vi "Main.vi"() -> ()   [LabVIEW 2018]
uses:
  <vilib>/picture/picture.llb/imagedata.ctl
  <vilib>/Utility/miscctls.llb/LVPoint32TypeDef.ctl
  <vilib>/Utility/miscctls.llb/LVMouseTypeDef.ctl
  <vilib>/Utility/miscctls.llb/LVPositionTypeDef.ctl
  <vilib>/Utility/miscctls.llb/LVPointTypeDef.ctl
  <vilib>/Utility/miscctls.llb/LVRectTypeDef.ctl
  Shared Variables/Alarm Cluster (UI).ctl
  Shared Variables/Alarm Cluster.ctl
  Drag and Drop/State Cluster.ctl
  support/Message Queue/Message Cluster.ctl
  Drag and Drop/Thumbnail Cluster.ctl
  Drag and Drop/Object Cluster.ctl
  Drag and Drop/Object Type Enum.ctl
  Config Module/Controls/Main Config Cluster.ctl
  OPC/OPC Module Config.ctl
  Scale Module Folder/Measure Instrument/State Enum.ctl
  OPC/OPC Settings.ctl
  OPC/Variable Data Cluster.ctl
  <vilib>/OPCUA/controls/NodeId.ctl
  <vilib>/OPCUA/controls/OPC UA StatusCode.ctl
  <vilib>/OPCUA/controls/Subscription ID.ctl
  <vilib>/OPCUA/controls/OPC UA Client Refnum.ctl
  <vilib>/OPCUA/controls/Subscription Data Change.ctl
  <vilib>/OPCUA/controls/Data Type.ctl
  Feed Module/Controls/Feed Module Config Cluster.ctl
  Feed Module/Controls/Feed Module Settings Cluster.ctl
  Ismatec ISM 831C/Controls/Ismatech Settings Cluster.ctl
  Masterflex 7550-30/Controls/Settings Cluster.ctl
  Mettler Toledo/Controls/Settings Cluster.ctl
  Bronkhorst M13 Flow Meter/Settings Cluster.ctl
  Measure Instrument/PID 2 Parameters Cluster.ctl
  Measure Instrument/PID Input Enum.ctl
  Measure Instrument/PID 2 Output Enum.ctl
  Tacmina QI/Tacmina QI DAQ Setting.ctl
  KNF Pump/Settings Cluster plus SIMDOS.ctl
  ASIA Pump/Pump Settings.ctl
  VICI M50 Party Mode/Settings Cluster.ctl
  FLOM Pump/Settings Cluster.ctl
  SSI PR Class/SSI PR or LD Settings Cluster.ctl
  Masterflex 75211/Masterflex 75211 DAQ Setting.ctl
  SSI PR Class/SSI P40 Settings Cluster.ctl
  TT Module/Controls/TT Module Config Cluster.ctl
  Tag VIs/Numeric Alarm Settings Cluster.ctl
  Acquisition/Hardware Configuration.ctl
  Acquisition/Task Cluster.ctl
  PT Module/Controls/PT Module Config Cluster.ctl
  Scale Module Folder/Feed Module/Controls/Scale Module Config Cluster.ctl
  Scale Module Folder/Feed Module/Controls/Scale Module Settings Cluster.ctl
  Pump Module Folder/Pump Module Config Cluster.ctl
  Pump Module Folder/Pump Module Settings Cluster.ctl
  LabJack Module/Controls/U3 Module Config Cluster.ctl
  Decoration Module/Decoration Module Config Cluster.ctl
  Flow Module Folder/Feed Module/Controls/Flow Module Config Cluster.ctl
  Flow Module Folder/Feed Module/Controls/Flow Module Settings Cluster.ctl
  TCU Module/TCU Module Folder/TCU Module Config Cluster.ctl
  TCU Module/TCU Module Folder/TCU Module Settings Cluster.ctl
  TCU Module/TCU Module Folder/Measure Instrument/Output Devices.ctl
  Huber TCU/Huber Settings.ctl
  Lauda Integral XT-150 TCU/Lauda Settings.ctl
  Julabo Type 1 TCU/Julabo Type 1 TCU Folder/Julabo FP-50 Settings.ctl
  Huber Unistat 410 TCU/Huber Unistat 410 RS485 Settings.ctl
  D-O Module Folder/Not Sure Where this is Used.ctl
  Sequencing/Squence Control.ctl
  D-O Module Folder/D-O Module Config Cluster.ctl
  D-O Module Folder/Valve Clusters.ctl
  D-O Module Folder/D-O Module Settings Cluster.ctl
  D-O Module Folder/D-O Device Settings Cluster.ctl
  VICI Electronic Actuator/VICI Electronic Actuator Settings.ctl
  Pressure Regulator Control Module/Pressure Regulator/Controls/4-20mA Module Config Cluster.ctl
  Pressure Regulator Control Module/Pressure Regulator/Controls/4-20mA Module Settings Cluster.ctl
  Pressure Transmitter/Pressure Transmitter Device Settings.ctl
  Pressure Reg Module/Pressure Regulator Device Settings.ctl
  Tag VIs/Tag FGV Operation Enum.ctl
  Shared Variables/Alarm Log Operation Enum.ctl
  Drag and Drop/Drop Parameters Cluster.ctl
  Drag and Drop/Module Instance Number Operation Enum.ctl
  Drag and Drop/Module Type Enum.ctl
  <vilib>/Utility/error.llb/DialogType.ctl
  Config Module/Controls/Config File Operation Enum.ctl
  Waveform Loop/Start Params Cluster.ctl
  Pump Calibration Program/Pump Calibration Config.ctl
  support/Message Queue/Enqueue Message (Single).vi
  <vilib>/Utility/cursorutil.llb/Set Cursor (Icon Pict).vi
  Main/Main Globals.vi
  LabJack Module/U3 (Main).vit
  D-O Module Folder/D-O Module (Main).vi
  TCU Module/TCU Module Folder/TCU Module (Main).vi
  Flow Module Folder/Flow Module (Main).vi
  <vilib>/Utility/cursorutil.llb/Set Cursor (Cursor ID).vi
  support/Message Queue/Message Queue.lvlib
  support/User Event - Stop/User Event - Stop.lvlib
  support/Support Library.lvlib
  Drag and Drop/Drag and Drop.lvlib
  Feed Module/Feed Module.lvlib
  TT Module/TT Module.lvlib
  History Graph/History Graph.lvlib
  Waveform Loop/Waveform Loop.lvlib
  CSV Log/CSV Log.lvlib
  TDMS Log/TDMS Log.lvlib
  Shared Variables/Dynamic Shared Variables.lvlib
  DAQ/DAQ.lvlib
  Config Module/Config Module.lvlib
  Bronkhorst M13 Flow Meter/Bronkhorst M13 Flow Meter.lvlib
  Mettler Toledo/Mettler Toledo.lvlib
  Masterflex 7550-30/Masterflex 7550-30.lvlib
  Ismatec ISM 831C/Ismatec ISM 831C.lvlib
  PT Module/PT Module.lvlib
  Scale Module Folder/Scale Module.lvlib
  Pump Module Folder/Pump Module.lvlib
  <vilib>/lvdsc/NI_DSC.lvlib
  LabJack Module/U3 Module.lvlib
  Flow Module Folder/Flow Module.lvlib
  Tacmina QI/Tacmina QI.lvlib
  KNF Pump/KNF SIMDOS.lvlib
  Huber TCU/Huber Ministat 230 TCU.lvlib
  TCU Module/TCU Module Folder/TCU Module.lvlib
  Lauda Integral XT-150 TCU/Lauda TCU.lvlib
  Julabo Type 1 TCU/Julabo Type 1 TCU Folder/Julabo Type FP-50 TCU.lvlib
  ASIA Pump.lvlib
  Sequencing/Sequencing Library.lvlib
  VICI M50 Party Mode/VICI M6 M50 Party Mode.lvlib
  D-O Module Folder/D-O Module.lvlib
  Pressure Regulator Control Module/Pressure Regulator/4-20mA Module.lvlib
  Pressure Reg Module/Pressure Regulator Library.lvlib
  Pressure Transmitter/Pressure Transmitter Library.lvlib
  FLOM Pump/FLOM Pump.lvlib
  support/Command Log VIs/Command Logging.lvlib
  Calibration VIs/Calibration.lvlib
  Lauda Integral XT-150 TCU/TCP Library.lvlib
  SSI PR Class/SSI PR or LD Pump.lvlib
  Scale Module Folder/Measure Instrument/Scale Module Engine.lvlib
  OPC/OPC UA.lvlib
  D-O Module Folder/DIO Valve/VICI Electronic Actuator.lvlib
  subVIs/Main SubVIs.lvlib
  Masterflex 75211/Masterflex 75211.lvlib
  SSI PR Class/SSI P40 Pump.lvlib
  Huber Unistat 410 TCU/Huber Unistat 410 TCU.lvlib
panel:
  out "Cluster":T1 {"Main Config"."PR Module Configs"."Settings"."PID 2 Parameters"."output range"."output low" format="%.2f"; "Main Config"."PR Module Configs"."Settings"."PID 2 Parameters"."output range"."output high" min=0.0 max=100.0 format="%.2f"; "Main Config"."PR Module Configs"."Settings"."PID 2 Parameters"."PID gains"."derivative time (Td, min)" format="%.3f"; "Main Config"."PR Module Configs"."Settings"."PID 2 Parameters"."PID gains"."integral time (Ti, min)" format="%.3f"; "Main Config"."PR Module Configs"."Settings"."PID 2 Parameters"."PID gains"."proportional gain (Kc)" format="%.3f"; "Main Config"."Steps"."Control" items=["Pump %", "Setpoint"]; "Main Config"."TCU Module Configs"."Settings"."Huber Unistat 410 Settings"."Address" min=0 max=99 format="%02.0f"; "Main Config"."TCU Module Configs"."Settings"."Julabo FP-50 Settings"."Pump Power" min=0 max=8 step=1; "Main Config"."TCU Module Configs"."Settings"."Lauda Settings"."Pump Power" min=0 max=8 step=1; "Main Config"."Pump Module Configs"."Settings"."ASIA Pump C"."channel" min=0 max=1 step=1; "Main Config"."Pump Module Configs"."Settings"."Masterflex"."Pump Number" min=1.0 max=20.0 step=1.0; "Main Config"."Pump Module Configs"."Settings"."Ismatech"."Pump Number" min=1.0 max=20.0 step=1.0; "Main Config"."Feed Module Configs"."Settings"."output range"."output low" min=0.0 max=100.0 format="%.2f"; "Main Config"."Feed Module Configs"."Settings"."output range"."output high" format="%.2f"; "Main Config"."Feed Module Configs"."Settings"."PID 2 Parameters"."PID gains"."derivative time (Td, min)" format="%.3f"; "Main Config"."Feed Module Configs"."Settings"."PID 2 Parameters"."PID gains"."integral time (Ti, min)" format="%.3f"; "Main Config"."Feed Module Configs"."Settings"."PID 2 Parameters"."PID gains"."proportional gain (Kc)" format="%.3f"; "Main Config"."Feed Module Configs"."Settings"."ASIA Pump C"."channel" min=0 max=1 step=1; "Main Config"."Feed Module Configs"."Settings"."Ismatech"."Pump Number" min=1.0 max=20.0 step=1.0; "Main Config"."Feed Module Configs"."Settings"."Masterflex"."Pump Number" min=1.0 max=20.0 step=1.0}
  in  "Alarm History Button":bool
  out "Alarm Model":T65[](array[typedef]) {"Alarm"."value" format="%.2f"; "Alarm"."setpoint" format="%.2f"; "Alarm"."clear time" format="%<%X\n%x>T"; "Alarm"."ack time" format="%<%X\n%x>T"; "Alarm"."set time" format="%<%X\n%x>T"}
  in  "UI Alarms":T66[](array[typedef])
  out "Message Data":variant
  out "data":errorcluster
  in  "End Program":bool
  out "CSV Log File":path
  out "error out":errorcluster
  in  "E-Stop":bool
  out "x-y":T4
  out "Front Panel Window:Panel Bounds":T4
  out "Drop Offset":T6
  out "Origin":T67
  out "Position":T6
  out "output cluster":cluster{"Coords":T10, "Mouse":T68}
  out "Mouse Position":cluster{"X":i32, "Y":i32}
  out "Path":path
  out "index of element":i32
  out "image data":T69
  in  "Page":string="Batch"
  in  "Notebook":string="Test"
  in  "Exit":bool
  in  "Settings":bool
  in  "Pause Log Button":bool
  in  "Force Trigger":bool
  in  "Start Log":bool
  out "Canvas":picture
  out "Palette":picture
  in  "?":T1 {"Main Config"."PR Module Configs"."Settings"."PID 2 Parameters"."output range"."output low" format="%.2f"; "Main Config"."PR Module Configs"."Settings"."PID 2 Parameters"."output range"."output high" min=0.0 max=100.0 format="%.2f"; "Main Config"."PR Module Configs"."Settings"."PID 2 Parameters"."PID gains"."derivative time (Td, min)" format="%.3f"; "Main Config"."PR Module Configs"."Settings"."PID 2 Parameters"."PID gains"."integral time (Ti, min)" format="%.3f"; "Main Config"."PR Module Configs"."Settings"."PID 2 Parameters"."PID gains"."proportional gain (Kc)" format="%.3f"; "Main Config"."Steps"."Control" items=["Pump %", "Setpoint"]; "Main Config"."TCU Module Configs"."Settings"."Huber Unistat 410 Settings"."Address" min=0 max=99 format="%02.0f"; "Main Config"."TCU Module Configs"."Settings"."Julabo FP-50 Settings"."Pump Power" min=0 max=8 step=1; "Main Config"."TCU Module Configs"."Settings"."Lauda Settings"."Pump Power" min=0 max=8 step=1; "Main Config"."Pump Module Configs"."Settings"."ASIA Pump C"."channel" min=0 max=1 step=1; "Main Config"."Pump Module Configs"."Settings"."Masterflex"."Pump Number" min=1.0 max=20.0 step=1.0; "Main Config"."Pump Module Configs"."Settings"."Ismatech"."Pump Number" min=1.0 max=20.0 step=1.0; "Main Config"."Feed Module Configs"."Settings"."output range"."output low" min=0.0 max=100.0 format="%.2f"; "Main Config"."Feed Module Configs"."Settings"."output range"."output high" format="%.2f"; "Main Config"."Feed Module Configs"."Settings"."PID 2 Parameters"."PID gains"."derivative time (Td, min)" format="%.3f"; "Main Config"."Feed Module Configs"."Settings"."PID 2 Parameters"."PID gains"."integral time (Ti, min)" format="%.3f"; "Main Config"."Feed Module Configs"."Settings"."PID 2 Parameters"."PID gains"."proportional gain (Kc)" format="%.3f"; "Main Config"."Feed Module Configs"."Settings"."ASIA Pump C"."channel" min=0 max=1 step=1; "Main Config"."Feed Module Configs"."Settings"."Ismatech"."Pump Number" min=1.0 max=20.0 step=1.0; "Main Config"."Feed Module Configs"."Settings"."Masterflex"."Pump Number" min=1.0 max=20.0 step=1.0}
  # "little pump\ncentrifigual pump\nflow rate\npressure\nS or P to the left\nsolvent or process"
  # "Question: how do we make the live VI, such as the feed module graphic\nsized right for the picture that is loaded?\n\nProbably should standarize each module size. Then the  flow sheet\ndrawings will all just match the size and we don't have to worry about\nscale."
  # "vertical or horizontal lines\nextendable"
  # "Tasks\n1. Load graphic\n2. Drag and drop onto picture control\n3. Picture control draws hot spot\n4. If drag and drop on picture control, then resize and redraw the nearest hotspot\n5. When operator turns \"ON\" the system, then the hotspots are replaced with actual VIs."
  # "as much drawing room as possible"
  # "Instrument Settings"
  # "Instrument Settings"
  # "Output Instruments"
  # "Flow Meter Settings"
  # "Output Instruments"
  # "Scale Settings"
  # "Output Instruments"
  # "Input Instruments"
  # "Instrument Settings"
  # "Instrument Settings"
  # "Output Instruments"
  # "Flow Meter Settings"
  # "Output Instruments"
  # "Scale Settings"
  # "Output Instruments"
  # "Input Instruments"
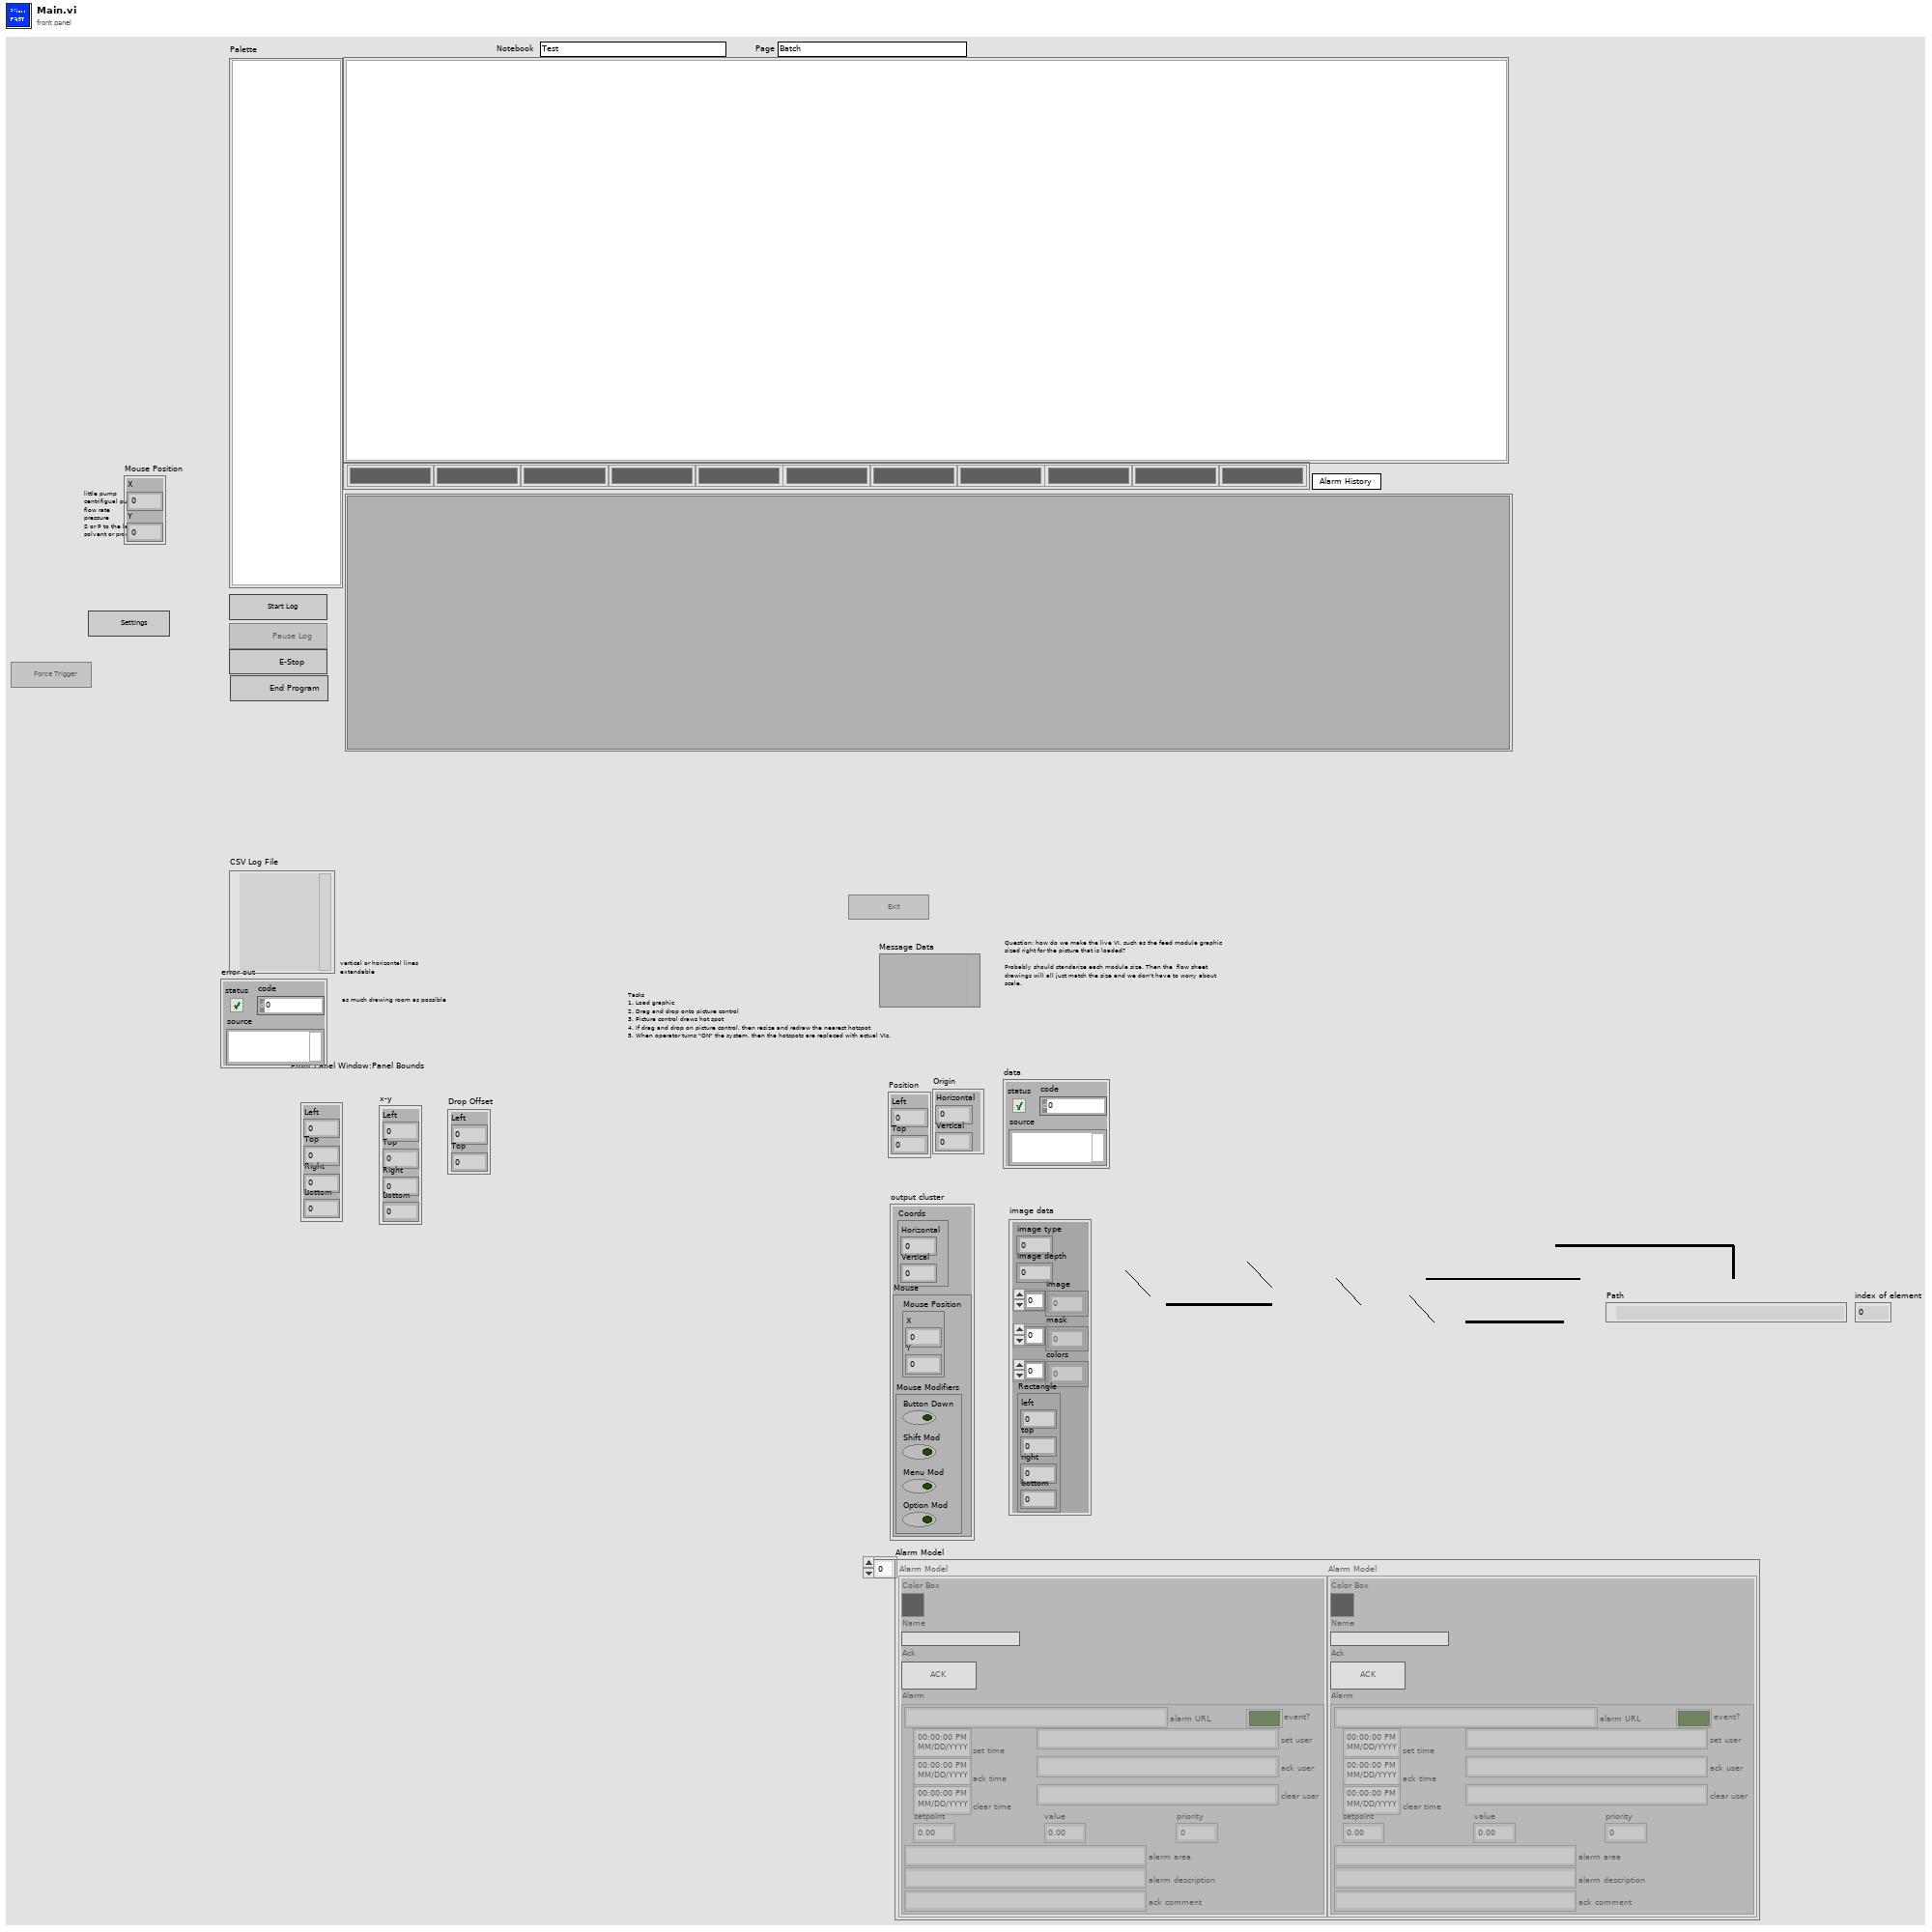
[diagram p1: front panel]
types:
  T1 = typedef "Drag and Drop.lvlib/State Cluster.ctl" = cluster{"VI refs":refnum<vi>[], "Queues":refnum<queue>[], "[Thumbnails]":T2[], "Drag Object Idx":i32, "[Objects]":T3[], "Active Object":i32, "Drop Offset":T6, "Process Name":string, "Main Config":T7, "Campaign Filepath":path, "Config Changed?":bool}
  T2 = typedef "Thumbnail Cluster.ctl" = cluster{"Path":path, "Rectangle":cluster{"left":i16, "top":i16, "right":i16, "bottom":i16}}
  T3 = typedef "Object Cluster.ctl" = cluster{"BMP Path":path, "Anchor Position":cluster{"X":i32, "Y":i32}, "Hot Spot":T4, "Type":T5, "Parameters":variant}
  T4 = typedef "LVRectTypeDef.ctl" = cluster{"Left":i16, "Top":i16, "Right":i16, "Bottom":i16}
  T5 = typedef "Object Type Enum.ctl" = enum16{"Icon", "Line", "Text", "Feed Module"}
  T6 = typedef "LVPositionTypeDef.ctl" = cluster{"Left":i32, "Top":i32}
  T7 = typedef "Config Module.lvlib/Main Config Cluster.ctl" = cluster{"Notebook":string, "Page":string, "OPC Module Configs":T8[], "Feed Module Configs":T17[], "Log File Path":path, "TT Module Configs":T34[], "DAQ Config":T36, "PT Module Configs":T38[], "Scale Module Configs":T39[], "Pump Module Configs":T41[], "U3 Module Configs":T43[], "Decoration Module Configs":T44[], "Flow Module Configs":T45[], "TCU Module Configs":T47[], "Steps":T54, "Abort":bool, "DO Module Configs":T56[], "PR Module Configs":T61[], "Cycle Period":dbl}
  T8 = typedef "OPC UA.lvlib/OPC Module Config.ctl" = cluster{"State":T9, "GUID":string, "Drop Coords":T10, "Configuration":T11, "First Iteration":bool, "Data":cluster{"Object Name":string, "Variable Array":T12[]}[], "Process Name":string, "Load Count":i32, "Log Started":bool, "subscription ID out":T15, "OPC UA client refnum out":T16, "Event Registration Refnum":refnum<event-registration>, "Start Time":timestamp, "Current Time":timestamp}
  T9 = typedef "Scale Module.lvlib/Scale Module Engine.lvlib/State Enum.ctl" = enum16{"Measuring", "Idle"}
  T10 = typedef "LVPoint32TypeDef.ctl" = cluster{"Horizontal":i32, "Vertical":i32}
  T11 = typedef "OPC UA.lvlib/OPC Settings.ctl" = cluster{"Cycle Period":dbl, "server endpoint URL":string, "security policy":cluster{"message mode":enum16{"None", "Sign", "Sign and Encrypt"}, "security":enum16{"Basic256", "Basic128Rsa15"}}, "Trust Any Server":bool}
  T12 = typedef "OPC UA.lvlib/Variable Data Cluster.ctl" = cluster{"node ID":T13, "browse name":string, "status":T14, "timestamp":timestamp, "value ":variant}
  T13 = typedef "NodeId.ctl" = string
  T14 = typedef "OPC UA StatusCode.ctl" = u32
  T15 = typedef "Subscription ID.ctl" = u32
  T16 = typedef "OPC UA Client Refnum.ctl" = refnum<k21>
  T17 = typedef "Feed Module.lvlib/Feed Module Config Cluster.ctl" = cluster{"GUID":string, "Drop Coords":T10, "Process Name":string, "Queue Name":string, "Settings":T18, "Settings Load Count":i32, "OP Load Count":i32}
  T18 = typedef "Feed Module.lvlib/Feed Module Settings Cluster.ctl" = cluster{"Cycle Period":dbl, "Ismatech":T19, "Masterflex":T20, "Mettler":T21, "Bronkhorst M13 Flow Meter":T22, "PID 2 Parameters":T23, "Manual Entry":dbl, "Auto?":bool, "output range":cluster{"output high":dbl, "output low":dbl}, "Bronkhorst M14":T21, "Tacmina Settings":T26, "KNF SIMDOS Settings":T27, "ASIA Pump C":T28, "VICI Settings":T29, "FLOM Settings":T30, "SSI PR/LD Settings":T31, "Masterflex 75211 Settings":T32, "SSI P40 Settings":T33}
  T19 = typedef "Ismatec ISM 831C.lvlib/Ismatech Settings Cluster.ctl" = cluster{"VISA resource name":refnum<visa-resource-name>, "Simulated?":bool, "Pump Number":dbl, "Reverse?":bool}
  T20 = typedef "Masterflex 7550-30.lvlib/Settings Cluster.ctl" = cluster{"VISA resource name":refnum<visa-resource-name>, "Simulated?":bool, "Pump Number":dbl, "Reverse?":bool}
  T21 = typedef "Mettler Toledo.lvlib/Settings Cluster.ctl" = cluster{"VISA resource name":refnum<visa-resource-name>, "Simulated?":bool}
  T22 = typedef "Bronkhorst M13 Flow Meter.lvlib/Settings Cluster.ctl" = cluster{"VISA resource name":refnum<visa-resource-name>, "Simulated?":bool}
  T23 = typedef "PID 2 Parameters Cluster.ctl" = cluster{"Input Device":T24, "Output Device":T25, "Setpoint":dbl, "PID gains":cluster{"proportional gain (Kc)":dbl, "integral time (Ti, min)":dbl, "derivative time (Td, min)":dbl}}
  T24 = typedef "PID Input Enum.ctl" = enum16{"Default", "Bronkhorst M13", "Bronkhorst M14", "Scale Rate of Change"}
  T25 = typedef "PID 2 Output Enum.ctl" = enum16{"Default", "Ismatec ISM 831C", "Masterflex 7550-30", "VICI", "Tacmina QI", "KNF SIMDOS", "ASIA Type C", "FLOM UI-22-11", "SSI PR/LD", "SSI P40", "Masterflex 75211-70"}
  T26 = typedef "Tacmina QI.lvlib/Tacmina QI DAQ Setting.ctl" = cluster{"Analog DAQ Task":refnum<k21>, "Digital DAQ Task":refnum<k21>}
  T27 = typedef "KNF SIMDOS.lvlib/Settings Cluster plus SIMDOS.ctl" = cluster{"VISA resource name":refnum<visa-resource-name>, "Simulated?":bool}
  T28 = typedef "ASIA Pump.lvlib/Pump Settings.ctl" = cluster{"ASIA Pump #":i32, "channel":i32, "Simulated":bool}
  T29 = typedef "VICI M6 M50 Party Mode.lvlib/Settings Cluster.ctl" = cluster{"VISA resource name":refnum<visa-resource-name>, "Simulated?":bool, "Pump Letter":string, "Reverse?":bool}
  T30 = typedef "FLOM Pump.lvlib/Settings Cluster.ctl" = cluster{"VISA resource name":refnum<visa-resource-name>, "Simulated?":bool, "Pump Number":dbl}
  T31 = typedef "SSI PR or LD Pump.lvlib/SSI PR or LD Settings Cluster.ctl" = cluster{"VISA resource name":refnum<visa-resource-name>, "Simulated?":bool}
  T32 = typedef "Masterflex 75211.lvlib/Masterflex 75211 DAQ Setting.ctl" = cluster{"Analog DAQ Task":refnum<k21>, "Digital DAQ Task":refnum<k21>}
  T33 = typedef "SSI P40 Pump.lvlib/SSI P40 Settings Cluster.ctl" = cluster{"VISA resource name":refnum<visa-resource-name>, "Simulated?":bool}
  T34 = typedef "TT Module.lvlib/TT Module Config Cluster.ctl" = cluster{"GUID":string, "Drop Coords":T10, "Input Channel Tag Name ":string, "Process Name":string, "Queue Name":string, "Input Channel Numeric Alarm Settings":T35[]}
  T35 = typedef "Numeric Alarm Settings Cluster.ctl" = cluster{"enable? (F)":bool, "name":string, "alarm type":enum16{"HI_HI", "HI", "LO", "LO_LO"}, "level/change":dbl, "deadband/time":dbl, "alarm delay":dbl, "priority":u32, "ack type":enum16{"Auto", "User", "None", "Each Occurrence"}, "area":string, "description":string, "log? (T)":bool}
  T36 = typedef "DAQ.lvlib/Hardware Configuration.ctl" = cluster{"Tasks":T37[]}
  T37 = typedef "Task Cluster.ctl" = cluster{"DAQmx Task":refnum<k21>, "Read-Write Radio":enum32{"Read", "Write"}}
  T38 = typedef "PT Module.lvlib/PT Module Config Cluster.ctl" = cluster{"GUID":string, "Drop Coords":T10, "Input Channel Tag Name ":string, "Process Name":string, "Queue Name":string, "Input Channel Numeric Alarm Settings":T35[]}
  T39 = typedef "Scale Module.lvlib/Scale Module Config Cluster.ctl" = cluster{"GUID":string, "Drop Coords":T10, "Process Name":string, "Queue Name":string, "Settings":T40, "Load Count":i32}
  T40 = typedef "Scale Module.lvlib/Scale Module Settings Cluster.ctl" = cluster{"Cycle Period":dbl, "Mettler":T21, "Scale Type":string}
  T41 = typedef "Pump Module.lvlib/Pump Module Config Cluster.ctl" = cluster{"GUID":string, "Drop Coords":T10, "Process Name":string, "Queue Name":string, "Settings":T42, "Load Count":i32}
  T42 = typedef "Pump Module.lvlib/Pump Module Settings Cluster.ctl" = cluster{"Cycle Period":dbl, "Manual Entry":dbl, "Output Device":T25, "Ismatech":T19, "Masterflex":T20, "VICI Settings":T29, "Tacmina Settings":T26, "KNF SIMDOS Settings":T27, "ASIA Pump C":T28, "FLOM Settings":T30, "SSI PR/LD Settings":T31, "SSI P40 Settings":T31, "Masterflex 75211 Settings":T32, "Pump Calibration File":path, "Calibration Slope":dbl, "Calibration Y Intercept":dbl, "Pump Cal Enum":u16}
  T43 = typedef "U3 Module.lvlib/U3 Module Config Cluster.ctl" = cluster{"GUID":string, "Drop Coords":T10, "AI Channel Number":enum16{"Default", "AI0", "AI1", "AI2", "AI3", "AI4", "AI5", "AI6", "AI7"}, "Process Name":string, "Queue Name":string, "Input Channel Numeric Alarm Settings":T35[]}
  T44 = typedef "Decoration Module Config Cluster.ctl" = cluster{"GUID":string, "Drop Coords":T10, "Decoration Filepath":path}
  T45 = typedef "Flow Module.lvlib/Flow Module Config Cluster.ctl" = cluster{"GUID":string, "Drop Coords":T10, "Process Name":string, "Queue Name":string, "Settings":T46, "Load Count":i32}
  T46 = typedef "Flow Module.lvlib/Flow Module Settings Cluster.ctl" = cluster{"Cycle Period":dbl, "Bronkhorst M13":T21, "Flow Meter Type":string, "Bronkhorst M14":T21}
  T47 = typedef "TCU Module.lvlib/TCU Module Config Cluster.ctl" = cluster{"GUID":string, "Drop Coords":T10, "Process Name":string, "Queue Name":string, "Settings":T48, "Load Count":i32, "Power Level Changed":bool}
  T48 = typedef "TCU Module.lvlib/TCU Module Settings Cluster.ctl" = cluster{"Cycle Period":dbl, "Setpoint Entry":dbl, "Output Device":T49, "Huber Ministat 230 Settings":T50, "Lauda Settings":T51, "Julabo FP-50 Settings":T52, "Internal Control?":bool, "Huber Unistat 410 Settings":T53}
  T49 = typedef "Output Devices.ctl" = enum16{"Default", "Huber Ministat 230", "Huber Unistat 410", "Lauda XT-150", "Julabo FP-50"}
  T50 = typedef "Huber Ministat 230 TCU.lvlib/Huber Settings.ctl" = cluster{"VISA resource name":refnum<visa-resource-name>, "Simulated?":bool}
  T51 = typedef "Lauda TCU.lvlib/Lauda Settings.ctl" = cluster{"VISA resource name":refnum<visa-resource-name>, "Simulated?":bool, "Pump Power":i32}
  T52 = typedef "Julabo Type FP-50 TCU.lvlib/Julabo FP-50 Settings.ctl" = cluster{"VISA resource name":refnum<visa-resource-name>, "Simulated?":bool, "Pump Power":i32}
  T53 = typedef "Huber Unistat 410 TCU.lvlib/Huber Unistat 410 RS485 Settings.ctl" = cluster{"VISA resource name":refnum<visa-resource-name>, "Address":i8, "Simulated?":bool}
  T54 = typedef "Not Sure Where this is Used.ctl" = T55[]
  T55 = typedef "Sequencing Library.lvlib/Squence Control.ctl" = cluster{"Module":string, "Control":u16, "Value":dbl, "Wait (sec)":dbl}
  T56 = typedef "D-O Module.lvlib/D-O Module Config Cluster.ctl" = cluster{"GUID":string, "Drop Coords":T10, "Process Name":string, "Queue Name":string, "Settings":T57, "Load Count":i32}
  T57 = typedef "D-O Module.lvlib/Valve Clusters.ctl" = cluster{"Valve Settings":T58, "Valve Type":enum16{"Default", "Digital Output Valve", "VICI Electronic Actuator"}, "Time On (Sec)":dbl, "Time Off (Sec)":dbl, "Run?":bool}
  T58 = typedef "D-O Module.lvlib/D-O Module Settings Cluster.ctl" = cluster{"D-O Settings":T59, "VICI Electronic Actuator":T60}
  T59 = typedef "D-O Module.lvlib/D-O Device Settings Cluster.ctl" = cluster{"DAQmx Task Name":refnum<k21>, "Output Channel":u16, "Output Channel Names":string[]}
  T60 = typedef "VICI Electronic Actuator.lvlib/VICI Electronic Actuator Settings.ctl" = cluster{"VISA resource name":refnum<visa-resource-name>, "Mode":enum16{"Two Positions With Stops", "Two Positions Without Stops", "Mutiposition"}, "Simulated":bool}
  T61 = typedef "4-20mA Module.lvlib/4-20mA Module Config Cluster.ctl" = cluster{"GUID":string, "Drop Coords":T10, "Process Name":string, "Queue Name":string, "Settings":T62, "Settings Load Count":i32}
  T62 = typedef "4-20mA Module.lvlib/4-20mA Module Settings Cluster.ctl" = cluster{"Cycle Period":dbl, "PID 2 Parameters":cluster{"Input Device":enum16{"Default", "4-20mA"}, "Output Device":enum16{"Default", "Equilibar Pressure Reg", "Flow Regulator"}, "Setpoint":dbl, "PID gains":cluster{"proportional gain (Kc)":dbl, "integral time (Ti, min)":dbl, "derivative time (Td, min)":dbl}, "output range":cluster{"output low":dbl, "output high":dbl}}, "Manual Entry":dbl, "Auto?":bool, "4-20mA Input Settings":T63, "4-20mA Out Settings":T64, "Input Channel Tag Name ":string}
  T63 = typedef "Pressure Transmitter Library.lvlib/Pressure Transmitter Device Settings.ctl" = cluster{"Input Channel ":u16}
  T64 = typedef "Pressure Regulator Library.lvlib/Pressure Regulator Device Settings.ctl" = cluster{"Output DAQ Task":refnum<k21>}
  T65 = typedef "Dynamic Shared Variables.lvlib/Alarm Cluster.ctl" = cluster{"Color Box":u32, "Name":string, "Ack":bool, "Alarm":cluster{"alarm URL":string, "set time":timestamp, "set user":string, "ack time":timestamp, "ack user":string, "clear time":timestamp, "clear user":string, "setpoint":dbl, "value":dbl, "priority":u32, "alarm area":string, "alarm description":string, "ack comment":string, "event?":bool, "Refnum":u64}}
  T66 = typedef "Dynamic Shared Variables.lvlib/Alarm Cluster (UI).ctl" = cluster{"Color Box":u32, "Name":string, "Ack":bool}
  T67 = typedef "LVPointTypeDef.ctl" = cluster{"Horizontal":i16, "Vertical":i16}
  T68 = typedef "LVMouseTypeDef.ctl" = cluster{"Mouse Position":cluster{"X":i32, "Y":i32}, "Mouse Modifiers":cluster{"Button Down":bool, "Shift Mod":bool, "Menu Mod":bool, "Option Mod":bool}}
  T69 = typedef "imagedata.ctl" = cluster{"image type":i32, "image depth":i32, "image":u8[], "mask":u8[], "colors":u32[], "Rectangle":cluster{"left":i16, "top":i16, "right":i16, "bottom":i16}}
  T70 = typedef "Tag FGV Operation Enum.ctl" = enum16{"Init", "Set Notification Queue", "Create Tag", "Commit", "Write Tag (Numeric)", "Write Tag (Boolean)", "Read All Tags", "Read One Tag", "Delete Tag Category", "Set Alarm Parameters (Numeric)", "Set Alarm Parameters (Boolean)", "Enable All Alarms", "Disable All Alarms", "Delete All Tags", "Read Alarms", "Ack Alarm", "Read Alarm Parameters (Numeric)", "Read Alarm Parameters (Boolean)"}
  T71 = cluster{"Down":bool, "Mouse":T68, "Drag":bool, "Canvas":bool}
  T72 = cluster{"Busy":bool, "PumpCnt":dbl, "RemoteEntered":bool, "OverpressureSet":bool}[]
  T73 = typedef "Main Queue Cluster.ctl" = cluster{"UI":refnum<queue>, "Waveform Loop":refnum<queue>, "CSV Log":refnum<queue>, "TDMS Log":refnum<queue>, "Graphs":refnum<queue>[], "DAQ":refnum<queue>, "Sequence":refnum<queue>, "TCP Write":refnum<queue>, "Sequence UI":refnum<queue>, "OPC UA Log":refnum<queue>, "TCP Read":refnum<queue>}
  T74 = cluster{"Event Registration Refnum":refnum<event-registration>, "Stop Event Registration Refnum":refnum<event-registration>}
  T75 = typedef "Alarm Log Operation Enum.ctl" = enum16{"Create Log", "Log Alarm", "Close Log"}
  T76 = enum32{"Invalid", "Standard", "Closed", "Hidden", "Minimized", "Maximized"}
  T77 = enum8{"Enabled", "Disabled", "Disabled and Grayed Out"}
  T78 = cluster{"alarm URL":string, "set time":timestamp, "set user":string, "ack time":timestamp, "ack user":string, "clear time":timestamp, "clear user":string, "setpoint":dbl, "value":dbl, "priority":u32, "alarm area":string, "alarm description":string, "ack comment":string, "event?":bool, "Refnum":u64}[]
  T79 = cluster{"alarm URL":string, "set time":timestamp, "set user":string, "ack time":timestamp, "ack user":string, "clear time":timestamp, "clear user":string, "setpoint":dbl, "value":dbl, "priority":u32, "alarm area":string, "alarm description":string, "ack comment":string, "event?":bool, "Refnum":u64}
  T80 = typedef "Drag and Drop.lvlib/Module Type Enum.ctl" = enum16{"<unknown module>", "Feed", "TT", "PT", "Scale", "Flow", "Pump", "U3", "TCU", "DO", "PR", "OPC"}
  T81 = typedef "Module Instance Number Operation Enum.ctl" = enum16{"Init", "Next Instance Number"}
  T82 = typedef "Drop Parameters Cluster.ctl" = cluster{"Module VI Filepath":path, "Process Name":string, "Main UI Message Queue":refnum<queue>, "Drop Coords":T10, "Module Parameters":variant, "Name of Parent Window":string}
  T83 = typedef "Config Module.lvlib/Config File Operation Enum.ctl" = enum16{"Read", "Write"}
  T84 = typedef "Waveform Loop.lvlib/Start Params Cluster.ctl" = cluster{"dt (seconds)":dbl, "CSV Logfile path":path, "TDMS Logfile path":path}
  T85 = typedef "Calibration.lvlib/Pump Calibration Config.ctl" = cluster{"Settings":cluster{"Cycle Period":dbl, "Ismatech":T19, "Masterflex":T20, "Bronkhorst M13 Flow Meter":T22, "PID 2 Parameters":cluster{"Input Device":T24, "Output Device":T25}, "Bronkhorst M14":T21, "Tacmina Settings":T26, "KNF SIMDOS Settings":T27, "VICI M50 Settings":T29, "FLOM Settings":T30, "Calibration Limits":cluster{"Minimum (ml/min)":dbl, "Maximum (ml/min)":dbl, "Steps":dbl}, "SSI PR Settings":T31}, "Flowmeter Output":dbl, "Density":dbl, "FL Temp":dbl, "Speed %":dbl, "File Refnum":refnum<file>, "Pump On?":enum16{"Off", "On", "Not Initialized"}}
  T86 = typedef "DialogType.ctl" = u16
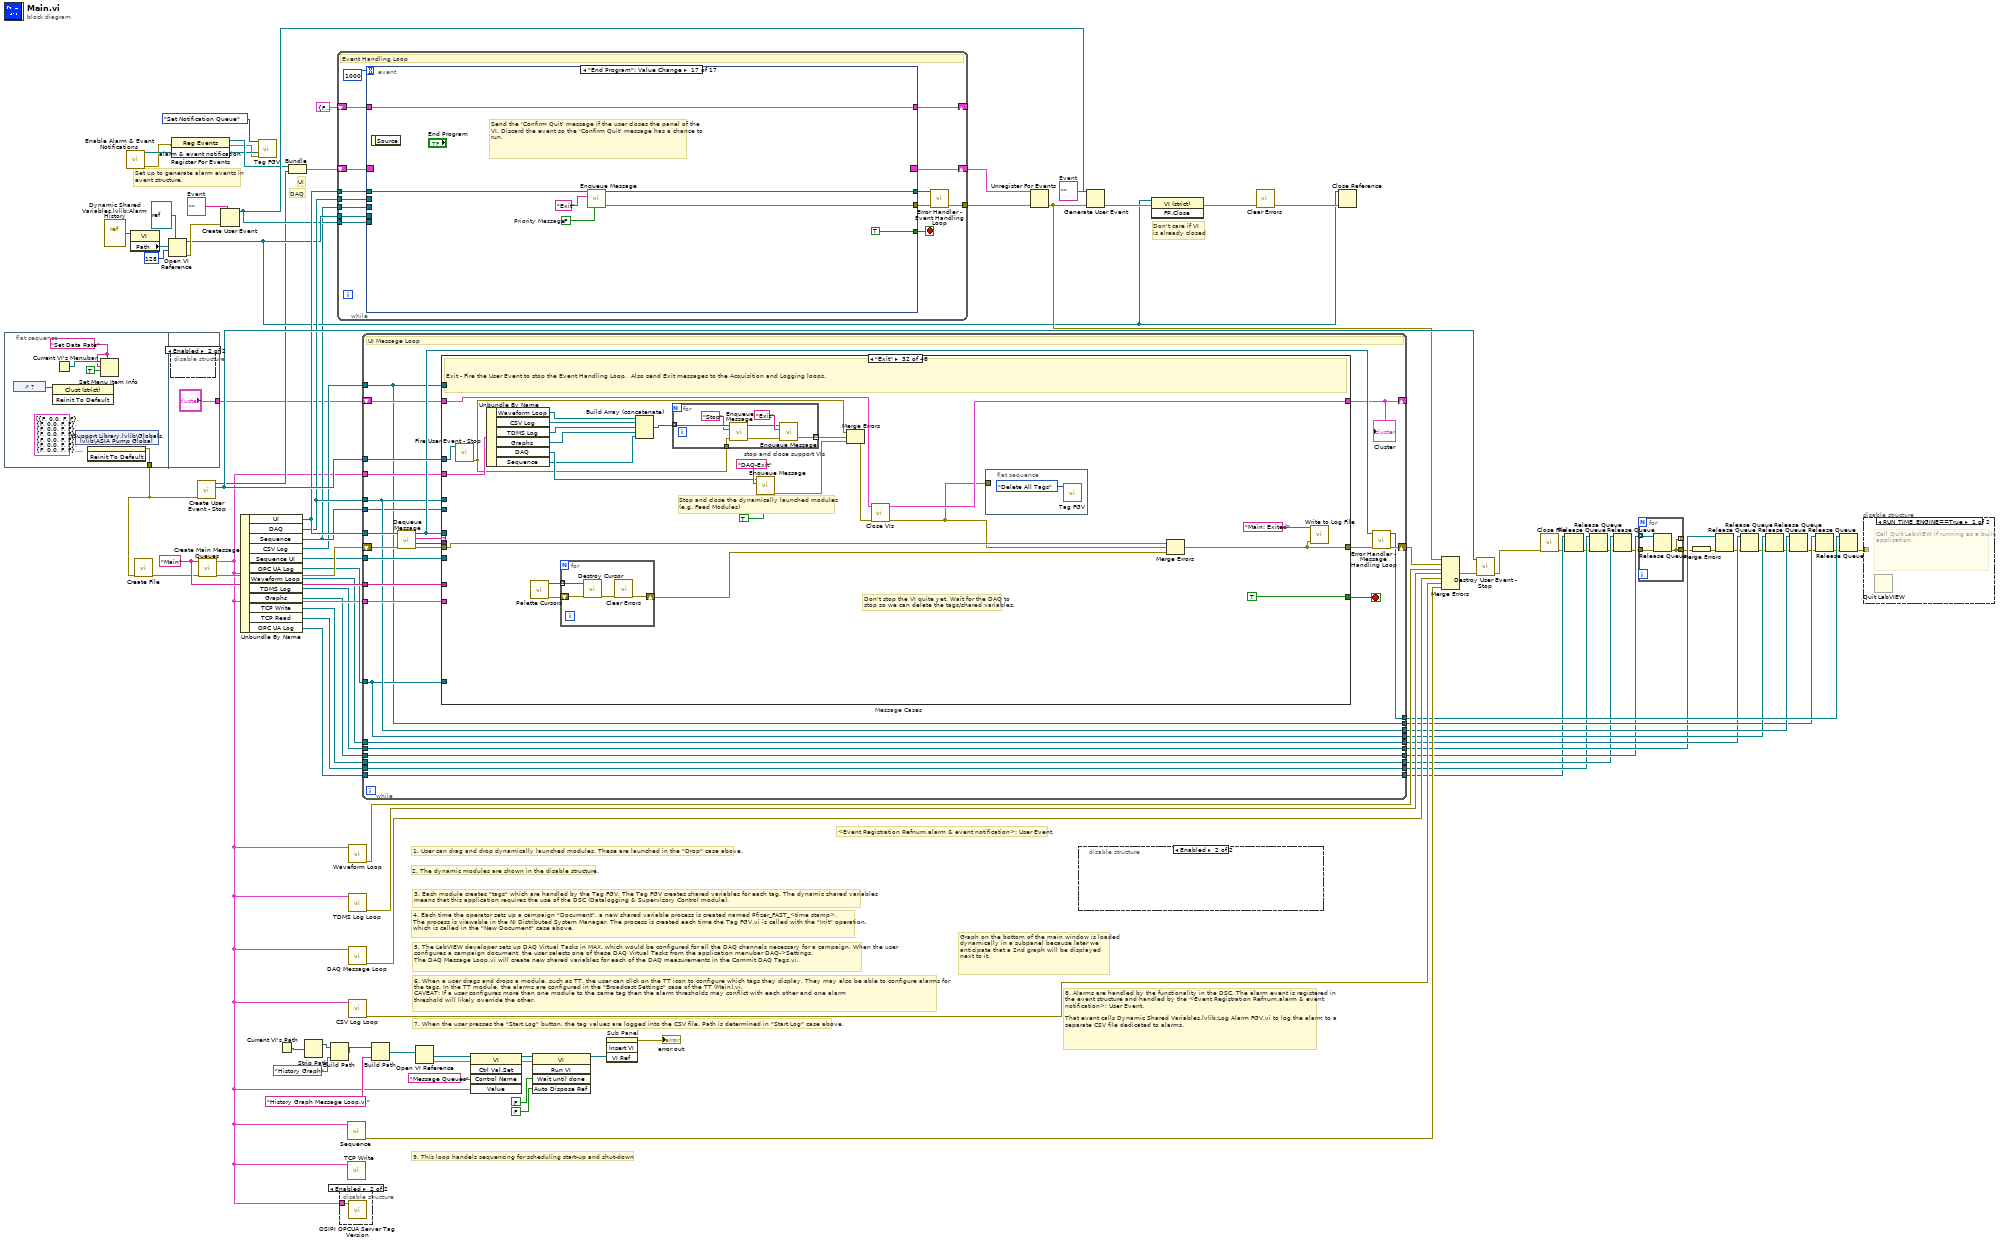
[diagram p0: block diagram]
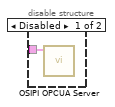
[diagram p2: hidden frame]
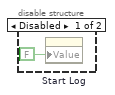
[diagram p3: hidden frame]
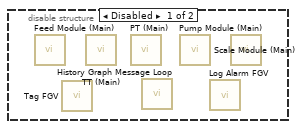
[diagram p5: hidden frame]
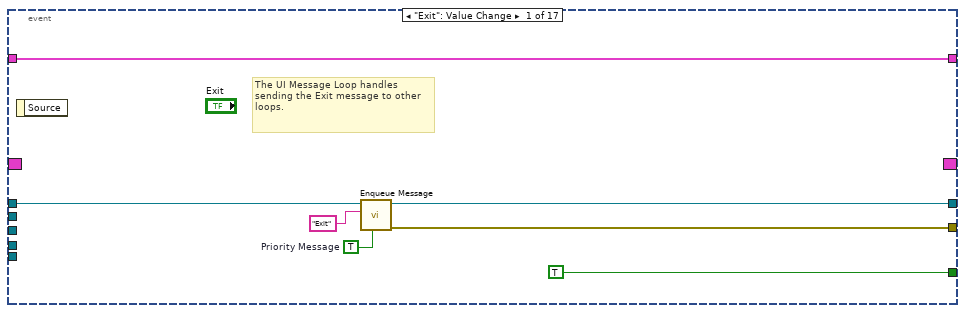
[diagram p6: hidden frame]
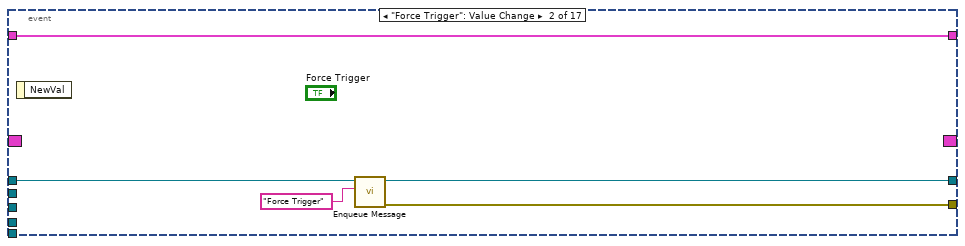
[diagram p7: hidden frame]
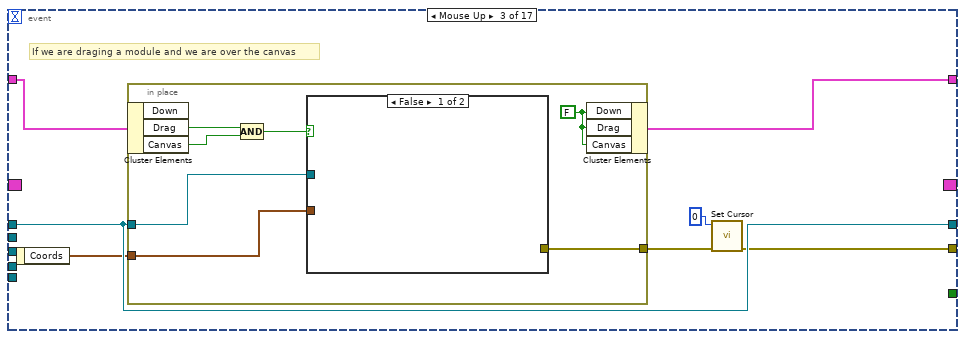
[diagram p8: hidden frame]
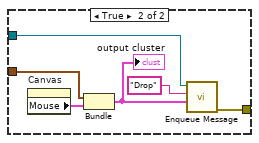
[diagram p9: hidden frame]
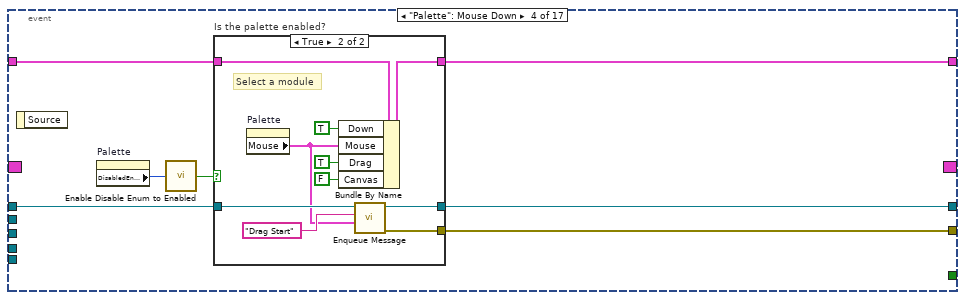
[diagram p10: hidden frame]
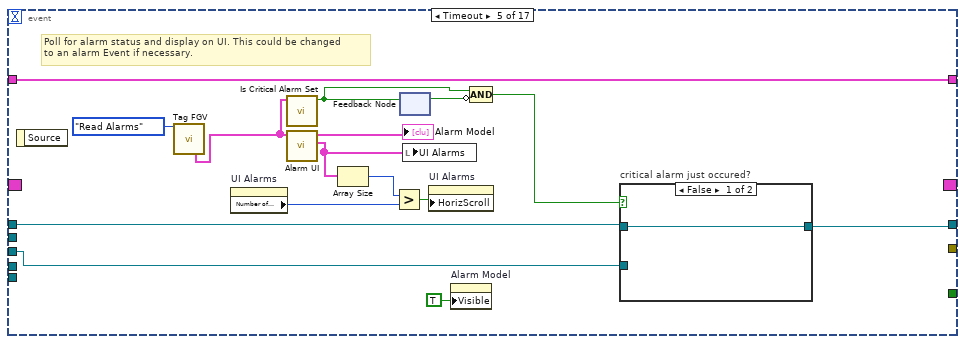
[diagram p12: hidden frame]
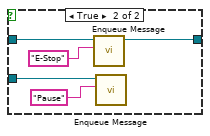
[diagram p13: hidden frame]
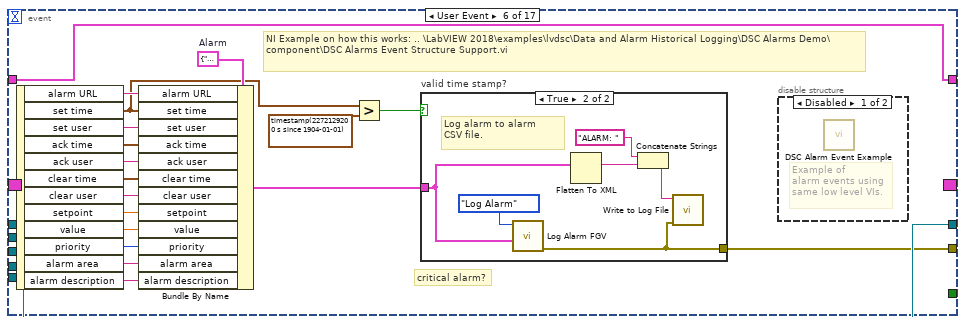
[diagram p14: hidden frame]
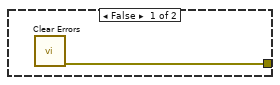
[diagram p16: hidden frame]
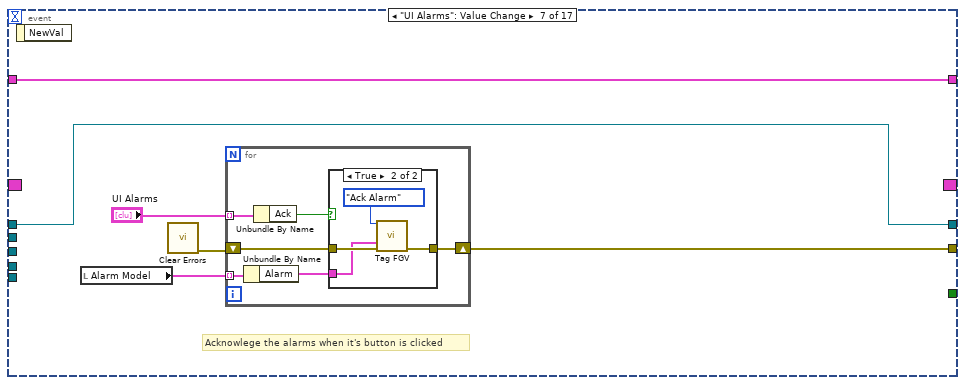
[diagram p17: hidden frame]
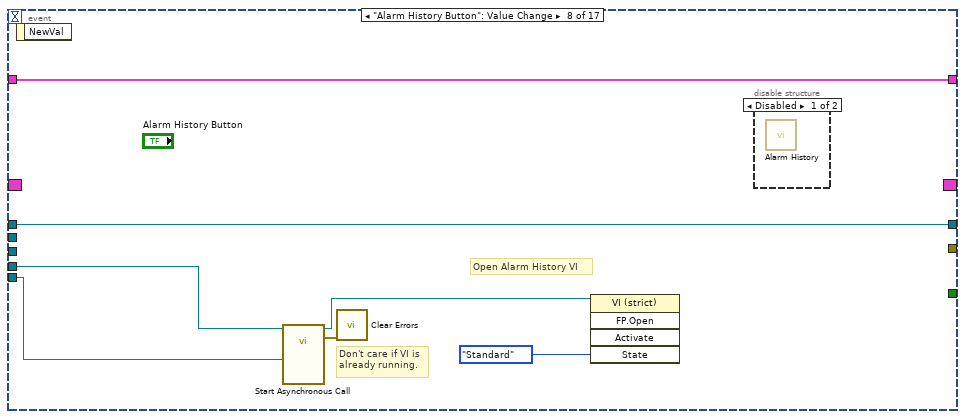
[diagram p19: hidden frame]
diagram:
  w50 = ""  # Event
  w57 = ""  # Event
  w80 = "Main" ("Process Name")
  # "<Event Registration Refnum.alarm & event notification>: User Event"
  # "9. This loop handels sequencing for scheduling start-up and shut-down"
  # "6. When a user drags and drops a module, such as TT, the user can click on the TT icon to configure which tags they display. They may also be able to configure alarms for\nthe tags. In the TT module, the alarms are configured in the \"Broadcast Settings\" case of the TT (Main).vi.\nCAVEAT: If a user configures more than one module to the same tag then the alarm thresholds may conflict with each other and one alarm\nthreshold will likely override the other."
  # "8. Alarms are handled by the functionality in the DSC. The alarm event is registered in the event structure and handled by the <Event Registration Refnum.alarm & event notification>: User Event.\n\nThat event calls Dynamic Shared Variables.lvlib:Log Alarm FGV.vi to log the alarm to a separate CSV file dedicated to alarms."
  # "Graph on the bottom of the main window is loaded dynamically in a subpanel because later we anticipate that a 2nd graph will be displayed\nnext to it."
  # "7. When the user presses the \"Start Log\" button, the tag values are logged into the CSV file. Path is determined in \"Start Log\" case above."
  # "5. The LabVIEW developer sets up DAQ Virtual Tasks in MAX, which would be configured for all the DAQ channels necessary for a campaign. When the user configures a campaign document, the user selects one of these DAQ Virtual Tasks from the application menubar DAQ->Settings.\nThe DAQ Message Loop.vi will create new shared variables for each of the DAQ measurements in the Commit DAQ Tags.vi."
  # "4. Each time the operator sets up a campaign \"Document\", a new shared variable process is created named Pfizer_FAST_<time stamp>.\nThe process is viewable in the NI Distributed System Manager. The process is created each time the Tag FGV.vi is called with the \"Init\" operation,\nwhich is called in the \"New Document\" case above."
  # "3. Each module creates \"tags\" which are handled by the Tag FGV. The Tag FGV creates shared variables for each tag. The dynamic shared variables\nmeans that this application requires the use of the DSC (Datalogging & Supervisory Control module)."
  # "2. The dynamic modules are shown in the disable structure."
  # "1. User can drag and drop dynamically launched modules. These are launched in the \"Drop\" case above."
  # "Set up to generate alarm events in\nevent structure."
  # "Don't care if VI\nis already closed"
  # "DAQ"
  # "UI"
  n1 = flat-sequence {
    tunnel: [w91] -> w39
    tunnel: ["?"] -> w40
    frame #0 {
      w89 = "Set Data Rate" ("item tag")
      n2 = control-ref of="?"() -> (w93:refnum<vi>)
      n3 = invoke class="Clust (strict)" method="Reinit To Default"(reference=w93) -> ()  [unwired: 2 in, 3 out]
      n4 = Current VI's Menubar() -> (w90:refnum<k9>)
      n5 = shared-variable ".\\Support Library.lvlib\\Globals.lvlib\\ASIA Pump Global"(T72 [{"Busy"=FALSE, "PumpCnt"=0.0, "RemoteEntered"=FALSE, "OverpressureSet"=FALSE}, {"Busy"=FALSE, "PumpCnt"=0.0, "RemoteEntered"=FALSE, "OverpressureSet"=FALSE}, {"Busy"=FALSE, "PumpCnt"=0.0, "RemoteEntered"=FALSE, "OverpressureSet"=FALSE}, {"Busy"=FALSE, "PumpCnt"=0.0, "RemoteEntered"=FALSE, "OverpressureSet"=FALSE}, {"Busy"=FALSE, "PumpCnt"=0.0, "RemoteEntered"=FALSE, "OverpressureSet"=FALSE}, {"Busy"=FALSE, "PumpCnt"=0.0, "RemoteEntered"=FALSE, "OverpressureSet"=FALSE}, {"Busy"=FALSE, "PumpCnt"=0.0, "RemoteEntered"=FALSE, "OverpressureSet"=FALSE}, {"Busy"=FALSE, "PumpCnt"=0.0, "RemoteEntered"=FALSE, "OverpressureSet"=FALSE}, {"Busy"=FALSE, "PumpCnt"=0.0, "RemoteEntered"=FALSE, "OverpressureSet"=FALSE}, {"Busy"=FALSE, "PumpCnt"=0.0, "RemoteEntered"=FALSE, "OverpressureSet"=FALSE}, {"Busy"=FALSE, "PumpCnt"=0.0, "RemoteEntered"=FALSE, "OverpressureSet"=FALSE}] ("ASIA Pump Global")) -> ()  [unwired: 1 in, 1 out]
      n6 = invoke class="Clust (strict)" method="Reinit To Default"() -> (error out=w91:errorcluster)  [unwired: 3 in, 2 out]
      n7 = Set Menu Item Info(7:w89, 9:TRUE ("enabled"), 10:w89, 11:w90) -> ()  [unwired: 3 in, 2 out]
    }
    frame #1 {
      n8 = disable-structure shown="Enabled" {
        frame Disabled {
          n9 = property on="Start Log" class="Bool"("Value"=FALSE) -> ()  [unwired: 2 in, 2 out]
        }
        frame Enabled {
        }
      }
    }
  }
  n10 = vi-ref "Dynamic Shared Variables.lvlib:Alarm History.vi"() -> (w61:refnum<vi>)
  n11 = call <vilib>:"Enable Alarm & Event Notifications.vi"() -> ("error out"=w44:errorcluster, "alarm & event notification"=w45:refnum<user-event>)  [unwired: 10 in]
  n12 = property class="VI"(reference=w61) -> ("Path"=w62:path)  [unwired: 1 in, 2 out]
  n13 = call "Create File.vi"("error in"=w39) -> ("error out"=w37:errorcluster)  [unwired: 10 in]
  n14 = Open VI Reference(type specifier VI Refnum (for type only)=refnum<vi> refnum, vi path=w62, options=128) -> (vi reference=w52:refnum<vi>, error out=w58:errorcluster)  [unwired: 3 in]
  n15 = register-events(error in=w44, w45) -> (reference out=w49:refnum<event-registration>, error out=w43:errorcluster)  [unwired: 1 in]
  n16 = call "Create User Event - Stop.vi"("error in (no error)"=w39) -> ("User Event - Stop"=w84:refnum<user-event>, "Stop Event Registration Refnum"=w48:refnum<event-registration>)  [unwired: 8 in, 1 out]
  n17 = call "Create Main Message Queues.vi"("error in (no error)"=w37, "Process Name"=w80) -> ("error out"=w81:errorcluster, "Message Queues out"=w29:T73)  [unwired: 8 in]
  n18 = Create User Event(user event datatype=w57, error in=w58) -> (user event=w51:refnum<user-event>)  [unwired: 1 out]
  n19 = Unbundle By Name(w29) -> ("UI"=w82:refnum<queue>, "DAQ"=w64:refnum<queue>, "Sequence"=w42:refnum<queue>, "CSV Log"=w41:refnum<queue>, "Sequence UI"=w31:refnum<queue>, "OPC UA Log"=w30:refnum<queue>, "Waveform Loop"=w24:refnum<queue>, "TDMS Log"=w23:refnum<queue>, "Graphs"=w22:refnum<queue>[], "TCP Write"=w21:refnum<queue>, "TCP Read"=w20:refnum<queue>, "OPC UA Log"=w19:refnum<queue>)
  n20 = call "Tag FGV.vi"("Operation"=Tag_FGV_Operation_Enum."Set Notification Queue", "Data"=w45, "error in (no error)"=w43) -> ()  [unwired: 5 in, 8 out]
  n21 = Current VI's Path() -> (path=w78:path)
  n22 = Bundle("Event Registration Refnum"=w49, "Stop Event Registration Refnum"=w48) -> (w47:T74)  [unwired: 1 in]
  n23 = Strip Path(path=w78) -> (stripped path=w68:path)  [unwired: 1 out]
  n24 = Build Path(base path=w68, name or relative path="History Graph") -> (appended path=w66:path)
  n25 = while {
    tunnel: w82 -> [w98]
    tunnel: [w107] -> w86
    shift-right: [w105] -> w83
    shift-left: w47 -> [w109]
    tunnel: w64 -> [w97]
    shift-right: [w103] -> _
    shift-left: T71 {"Down"=FALSE, "Mouse"={"Mouse Position"={"X"=0, "Y"=0}, "Mouse Modifiers"={"Button Down"=FALSE, "Shift Mod"=FALSE, "Menu Mod"=FALSE, "Option Mod"=FALSE}}, "Drag"=FALSE, "Canvas"=FALSE} -> [w104]
    tunnel: w52 -> [w101]
    tunnel: w51 -> [w100]
    tunnel: w42 -> [w96]
    stop <- w106 stop-if-true
    # "Event Handling Loop"
    n26 = event shown="[16] \"End Program\": Value Change" {
      selector: w109 -> [_ _ _ _ _ _ _ _ _ _ _ _ _ _ _ _ _]
      dyn-events: [_ _ _ _ _ _ _ _ _ _ _ _ _ _ _ _ _] -> w105
      timeout: 1000 -> [_ _ _ _ _ _ _ _ _ _ _ _ _ _ _ _ _]
      tunnel: w98 -> [w113 w120 w128 w146 w164 w199 w209 w230 w234 w245 w252 w263 w270 w311 w319 w330 w341]
      tunnel: [w116 w119 w125 w144 _ w184 w210 _ w236 w238 w251 w262 w267 _ _ w327 w336] -> w108
      tunnel: [TRUE _ _ _ _ _ _ _ _ _ FALSE FALSE w269 _ _ TRUE TRUE] -> w106
      tunnel: w97 -> [_ _ _ _ _ _ _ _ _ _ _ _ w268 _ _ _ _]
      tunnel: w104 -> [w110 w117 w123 w148 w175 w200 w208 w231 w232 w242 w247 w259 w266 w313 w321 w329 w337]
      tunnel: [w110 w117 w122 w147 w175 w200 w208 w231 w232 w242 w247 w259 w266 w312 w322 w329 w337] -> w103
      tunnel: [w112 w118 w128 w145 w163 w199 w209 w230 w233 w244 w250 w261 w270 w311 w319 w328 w335] -> w102
      tunnel: w101 -> [_ _ _ _ _ _ _ w226 _ _ _ _ _ _ _ _ _]
      tunnel: w100 -> [_ _ _ _ _ _ _ w225 _ _ _ _ _ _ _ _ _]
      tunnel: w96 -> [_ _ _ _ w161 _ _ _ _ _ _ _ _ _ _ _ _]
      event "Exit": Value Change {
        w114 = TRUE  # Priority Message
        # "The UI Message Loop handles sending the Exit message to other loops."
        n27 = event-data() -> ()  [unwired: 1 in, 1 out]
        n28 = call-poly "Enqueue Message.vi"("Priority Message? (F)"=w114, "Message"="Exit", "Message Queue"=w113) -> ("error out"=w116:errorcluster, "dup Message Queue"=w112:refnum<queue>)  [unwired: 7 in]
      }
      event "Force Trigger": Value Change {
        n29 = event-data() -> ()  [unwired: 1 in, 1 out]
        n30 = call-poly "Enqueue Message.vi"("Message"="Force Trigger", "Message Queue"=w120) -> ("error out"=w119:errorcluster, "dup Message Queue"=w118:refnum<queue>)  [unwired: 8 in]
      }
      event Mouse Up {
        # "If we are draging a module and we are over the canvas"
        n31 = event-data() -> ("Coords"=w127:T10)  [unwired: 1 in]
        n32 = in-place {
          in-place-border: w128 -> [w135]
          in-place-border: w127 -> [w134]
          in-place-border: [w133] -> w126
          w129 = FALSE ("Down")
          n33 = in-place-cluster #1(w123) -> ("Drag"=w131:bool, "Canvas"=w130:bool)  [unwired: 1 out]
          n34 = Compound Arithmetic op=AND(w131, w130) -> (w132:bool)
          n35 = case shown="False" w132 {
            tunnel: [_ w136] -> w133
            tunnel: w135 -> [_ w139]
            tunnel: w134 -> [_ w138]
            frame False {
            }
            frame True {
              n36 = property on="Canvas" class="Pict"() -> ("Mouse"=w141:T68)  [unwired: 2 in, 2 out]
              n37 = Bundle("Coords"=w138, "Mouse"=w141) -> (w137:cluster{"Coords":T10, "Mouse":T68})  [unwired: 1 in]
              "output cluster" <- w137
              n38 = call-poly "Enqueue Message.vi"("Message Data"=w137, "Message"="Drop", "Message Queue"=w139) -> ("error out"=w136:errorcluster)  [unwired: 7 in, 1 out]
            }
          }
          n39 = in-place-cluster #1("Down"=w129, "Drag"=w129, "Canvas"=w129) -> (w122:T71)
        }
        n40 = call-poly <vilib>:"Set Cursor.vi"("error in (no error)"=w126, "icon"=u16 0) -> ("error out"=w125:errorcluster)  [unwired: 8 in, 1 out]
      }
      event "Palette": Mouse Down {
        n41 = event-data() -> ()  [unwired: 1 in, 1 out]
        n42 = property on="Palette" class="Pict"() -> ("DisabledEnum"=w143:T77)  [unwired: 2 in, 2 out]
        n43 = call "Enable Disable Enum to Enabled.vi"("Disabled"=w143) -> ("Enabled"=w142:bool)
        n44 = case "Is the palette enabled?" shown="True" w142 {
          tunnel: w148 -> [w149 w160]
          tunnel: [w149 w158] -> w147
          tunnel: w146 -> [w150 w154]
          tunnel: [w150 w153] -> w145
          tunnel: [_ w152] -> w144
          frame False {
          }
          frame True {
            # "Select a module"
            n45 = property on="Palette" class="Pict"() -> ("Mouse"=w151:T68)  [unwired: 2 in, 2 out]
            n46 = Bundle By Name(cluster=w160, "Down"=TRUE, "Mouse"=w151, "Drag"=TRUE, "Canvas"=FALSE) -> (w158:T71)
            n47 = call-poly "Enqueue Message.vi"("Message Data"=w151, "Message"="Drag Start", "Message Queue"=w154) -> ("error out"=w152:errorcluster, "dup Message Queue"=w153:refnum<queue>)  [unwired: 7 in]
          }
        }
      }
      event Timeout {
        # "Poll for alarm status and display on UI. This could be changed\nto an alarm Event if necessary."
        n48 = event-data() -> ()  [unwired: 1 in, 1 out]
        n49 = call "Tag FGV.vi"("Operation"=Tag_FGV_Operation_Enum."Read Alarms") -> ("alarms"=w169:T78)  [unwired: 7 in, 7 out]
        n50 = property on="UI Alarms" class="Arr (strict)"() -> ("Number of Columns"=w172:u32)  [unwired: 2 in, 2 out]
        n51 = call "Is Critical Alarm Set.vi"("alarms"=w169) -> ("critical alarm?"=w167:bool)  [unwired: 10 in]
        n52 = call "Alarm UI.vi"("alarms"=w169) -> ("UI Alarms"=w174:T66[], "Alarm Model"=→"Alarm Model":T65[])  [unwired: 9 in]
        n53 = Array Size(array=w174) -> (size(s)=w173:i32)
        n54 = Greater?(x=w173, y=w172) -> (0:w171:bool)
        n55 = feedback #2() -> (w168:bool)  [unwired: 1 in]
        n56 = feedback-in #2(w167) -> ()
        n57 = local write "UI Alarms"(w174) -> ()
        n58 = property on="UI Alarms" class="Arr (strict)"("HorizScroll"=w171) -> ()  [unwired: 2 in, 2 out]
        n59 = property on="Alarm Model" class="Arr (strict)"("Visible"=TRUE) -> ()  [unwired: 2 in, 2 out]
        n60 = Compound Arithmetic op=AND(w167, invert w168) -> (w166:bool)
        n61 = case "critical alarm just occured?" shown="False" w166 {
          tunnel: [w176 w180] -> w163
          tunnel: w164 -> [w176 w179]
          tunnel: w161 -> [_ w177]
          frame False {
          }
          frame True {
            n62 = call-poly "Enqueue Message.vi"("Message"="E-Stop", "Message Queue"=w179) -> ("dup Message Queue"=w180:refnum<queue>)  [unwired: 8 in, 1 out]
            n63 = call-poly "Enqueue Message.vi"("Message"="Pause", "Message Queue"=w177) -> ()  [unwired: 8 in, 2 out]
          }
        }
      }
      event User Event {
        w197 = T79 {"alarm URL"="", "set time"=timestamp(0 s since 1904-01-01), "set user"="", "ack time"=timestamp(0 s since 1904-01-01), "ack user"="", "clear time"=timestamp(0 s since 1904-01-01), "clear user"="", "setpoint"=0.0, "value"=0.0, "priority"=0, "alarm area"="", "alarm description"="", "ack comment"="", "event?"=FALSE, "Refnum"=0}  # Alarm
        # "NI Example on how this works: .. \\LabVIEW 2018\\examples\\lvdsc\\Data and Alarm Historical Logging\\DSC Alarms Demo\\component\\DSC Alarms Event Structure Support.vi"
        # "critical alarm?"
        n64 = event-data() -> ("alarm URL"=w196:string, "set time"=w195:timestamp, "set user"=w194:string, "ack time"=w193:timestamp, "ack user"=w192:string, "clear time"=w191:timestamp, "clear user"=w190:string, "setpoint"=w189:dbl, "value"=w188:dbl, "priority"=w185:u32, "alarm area"=w187:string, "alarm description"=w186:string)  [unwired: 1 in]
        n65 = Bundle By Name(cluster=w197, "alarm URL"=w196, "set time"=w195, "set user"=w194, "ack time"=w193, "ack user"=w192, "clear time"=w191, "clear user"=w190, "setpoint"=w189, "value"=w188, "priority"=w185, "alarm area"=w187, "alarm description"=w186) -> (w183:T79)
        n66 = Greater?(x=w195, y=timestamp(2272129200 s since 1904-01-01)) -> (0:w182:bool)
        n67 = case "valid time stamp?" shown="True" w182 {
          tunnel: [w201 w206] -> w184
          tunnel: w183 -> [_ w202]
          frame False {
            n68 = call <vilib>:"Clear Errors.vi"() -> ("error out"=w201:errorcluster)  [unwired: 6 in, 1 out]
          }
          frame True {
            # "Log alarm to alarm\nCSV file."
            n69 = call "Log Alarm FGV.vi"("Alarm"=w202, "Operation"=Alarm_Log_Operation_Enum."Log Alarm") -> ("error out"=w206:errorcluster)  [unwired: 9 in]
            n70 = Flatten To XML(anything=w202) -> (xml string=w203:string)
            n71 = Concatenate Strings("ALARM: " ("text"), w203) -> (w204:string)
            n72 = call "Write to Log File.vi"("error in"=w206, "text"=w204) -> ()  [unwired: 9 in, 1 out]
          }
        }
        n73 = disable-structure shown="Disabled" {
          frame Disabled {
            # "Example of\nalarm events using\nsame low level VIs."
            n74 = call "DSC Alarm Event Example.vi"() -> ()  [unwired: 12 in]
          }
          frame Enabled {
          }
        }
      }
      event "UI Alarms": Value Change {
        # "Acknowlege the alarms when it's button is clicked"
        n75 = event-data() -> ()  [unwired: 1 in, 1 out]
        n76 = local read "Alarm Model"() -> (w212:T65[])
        n77 = call <vilib>:"Clear Errors.vi"() -> ("error out"=w211:errorcluster)  [unwired: 6 in, 1 out]
        n78 = for {
          shift-right: [w218] -> w210
          shift-left: w211 -> [w219]
          tunnel: "UI Alarms" -> [w217] mode=indexing
          tunnel: w212 -> [w215] mode=indexing
          n79 = Unbundle By Name(w215) -> ("Alarm"=w214:T79)
          n80 = Unbundle By Name(w217) -> ("Ack"=w216:bool)
          n81 = case shown="True" w216 {
            tunnel: w219 -> [w220 w224]
            tunnel: [w220 w223] -> w218
            tunnel: w214 -> [_ w221]
            frame False {
            }
            frame True {
              n82 = call "Tag FGV.vi"("Operation"=Tag_FGV_Operation_Enum."Ack Alarm", "Data"=w221, "error in (no error)"=w224) -> ("error out"=w223:errorcluster)  [unwired: 5 in, 7 out]
            }
          }
        }
      }
      event "Alarm History Button": Value Change {
        # "Open Alarm History VI"
        # "Don't care if VI is\nalready running."
        n83 = event-data() -> ()  [unwired: 1 in, 1 out]
        n84 = call-by-ref "Start Asynchronous Call"(reference=w226, "user event"=w225) -> (reference out=w228:refnum<vi>, error out=w227:errorcluster)  [unwired: 12 in]
        n85 = call <vilib>:"Clear Errors.vi"("error in (no error)"=w227) -> ()  [unwired: 5 in, 2 out]
        n86 = invoke class="VI (strict)" method="FP.Open"(reference=w228, "State"=T76."Standard") -> ()  [unwired: 3 in, 5 out]
        n87 = disable-structure shown="Disabled" {
          frame Disabled {
            n88 = call "Alarm History.vi"() -> ()  [unwired: 12 in]
          }
          frame Enabled {
          }
        }
      }
      event "Settings": Value Change {
        n89 = event-data() -> ()  [unwired: 1 in, 1 out]
        n90 = call-poly "Enqueue Message.vi"("Message"="Launch Settings Dialog", "Message Queue"=w234) -> ("error out"=w236:errorcluster, "dup Message Queue"=w233:refnum<queue>)  [unwired: 8 in]
      }
      event "Start Log": Value Change {
        w237 = "Add Note" ("item name")
        # "Add the menu item when the Log is Started"
        n91 = event-data() -> ()  [unwired: 1 in, 1 out]
        n92 = call-poly "Enqueue Message.vi"("Message"="Start Log", "Message Queue"=w245) -> ("error out"=w239:errorcluster, "dup Message Queue"=w244:refnum<queue>)  [unwired: 8 in]
        n93 = property on="Pause Log Button" class="Bool (strict)"("Val(Sgnl)"=FALSE ("Pause Log Button")) -> ()  [unwired: 2 in, 2 out]
        n94 = Current VI's Menubar() -> (w241:refnum<k9>)
        n95 = Set Menu Item Info(7:w237, 8:w239, 9:TRUE ("enabled"), 10:w237, 11:w241) -> (0:w238:errorcluster)  [unwired: 2 in, 1 out]
      }
      event "Pause Log Button": Value Change {
        n96 = event-data() -> ()  [unwired: 1 in, 1 out]
        n97 = global write "Main Globals.vi" "Pause Log"("Pause Log Button") -> ()
        n98 = disable-structure shown="Enabled" {
          disable-tunnel: w252 -> [w257 w258]
          disable-tunnel: [w256 _] -> w251
          disable-tunnel: [w255 w258] -> w250
          disable-tunnel: "Pause Log Button" -> [w253 _]
          frame Disabled {
            n99 = call-poly "Enqueue Message.vi"("Message Data"=w253, "Message"="Pause Log", "Message Queue"=w257) -> ("error out"=w256:errorcluster, "dup Message Queue"=w255:refnum<queue>)  [unwired: 7 in]
          }
          frame Enabled {
          }
        }
      }
      event "E-Stop": Value Change {
        n100 = event-data() -> ()  [unwired: 1 in, 1 out]
        n101 = call-poly "Enqueue Message.vi"("Message"="E-Stop", "Message Queue"=w263) -> ("error out"=w262:errorcluster, "dup Message Queue"=w261:refnum<queue>)  [unwired: 8 in]
      }
      event Menu Selection (User) {
        n102 = event-data() -> ("ItemTag"=w265:string)  [unwired: 1 in]
        n103 = case shown="\"Save Campaign As...\"" w265 {
          tunnel: w270 -> [_ _ _ w282 w285 w288 w292 w294 w297 w301 w304 w309]
          tunnel: [_ _ _ _ _ _ _ _ _ _ _ TRUE] -> w269
          tunnel: w268 -> [_ _ w280 _ _ _ _ _ _ _ _ _]
          tunnel: [w271 w272 w279 w283 w286 w289 w293 w295 w298 w300 w303 w308] -> w267
          frame Default {
            n104 = call <vilib>:"Clear Errors.vi"() -> ("error out"=w271:errorcluster)  [unwired: 6 in, 1 out]
          }
          frame "Open BMP" {
            n105 = call "File Dialog"() -> ("selected path"=w273:path, "cancelled"=w274:bool)  [unwired: 12 in, 2 out]
            n106 = case shown="False" w274 {
              tunnel: w273 -> [w276 _]
              frame False {
                n107 = call "Empty Picture"() -> ("empty picture"=w275:picture)
                n108 = call "Draw BMP at Location.vi"("selected path"=w276, "picture in"=w275) -> ("image data"=→"image data":T69, "picture out"=→"Canvas":picture)  [unwired: 7 in, 1 out]
              }
              frame True {
              }
            }
            n109 = call <vilib>:"Clear Errors.vi"() -> ("error out"=w272:errorcluster)  [unwired: 6 in, 1 out]
          }
          frame "DAQSettings" {
            # "Open the DAQ Settings dialog"
            n110 = call-poly "Enqueue Message.vi"("Message"="DAQ-Settings", "Message Queue"=w280) -> ("error out"=w279:errorcluster)  [unwired: 8 in, 1 out]
          }
          frame "Open Campaign" {
            n111 = call-poly "Enqueue Message.vi"("Message"="Open Campaign", "Message Queue"=w282) -> ("error out"=w283:errorcluster)  [unwired: 8 in, 1 out]
          }
          frame "Save Campaign" {
            n112 = call-poly "Enqueue Message.vi"("Message"="Save Campaign", "Message Queue"=w285) -> ("error out"=w286:errorcluster)  [unwired: 8 in, 1 out]
          }
          frame "Save Campaign As..." {
            n113 = call-poly "Enqueue Message.vi"("Message"="Save Campaign As", "Message Queue"=w288) -> ("error out"=w289:errorcluster)  [unwired: 8 in, 1 out]
          }
          frame "FileSettings" {
            # "Open the File Settings dialog"
            n114 = call-poly "Enqueue Message.vi"("Message"="File-Settings", "Message Queue"=w292) -> ("error out"=w293:errorcluster)  [unwired: 8 in, 1 out]
          }
          frame "Set Sequence" {
            n115 = call-poly "Enqueue Message.vi"("Message"="Launch Sequence Dialog", "Message Queue"=w294) -> ("error out"=w295:errorcluster)  [unwired: 8 in, 1 out]
          }
          frame "Set Data Rate" {
            n116 = call-poly "Enqueue Message.vi"("Message"="Launch Data Rate Dialog", "Message Queue"=w297) -> ("error out"=w298:errorcluster)  [unwired: 8 in, 1 out]
          }
          frame "Launch Calibration Dialog" {
            n117 = call-poly "Enqueue Message.vi"("Message"="Launch Calibration Dialog", "Message Queue"=w301) -> ("error out"=w300:errorcluster)  [unwired: 8 in, 1 out]
          }
          frame "Add Note" {
            n118 = call-poly "Enqueue Message.vi"("Message"="Launch Note Dialog", "Message Queue"=w304) -> ("error out"=w303:errorcluster)  [unwired: 8 in, 1 out]
          }
          frame "Exit" {
            w306 = TRUE  # Priority Message
            n119 = call-poly "Enqueue Message.vi"("Priority Message? (F)"=w306, "Message"="Exit", "Message Queue"=w309) -> ("error out"=w308:errorcluster)  [unwired: 7 in, 1 out]
          }
        }
      }
      event "Canvas": Mouse Enter {
        n120 = event-data() -> ()  [unwired: 1 in, 1 out]
        n121 = Unbundle By Name(w313) -> ("Drag"=w314:bool)
        n122 = case shown="False" w314 {
          tunnel: w313 -> [w315 w318]
          tunnel: [w315 w317] -> w312
          frame False {
          }
          frame True {
            n123 = Bundle By Name(cluster=w318, "Canvas"=TRUE) -> (w317:T71)
          }
        }
      }
      event "Canvas": Mouse Leave {
        n124 = event-data() -> ()  [unwired: 1 in, 1 out]
        n125 = Unbundle By Name(w321) -> ("Canvas"=w320:bool)
        n126 = case shown="False" w320 {
          tunnel: w321 -> [w323 w326]
          tunnel: [w323 w325] -> w322
          frame False {
          }
          frame True {
            n127 = Bundle By Name(cluster=w326, "Canvas"=FALSE) -> (w325:T71)
          }
        }
      }
      event Panel Close? {
        w331 = TRUE  # Priority Message
        # "Send the 'Confirm Quit' message if the user closes the panel of the VI. Discard the event so the 'Confirm Quit' message has a chance to run."
        n128 = event-data() -> ()  [unwired: 1 in, 1 out]
        n129 = invoke class="VI" method="FP.Close"() -> ()  [unwired: 3 in, 3 out]
        n130 = call-poly "Enqueue Message.vi"("Priority Message? (F)"=w331, "Message"="Exit", "Message Queue"=w330) -> ("error out"=w327:errorcluster, "dup Message Queue"=w328:refnum<queue>)  [unwired: 7 in]
        n131 = event-data("Discard?"=TRUE) -> ()  [unwired: 1 in, 1 out]
      }
      event "End Program": Value Change {
        w338 = FALSE  # Priority Message
        # "Send the 'Confirm Quit' message if the user closes the panel of the VI. Discard the event so the 'Confirm Quit' message has a chance to run."
        n132 = event-data() -> ()  [unwired: 1 in, 1 out]
        n133 = call-poly "Enqueue Message.vi"("Priority Message? (F)"=w338, "Message"="Exit", "Message Queue"=w341) -> ("error out"=w336:errorcluster, "dup Message Queue"=w335:refnum<queue>)  [unwired: 7 in]
      }
    }
    n134 = call "Error Handler - Event Handling Loop.vi"("error in (no error)"=w108, "Message Queue"=w102) -> ("dup error in"=w107:errorcluster)  [unwired: 8 in, 1 out]
  }
  n135 = disable-structure shown="Enabled" {
    disable-tunnel: w29 -> [w342 w343]
    frame Disabled {
      n136 = call "OSIPI OPCUA Server.vi"("Main Queue Cluster"=w342) -> ()  [unwired: 11 in]
    }
    frame Enabled {
      n137 = call "OSIPI OPCUA Server Tag Version.vi"("Main Queue Cluster"=w343) -> ()  [unwired: 11 in]
    }
  }
  n138 = call "Sequence.vi"("Message Queues in"=w29) -> ("error out"=w32:errorcluster)  [unwired: 10 in]
  n139 = call "TCP Write.vi"("Message Queues out"=w29) -> ()  [unwired: 11 in]
  n140 = call "Waveform Loop.vi"("Message Queues out"=w29) -> ("error out"=w36:errorcluster)  [unwired: 10 in]
  n141 = call "TDMS Log Loop.vi"("Message Queues"=w29) -> ("error out"=w35:errorcluster)  [unwired: 10 in]
  n142 = call "DAQ Message Loop.vi"("Message Queues"=w29) -> ("error out"=w34:errorcluster)  [unwired: 10 in]
  n143 = call "CSV Log Loop.vi"("Message Queues"=w29) -> ("error out"=w33:errorcluster)  [unwired: 10 in]
  n144 = while {
    tunnel: w82 -> [w364]
    tunnel: w84 -> [w369]
    shift-right: [w362] -> w87
    shift-left: w81 -> [w368]
    tunnel: w80 -> [w360]
    tunnel: w29 -> [w359]
    shift-right: [w357] -> _
    shift-left: w40 -> [w358]
    tunnel: w29 -> [w356]
    tunnel: w64 -> [w353]
    tunnel: w42 -> [w352]
    tunnel: w41 -> [w350]
    tunnel: w31 -> [w354]
    tunnel: w30 -> [w351]
    tunnel: [w355] -> w28
    tunnel: [w353] -> w27
    tunnel: [w351] -> w26
    tunnel: [w350] -> w25
    tunnel: w24 -> [w349]
    tunnel: w23 -> [w348]
    tunnel: w22 -> [w347]
    tunnel: w21 -> [w346]
    tunnel: w20 -> [w345]
    tunnel: w19 -> [w344]
    tunnel: [w349] -> w18
    tunnel: [w348] -> w17
    tunnel: [w347] -> w16
    tunnel: [w346] -> w15
    tunnel: [w345] -> w14
    tunnel: [w344] -> w13
    stop <- w370 stop-if-true
    # "UI Message Loop"
    n145 = call "Dequeue Message.vi"("error in (no error)"=w368, "Message Queue"=w364) -> ("error out"=w367:errorcluster, "Message Data"=w365:variant, "Message"=w366:string, "dup Message Queue"=w361:refnum<queue>)  [unwired: 6 in]
    n146 = case "Message Cases" shown="\"Exit\"" w366 {
      selector: w366 -> [_ _ _ _ _ _ _ _ _ _ _ _ _ _ _ _ _ _ _ _ _ _ _ _ _ _ _ _ _ _ _ _ _ _ _ _ _ _ w1445 _ _ _ _ _ _ _ w1619 _]
      tunnel: w361 -> [_ _ _ _ _ _ _ _ _ _ _ _ _ _ _ w897 w921 w945 w969 w993 w1017 w1041 w1067 w1091 w1115 w1139 _ _ w1201 _ w1266 _ _ w1329 _ w1376 w1424 _ _ w1492 _ _ _ _ _ _ _ _]
      tunnel: w367 -> [w373 w381 w400 w445 w490 w535 w577 w620 w663 w706 w748 w791 w834 w879 w889 w896 w920 w944 w968 w992 w1016 w1040 w1066 w1090 w1114 w1138 w1162 w1193 w1208 w1249 _ w1280 w1316 w1328 w1365 w1389 _ w1434 w1451 w1500 w1554 w1560 w1572 w1604 w1610 w1616 _ w1628]
      tunnel: [w372 w374 w392 w437 w482 w527 w572 w615 w658 w701 w744 w787 w830 w873 w887 w894 w918 w942 w966 w990 w1014 w1038 w1064 w1088 w1112 w1136 w1160 w1179 w1200 w1247 w1258 w1275 w1312 w1320 w1359 w1374 w1420 w1429 w1439 w1478 w1546 w1560 w1562 w1603 w1608 w1612 w1618 w1628] -> w363
      tunnel: [_ _ _ _ _ _ _ _ _ _ _ _ _ _ _ _ _ _ _ _ _ _ _ _ _ _ _ _ _ FALSE _ TRUE _ _ _ _ _ _ _ _ _ _ _ _ _ _ _ _] -> w370
      tunnel: w365 -> [_ w382 w401 w446 w491 w536 w578 w621 w664 w707 w749 w792 w835 w880 _ _ _ _ _ _ _ _ _ _ _ _ _ w1192 w1210 _ w1268 _ _ _ _ _ _ _ _ _ _ _ _ _ _ _ _ _]
      tunnel: w369 -> [_ _ _ _ _ _ _ _ _ _ _ _ _ _ _ _ _ _ _ _ _ _ _ _ _ _ _ _ _ _ _ w1297 _ _ _ _ _ _ _ _ _ _ _ _ _ _ _ _]
      tunnel: w360 -> [_ _ _ _ _ _ _ _ _ _ _ _ _ _ _ _ _ _ _ _ _ _ _ _ _ _ _ _ _ _ _ _ _ _ _ _ _ _ _ _ _ _ _ _ _ _ _ _]
      tunnel: w359 -> [_ _ _ _ _ _ _ _ _ _ _ _ _ _ _ _ _ _ _ _ _ _ _ _ _ _ _ _ _ _ _ _ _ _ _ _ _ _ _ _ _ _ _ _ _ _ _ _]
      tunnel: w358 -> [w371 w379 w391 w436 w481 w526 w571 w614 w657 w700 w743 w786 w829 w872 w891 w900 w924 w948 w972 w996 w1020 w1044 w1070 w1094 w1118 w1142 w1163 w1184 w1207 w1252 w1264 w1284 w1315 w1317 w1373 w1379 w1423 w1432 w1438 w1476 w1555 w1559 w1565 w1601 w1607 w1615 w1627 w1630]
      tunnel: [w371 w380 w390 w435 w480 w525 w570 w613 w656 w699 w742 w785 w828 w871 w891 w901 w925 w949 w973 w997 w1021 w1045 w1071 w1095 w1119 w1143 w1163 w1185 w1195 w1251 w1264 w1285 w1311 w1351 w1373 w1380 w1423 w1433 w1446 w1476 w1555 w1559 w1569 w1602 w1607 w1615 w1627 w1630] -> w357
      tunnel: w356 -> [_ _ _ _ _ _ _ _ _ _ _ _ _ _ _ _ _ _ _ _ _ _ _ _ _ _ _ _ _ _ _ w1296 _ _ _ _ _ _ _ w1510 w1557 _ _ _ _ _ _ _]
      tunnel: w353 -> [_ _ _ _ _ _ _ _ _ _ _ _ _ _ w892 _ _ _ _ _ _ _ _ _ _ _ _ _ _ _ _ _ _ _ w1369 w1375 _ _ _ _ _ _ _ _ _ _ _ _]
      tunnel: w352 -> [_ _ _ _ _ _ _ _ _ _ _ _ _ _ _ _ _ _ _ _ _ _ _ _ _ _ _ _ _ _ _ _ _ _ _ _ _ _ _ _ _ _ w1567 _ _ _ _ _]
      tunnel: w350 -> [_ _ _ _ _ _ _ _ _ _ _ _ _ _ _ _ _ _ _ _ _ _ _ _ _ _ _ _ _ _ _ _ _ _ _ _ _ _ _ w1491 _ _ _ _ _ w1617 _ _]
      tunnel: w354 -> [_ _ _ _ _ _ _ _ _ _ _ _ _ _ _ _ _ _ _ _ _ _ _ _ _ _ _ _ _ _ _ _ _ _ _ _ _ _ _ _ _ _ w1561 _ _ _ _ _]
      tunnel: w351 -> [_ _ _ _ _ _ _ _ _ _ _ _ _ _ _ _ _ _ _ _ _ _ _ _ _ _ _ _ _ _ _ _ _ _ _ _ _ _ _ w1477 _ _ _ _ _ _ _ _]
      frame "---Copy This Frame---" {
        # "Duplicate this frame when creating new messages.  Change this comment in the duplicated frame to describe this message."
        n147 = Merge Errors(w373) -> (w372:errorcluster)
      }
      frame "Commit Config (DAQ)" {
        # "Save DAQ Settings"
        n148 = Unbundle By Name(w379) -> ("Main Config.DAQ Config"=w378:T36)
        n149 = Variant To Data(error in=w381, type=w378, Variant=w382) -> (data=w376:T36, error out=w377:errorcluster)
        n150 = case shown="No Error" w377 {
          selector: w377 -> [w383 w388]
          tunnel: [w387 w389] -> w380
          tunnel: w379 -> [w386 w389]
          tunnel: w376 -> [w385 _]
          tunnel: [w383 w388] -> w374
          frame No Error {
            n151 = Bundle By Name(cluster=w386, "Main Config.DAQ Config"=w385, "Config Changed?"=TRUE) -> (w387:T1)
          }
          frame Error {
          }
        }
        n152 = call "Write to Log File.vi"("error in"=w374, "text"="Main: Commit Config (DAQ)") -> ()  [unwired: 9 in, 1 out]
      }
      frame "Commit Config (Feed Module)" {
        # "Save Feed Module Settings"
        n153 = Variant To Data(error in=w400, type=T17 {"GUID"="", "Drop Coords"={"Horizontal"=0, "Vertical"=0}, "Process Name"="", "Queue Name"="", "Settings"={"Cycle Period"=500.0, "Ismatech"={"VISA resource name"="", "Simulated?"=TRUE, "Pump Number"=1.0, "Reverse?"=FALSE}, "Masterflex"={"VISA resource name"="", "Simulated?"=TRUE, "Pump Number"=1.0, "Reverse?"=FALSE}, "Mettler"={"VISA resource name"="", "Simulated?"=FALSE}, "Bronkhorst M13 Flow Meter"={"VISA resource name"="", "Simulated?"=TRUE}, "PID 2 Parameters"={"Input Device"=enum."Default", "Output Device"=enum."Default", "Setpoint"=0.0, "PID gains"={"proportional gain (Kc)"=1.0, "integral time (Ti, min)"=0.01, "derivative time (Td, min)"=0.0}}, "Manual Entry"=0.0, "Auto?"=TRUE, "output range"={"output high"=100.0, "output low"=0.0}, "Bronkhorst M14"={"VISA resource name"="", "Simulated?"=FALSE}, "Tacmina Settings"={"Analog DAQ Task"="", "Digital DAQ Task"=""}, "KNF SIMDOS Settings"={"VISA resource name"="", "Simulated?"=TRUE}, "ASIA Pump C"={"ASIA Pump #"=0, "channel"=0, "Simulated"=FALSE}, "VICI Settings"={"VISA resource name"="", "Simulated?"=TRUE, "Pump Letter"="", "Reverse?"=FALSE}, "FLOM Settings"={"VISA resource name"="", "Simulated?"=TRUE, "Pump Number"=0.0}, "SSI PR/LD Settings"={"VISA resource name"="", "Simulated?"=FALSE}, "Masterflex 75211 Settings"={"Analog DAQ Task"="", "Digital DAQ Task"=""}, "SSI P40 Settings"={"VISA resource name"="", "Simulated?"=TRUE}}, "Settings Load Count"=0, "OP Load Count"=0} ("Feed Module Config"), Variant=w401) -> (data=w399:T17, error out=w395:errorcluster)
        n154 = Unbundle By Name(w399) -> ("GUID"=w396:string)
        n155 = Format Into String(format string="Could not save Feed Module config. No matching GUID for \"%s\"." ("error message (\"\")"), w396) -> (resulting string=w397:string)  [unwired: 2 in, 1 out]
        n156 = in-place {
          in-place-border: w399 -> [w408]
          in-place-border: w397 -> [w407]
          in-place-border: w396 -> [w406]
          in-place-border: w395 -> [w405]
          in-place-border: [w404] -> w392
          n157 = in-place-cluster #3(w391) -> ("Main Config.Feed Module Configs"=w403:T17[])
          n158 = Empty Array?(array=w403) -> (empty?=w409:bool)
          n159 = case shown="True" w409 {
            tunnel: w406 -> [w417 _]
            tunnel: w403 -> [w415 w434]
            tunnel: w408 -> [w414 w433]
            tunnel: [w413 w432] -> w402
            tunnel: w407 -> [w412 _]
            tunnel: w405 -> [w411 w431]
            tunnel: [w410 w431] -> w404
            frame False {
              n160 = for {
                tunnel: w415 -> [w430] mode=indexing
                tunnel: [w429] -> w418 mode=indexing
                workers-P: _ -> [_]
                n161 = Unbundle By Name(w430) -> ("GUID"=w429:string)
              }
              n162 = Search 1D Array(1D array=w418, element=w417) -> (index of element=w416:i32)  [unwired: 1 in]
              n163 = case shown="0, Default" w416 {
                selector: w416 -> [w422 _]
                tunnel: w415 -> [w423 w428]
                tunnel: w414 -> [w421 _]
                tunnel: [w420 w428] -> w413
                tunnel: w412 -> [_ w426]
                tunnel: w411 -> [w419 w425]
                tunnel: [w419 w424] -> w410
                frame 0, Default {
                  n164 = Replace Array Subset(array=w423, new element=w421, index=w422) -> (w420:T17[])
                }
                frame -1 {
                  n165 = call <vilib>:"Error Cluster From Error Code.vi"("error in (no error)"=w425, "error message (\"\")"=w426, "error code (0)"=7004) -> ("error out"=w424:errorcluster)  [unwired: 6 in]
                }
              }
            }
            frame True {
              n166 = Build Array (concatenate)(w434, w433) -> (w432:T17[])
            }
          }
          n167 = in-place-cluster #3("Main Config.Feed Module Configs"=w402) -> (w390:T1)
        }
        n168 = call "Write to Log File.vi"("error in"=w392, "text"="Main: Commit Config (Feed Module)") -> ()  [unwired: 9 in, 1 out]
      }
      frame "Commit Config (OPC Module)" {
        # "Save Feed Module Settings"
        n169 = Variant To Data(error in=w445, type=T8 {"State"=enum."Idle", "GUID"="", "Drop Coords"={"Horizontal"=0, "Vertical"=0}, "Configuration"={"Cycle Period"=500.0, "server endpoint URL"="opc.tcp://10.131.1.22:4840", "security policy"={"message mode"=enum."Sign", "security"=enum."Basic256"}, "Trust Any Server"=FALSE}, "First Iteration"=FALSE, "Data"=[], "Process Name"="", "Load Count"=0, "Log Started"=FALSE, "subscription ID out"=0, "OPC UA client refnum out"="", "Event Registration Refnum"=refnum, "Start Time"=timestamp(0 s since 1904-01-01), "Current Time"=timestamp(0 s since 1904-01-01)} ("OPC Module Config"), Variant=w446) -> (data=w444:T8, error out=w440:errorcluster)
        n170 = Unbundle By Name(w444) -> ("GUID"=w441:string)
        n171 = Format Into String(format string="Could not save Feed Module config. No matching GUID for \"%s\"." ("error message (\"\")"), w441) -> (resulting string=w442:string)  [unwired: 2 in, 1 out]
        n172 = in-place {
          in-place-border: w444 -> [w453]
          in-place-border: w442 -> [w452]
          in-place-border: w441 -> [w451]
          in-place-border: w440 -> [w450]
          in-place-border: [w449] -> w437
          n173 = in-place-cluster #4(w436) -> ("Main Config.OPC Module Configs"=w448:T8[])
          n174 = Empty Array?(array=w448) -> (empty?=w454:bool)
          n175 = case shown="True" w454 {
            tunnel: w451 -> [w462 _]
            tunnel: w448 -> [w460 w479]
            tunnel: w453 -> [w459 w478]
            tunnel: [w458 w477] -> w447
            tunnel: w452 -> [w457 _]
            tunnel: w450 -> [w456 w476]
            tunnel: [w455 w476] -> w449
            frame False {
              n176 = for {
                tunnel: w460 -> [w475] mode=indexing
                tunnel: [w474] -> w463 mode=indexing
                workers-P: _ -> [_]
                n177 = Unbundle By Name(w475) -> ("GUID"=w474:string)
              }
              n178 = Search 1D Array(1D array=w463, element=w462) -> (index of element=w461:i32)  [unwired: 1 in]
              n179 = case shown="0, Default" w461 {
                selector: w461 -> [w467 _]
                tunnel: w460 -> [w468 w473]
                tunnel: w459 -> [w466 _]
                tunnel: [w465 w473] -> w458
                tunnel: w457 -> [_ w471]
                tunnel: w456 -> [w464 w470]
                tunnel: [w464 w469] -> w455
                frame 0, Default {
                  n180 = Replace Array Subset(array=w468, new element=w466, index=w467) -> (w465:T8[])
                }
                frame -1 {
                  n181 = call <vilib>:"Error Cluster From Error Code.vi"("error in (no error)"=w470, "error message (\"\")"=w471, "error code (0)"=7004) -> ("error out"=w469:errorcluster)  [unwired: 6 in]
                }
              }
            }
            frame True {
              n182 = Build Array (concatenate)(w479, w478) -> (w477:T8[])
            }
          }
          n183 = in-place-cluster #4("Main Config.OPC Module Configs"=w447) -> (w435:T1)
        }
        n184 = call "Write to Log File.vi"("error in"=w437, "text"="Main: Commit Config (Feed Module)") -> ()  [unwired: 9 in, 1 out]
      }
      frame "Commit Config (Pump Module)" {
        # "Save Pump Module Settings"
        n185 = Variant To Data(error in=w490, type=T41 {"GUID"="", "Drop Coords"={"Horizontal"=0, "Vertical"=0}, "Process Name"="", "Queue Name"="", "Settings"={"Cycle Period"=500.0, "Manual Entry"=0.0, "Output Device"=enum."Default", "Ismatech"={"VISA resource name"="", "Simulated?"=TRUE, "Pump Number"=1.0, "Reverse?"=FALSE}, "Masterflex"={"VISA resource name"="", "Simulated?"=TRUE, "Pump Number"=1.0, "Reverse?"=FALSE}, "VICI Settings"={"VISA resource name"="", "Simulated?"=TRUE, "Pump Letter"="", "Reverse?"=FALSE}, "Tacmina Settings"={"Analog DAQ Task"="", "Digital DAQ Task"=""}, "KNF SIMDOS Settings"={"VISA resource name"="", "Simulated?"=TRUE}, "ASIA Pump C"={"ASIA Pump #"=0, "channel"=0, "Simulated"=FALSE}, "FLOM Settings"={"VISA resource name"="", "Simulated?"=TRUE, "Pump Number"=0.0}, "SSI PR/LD Settings"={"VISA resource name"="", "Simulated?"=FALSE}, "SSI P40 Settings"={"VISA resource name"="", "Simulated?"=FALSE}, "Masterflex 75211 Settings"={"Analog DAQ Task"="", "Digital DAQ Task"=""}, "Pump Calibration File"=path "", "Calibration Slope"=0.0, "Calibration Y Intercept"=0.0, "Pump Cal Enum"=0}, "Load Count"=0} ("Pump Module Config"), Variant=w491) -> (data=w484:T41, error out=w486:errorcluster)
        n186 = Unbundle By Name(w484) -> ("GUID"=w487:string)
        n187 = Format Into String(format string="Could not save Pump Module config. No matching GUID for \"%s\"." ("error message (\"\")"), w487) -> (resulting string=w488:string)  [unwired: 2 in, 1 out]
        n188 = in-place {
          in-place-border: w488 -> [w498]
          in-place-border: w487 -> [w497]
          in-place-border: w486 -> [w496]
          in-place-border: w484 -> [w495]
          in-place-border: [w494] -> w482
          n189 = in-place-cluster #5(w481) -> ("Main Config.Pump Module Configs"=w493:T41[])
          n190 = Empty Array?(array=w493) -> (empty?=w499:bool)
          n191 = case shown="True" w499 {
            tunnel: w497 -> [w507 _]
            tunnel: w493 -> [w505 w524]
            tunnel: w495 -> [w504 w521]
            tunnel: [w503 w523] -> w492
            tunnel: w498 -> [w502 _]
            tunnel: w496 -> [w501 w522]
            tunnel: [w500 w522] -> w494
            frame False {
              n192 = for {
                tunnel: w505 -> [w520] mode=indexing
                tunnel: [w519] -> w508 mode=indexing
                workers-P: _ -> [_]
                n193 = Unbundle By Name(w520) -> ("GUID"=w519:string)
              }
              n194 = Search 1D Array(1D array=w508, element=w507) -> (index of element=w506:i32)  [unwired: 1 in]
              n195 = case shown="0, Default" w506 {
                selector: w506 -> [w512 _]
                tunnel: w505 -> [w513 w518]
                tunnel: w504 -> [w509 _]
                tunnel: [w511 w518] -> w503
                tunnel: w502 -> [_ w516]
                tunnel: w501 -> [w510 w515]
                tunnel: [w510 w514] -> w500
                frame 0, Default {
                  n196 = Replace Array Subset(array=w513, new element=w509, index=w512) -> (w511:T41[])
                }
                frame -1 {
                  n197 = call <vilib>:"Error Cluster From Error Code.vi"("error in (no error)"=w515, "error message (\"\")"=w516, "error code (0)"=7004) -> ("error out"=w514:errorcluster)  [unwired: 6 in]
                }
              }
            }
            frame True {
              n198 = Build Array (concatenate)(w524, w521) -> (w523:T41[])
            }
          }
          n199 = in-place-cluster #5("Main Config.Pump Module Configs"=w492) -> (w480:T1)
        }
        n200 = call "Write to Log File.vi"("error in"=w482, "text"="Main: Commit Config (Pump Module)") -> ()  [unwired: 9 in, 1 out]
      }
      frame "Commit Config (DO)" {
        # "Save Digital Output Module Settings"
        n201 = Variant To Data(error in=w535, type=T56 {"GUID"="", "Drop Coords"={"Horizontal"=0, "Vertical"=0}, "Process Name"="", "Queue Name"="", "Settings"={"Valve Settings"={"D-O Settings"={"DAQmx Task Name"="", "Output Channel"=0, "Output Channel Names"=[]}, "VICI Electronic Actuator"={"VISA resource name"="", "Mode"=enum."Two Positions With Stops", "Simulated"=FALSE}}, "Valve Type"=enum."Default", "Time On (Sec)"=0.0, "Time Off (Sec)"=0.0, "Run?"=FALSE}, "Load Count"=0} ("D-O Module Config"), Variant=w536) -> (data=w534:T56, error out=w530:errorcluster)
        n202 = Unbundle By Name(w534) -> ("GUID"=w531:string)
        n203 = Format Into String(format string="Could not save Digital Out Module config. No matching GUID for \"%s\"." ("error message (\"\")"), w531) -> (resulting string=w532:string)  [unwired: 2 in, 1 out]
        n204 = in-place {
          in-place-border: w534 -> [w543]
          in-place-border: w532 -> [w542]
          in-place-border: w531 -> [w541]
          in-place-border: w530 -> [w540]
          in-place-border: [w539] -> w527
          n205 = in-place-cluster #6(w526) -> ("Main Config.DO Module Configs"=w538:T56[])
          n206 = Empty Array?(array=w538) -> (empty?=w544:bool)
          n207 = case shown="True" w544 {
            tunnel: w541 -> [w552 _]
            tunnel: w538 -> [w550 w569]
            tunnel: w543 -> [w549 w568]
            tunnel: [w548 w567] -> w537
            tunnel: w542 -> [w547 _]
            tunnel: w540 -> [w546 w566]
            tunnel: [w545 w566] -> w539
            frame False {
              n208 = for {
                tunnel: w550 -> [w565] mode=indexing
                tunnel: [w564] -> w553 mode=indexing
                workers-P: _ -> [_]
                n209 = Unbundle By Name(w565) -> ("GUID"=w564:string)
              }
              n210 = Search 1D Array(1D array=w553, element=w552) -> (index of element=w551:i32)  [unwired: 1 in]
              n211 = case shown="0, Default" w551 {
                selector: w551 -> [w557 _]
                tunnel: w550 -> [w558 w563]
                tunnel: w549 -> [w556 _]
                tunnel: [w555 w563] -> w548
                tunnel: w547 -> [_ w561]
                tunnel: w546 -> [w554 w560]
                tunnel: [w554 w559] -> w545
                frame 0, Default {
                  n212 = Replace Array Subset(array=w558, new element=w556, index=w557) -> (w555:T56[])
                }
                frame -1 {
                  n213 = call <vilib>:"Error Cluster From Error Code.vi"("error in (no error)"=w560, "error message (\"\")"=w561, "error code (0)"=7004) -> ("error out"=w559:errorcluster)  [unwired: 6 in]
                }
              }
            }
            frame True {
              n214 = Build Array (concatenate)(w569, w568) -> (w567:T56[])
            }
          }
          n215 = in-place-cluster #6("Main Config.DO Module Configs"=w537) -> (w525:T1)
        }
        n216 = call "Write to Log File.vi"("error in"=w527, "text"="Main: Commit Config (DO)") -> ()  [unwired: 9 in, 1 out]
      }
      frame "Commit Config (PR Module)" {
        # "Save Pressure Regulator Module Settings"
        n217 = Variant To Data(error in=w577, type=T61 {"GUID"="", "Drop Coords"={"Horizontal"=0, "Vertical"=0}, "Process Name"="", "Queue Name"="", "Settings"={"Cycle Period"=500.0, "PID 2 Parameters"={"Input Device"=enum."Default", "Output Device"=enum."Default", "Setpoint"=0.0, "PID gains"={"proportional gain (Kc)"=1.0, "integral time (Ti, min)"=0.01, "derivative time (Td, min)"=0.0}, "output range"={"output low"=0.0, "output high"=100.0}}, "Manual Entry"=0.0, "Auto?"=TRUE, "4-20mA Input Settings"={"Input Channel "=0}, "4-20mA Out Settings"={"Output DAQ Task"=""}, "Input Channel Tag Name "=""}, "Settings Load Count"=0} ("Feed Module Config"), Variant=w578) -> (data=w576:T61, error out=w575:errorcluster)
        n218 = in-place {
          in-place-border: w576 -> [w586]
          in-place-border: w575 -> [w582]
          in-place-border: [w581] -> w572
          n219 = in-place-cluster #7(w571) -> ("Main Config.PR Module Configs"=w580:T61[])
          n220 = Unbundle By Name(w586) -> ("GUID"=w583:string)
          n221 = Empty Array?(array=w580) -> (empty?=w587:bool)
          n222 = Format Into String(format string="Could not save Digital Out Module config. No matching GUID for \"%s\"." ("error message (\"\")"), w583) -> (resulting string=w584:string)  [unwired: 2 in, 1 out]
          n223 = case shown="True" w587 {
            tunnel: w583 -> [w595 _]
            tunnel: w580 -> [w593 w612]
            tunnel: w586 -> [w592 w609]
            tunnel: [w591 w611] -> w579
            tunnel: w584 -> [w590 _]
            tunnel: w582 -> [w589 w610]
            tunnel: [w588 w610] -> w581
            frame False {
              n224 = for {
                tunnel: w593 -> [w608] mode=indexing
                tunnel: [w607] -> w596 mode=indexing
                workers-P: _ -> [_]
                n225 = Unbundle By Name(w608) -> ("GUID"=w607:string)
              }
              n226 = Search 1D Array(1D array=w596, element=w595) -> (index of element=w594:i32)  [unwired: 1 in]
              n227 = case shown="-1" w594 {
                selector: w594 -> [w600 _]
                tunnel: w593 -> [w601 w606]
                tunnel: w592 -> [w599 _]
                tunnel: [w598 w606] -> w591
                tunnel: w590 -> [_ w604]
                tunnel: w589 -> [w597 w603]
                tunnel: [w597 w602] -> w588
                frame 0, Default {
                  n228 = Replace Array Subset(array=w601, new element=w599, index=w600) -> (w598:T61[])
                }
                frame -1 {
                  n229 = call <vilib>:"Error Cluster From Error Code.vi"("error in (no error)"=w603, "error message (\"\")"=w604, "error code (0)"=7004) -> ("error out"=w602:errorcluster)  [unwired: 6 in]
                }
              }
            }
            frame True {
              n230 = Build Array (concatenate)(w612, w609) -> (w611:T61[])
            }
          }
          n231 = in-place-cluster #7("Main Config.PR Module Configs"=w579) -> (w570:T1)
        }
        n232 = call "Write to Log File.vi"("error in"=w572, "text"="Main: Commit Config (PR Module)") -> ()  [unwired: 9 in, 1 out]
      }
      frame "Commit Config (TCU Module)" {
        # "Save Temperature Control Unit Module Settings"
        n233 = Variant To Data(error in=w620, type=T47 {"GUID"="", "Drop Coords"={"Horizontal"=0, "Vertical"=0}, "Process Name"="", "Queue Name"="", "Settings"={"Cycle Period"=500.0, "Setpoint Entry"=0.0, "Output Device"=enum."Default", "Huber Ministat 230 Settings"={"VISA resource name"="", "Simulated?"=FALSE}, "Lauda Settings"={"VISA resource name"="", "Simulated?"=FALSE, "Pump Power"=2}, "Julabo FP-50 Settings"={"VISA resource name"="", "Simulated?"=FALSE, "Pump Power"=2}, "Internal Control?"=FALSE, "Huber Unistat 410 Settings"={"VISA resource name"="", "Address"=0, "Simulated?"=FALSE}}, "Load Count"=0, "Power Level Changed"=FALSE} ("TCU Module Config"), Variant=w621) -> (data=w619:T47, error out=w618:errorcluster)
        n234 = in-place {
          in-place-border: w619 -> [w629]
          in-place-border: w618 -> [w625]
          in-place-border: [w624] -> w615
          n235 = in-place-cluster #8(w614) -> ("Main Config.TCU Module Configs"=w623:T47[])
          n236 = Unbundle By Name(w629) -> ("GUID"=w626:string)
          n237 = Empty Array?(array=w623) -> (empty?=w630:bool)
          n238 = Format Into String(format string="Could not save TCU Module config. No matching GUID for \"%s\"." ("error message (\"\")"), w626) -> (resulting string=w627:string)  [unwired: 2 in, 1 out]
          n239 = case shown="False" w630 {
            tunnel: w626 -> [w638 _]
            tunnel: w623 -> [w636 w655]
            tunnel: w629 -> [w635 w654]
            tunnel: [w634 w653] -> w622
            tunnel: w627 -> [w633 _]
            tunnel: w625 -> [w632 w652]
            tunnel: [w631 w652] -> w624
            frame False {
              n240 = for {
                tunnel: w636 -> [w651] mode=indexing
                tunnel: [w650] -> w639 mode=indexing
                workers-P: _ -> [_]
                n241 = Unbundle By Name(w651) -> ("GUID"=w650:string)
              }
              n242 = Search 1D Array(1D array=w639, element=w638) -> (index of element=w637:i32)  [unwired: 1 in]
              n243 = case shown="0, Default" w637 {
                selector: w637 -> [w643 _]
                tunnel: w636 -> [w644 w649]
                tunnel: w635 -> [w642 _]
                tunnel: [w641 w649] -> w634
                tunnel: w633 -> [_ w647]
                tunnel: w632 -> [w640 w646]
                tunnel: [w640 w645] -> w631
                frame 0, Default {
                  n244 = Replace Array Subset(array=w644, new element=w642, index=w643) -> (w641:T47[])
                }
                frame -1 {
                  n245 = call <vilib>:"Error Cluster From Error Code.vi"("error in (no error)"=w646, "error message (\"\")"=w647, "error code (0)"=7004) -> ("error out"=w645:errorcluster)  [unwired: 6 in]
                }
              }
            }
            frame True {
              n246 = Build Array (concatenate)(w655, w654) -> (w653:T47[])
            }
          }
          n247 = in-place-cluster #8("Main Config.TCU Module Configs"=w622) -> (w613:T1)
        }
        n248 = call "Write to Log File.vi"("error in"=w615, "text"="Main: Commit Config (TCU)") -> ()  [unwired: 9 in, 1 out]
      }
      frame "Commit Config (Scale Module)" {
        w660 = T39 {"GUID"="", "Drop Coords"={"Horizontal"=0, "Vertical"=0}, "Process Name"="", "Queue Name"="", "Settings"={"Cycle Period"=500.0, "Mettler"={"VISA resource name"="", "Simulated?"=FALSE}, "Scale Type"=""}, "Load Count"=0}  # Scale Module Config
        # "Save Scale Module Settings"
        n249 = Variant To Data(error in=w663, type=w660, Variant=w664) -> (data=w662:T39, error out=w661:errorcluster)
        n250 = in-place {
          in-place-border: w662 -> [w672]
          in-place-border: w661 -> [w668]
          in-place-border: [w667] -> w658
          n251 = in-place-cluster #9(w657) -> ("Main Config.Scale Module Configs"=w666:T39[])
          n252 = Unbundle By Name(w672) -> ("GUID"=w669:string)
          n253 = Empty Array?(array=w666) -> (empty?=w673:bool)
          n254 = Format Into String(format string="Could not save Scale Module config. No matching GUID for \"%s\"." ("error message (\"\")"), w669) -> (resulting string=w670:string)  [unwired: 2 in, 1 out]
          n255 = case shown="True" w673 {
            tunnel: w669 -> [w681 _]
            tunnel: w666 -> [w679 w698]
            tunnel: w672 -> [w678 w697]
            tunnel: [w677 w696] -> w665
            tunnel: w670 -> [w676 _]
            tunnel: w668 -> [w675 w695]
            tunnel: [w674 w695] -> w667
            frame False {
              n256 = for {
                tunnel: w679 -> [w694] mode=indexing
                tunnel: [w693] -> w682 mode=indexing
                workers-P: _ -> [_]
                n257 = Unbundle By Name(w694) -> ("GUID"=w693:string)
              }
              n258 = Search 1D Array(1D array=w682, element=w681) -> (index of element=w680:i32)  [unwired: 1 in]
              n259 = case shown="0, Default" w680 {
                selector: w680 -> [w686 _]
                tunnel: w679 -> [w687 w692]
                tunnel: w678 -> [w685 _]
                tunnel: [w684 w692] -> w677
                tunnel: w676 -> [_ w690]
                tunnel: w675 -> [w683 w689]
                tunnel: [w683 w688] -> w674
                frame 0, Default {
                  n260 = Replace Array Subset(array=w687, new element=w685, index=w686) -> (w684:T39[])
                }
                frame -1 {
                  n261 = call <vilib>:"Error Cluster From Error Code.vi"("error in (no error)"=w689, "error message (\"\")"=w690, "error code (0)"=7004) -> ("error out"=w688:errorcluster)  [unwired: 6 in]
                }
              }
            }
            frame True {
              n262 = Build Array (concatenate)(w698, w697) -> (w696:T39[])
            }
          }
          n263 = in-place-cluster #9("Main Config.Scale Module Configs"=w665) -> (w656:T1)
        }
        n264 = call "Write to Log File.vi"("error in"=w658, "text"="Main: Commit Config (Scale Module)") -> ()  [unwired: 9 in, 1 out]
      }
      frame "Commit Config (Flow Module)" {
        w703 = T45 {"GUID"="", "Drop Coords"={"Horizontal"=0, "Vertical"=0}, "Process Name"="", "Queue Name"="", "Settings"={"Cycle Period"=500.0, "Bronkhorst M13"={"VISA resource name"="", "Simulated?"=FALSE}, "Flow Meter Type"="", "Bronkhorst M14"={"VISA resource name"="", "Simulated?"=FALSE}}, "Load Count"=0}  # Flow Module Config
        # "Save Flow Module Settings"
        n265 = Variant To Data(error in=w706, type=w703, Variant=w707) -> (data=w705:T45, error out=w704:errorcluster)
        n266 = in-place {
          in-place-border: w705 -> [w715]
          in-place-border: w704 -> [w711]
          in-place-border: [w710] -> w701
          n267 = in-place-cluster #10(w700) -> ("Main Config.Flow Module Configs"=w708:T45[])
          n268 = Unbundle By Name(w715) -> ("GUID"=w712:string)
          n269 = Empty Array?(array=w708) -> (empty?=w716:bool)
          n270 = Format Into String(format string="Could not save Scale Module config. No matching GUID for \"%s\"." ("error message (\"\")"), w712) -> (resulting string=w713:string)  [unwired: 2 in, 1 out]
          n271 = case shown="True" w716 {
            tunnel: w712 -> [w724 _]
            tunnel: w708 -> [w722 w741]
            tunnel: w715 -> [w721 w740]
            tunnel: [w720 w739] -> w709
            tunnel: w713 -> [w719 _]
            tunnel: w711 -> [w718 w738]
            tunnel: [w717 w738] -> w710
            frame False {
              n272 = for {
                tunnel: w722 -> [w737] mode=indexing
                tunnel: [w736] -> w725 mode=indexing
                workers-P: _ -> [_]
                n273 = Unbundle By Name(w737) -> ("GUID"=w736:string)
              }
              n274 = Search 1D Array(1D array=w725, element=w724) -> (index of element=w723:i32)  [unwired: 1 in]
              n275 = case shown="0, Default" w723 {
                selector: w723 -> [w729 _]
                tunnel: w722 -> [w730 w735]
                tunnel: w721 -> [w728 _]
                tunnel: [w727 w735] -> w720
                tunnel: w719 -> [_ w733]
                tunnel: w718 -> [w726 w732]
                tunnel: [w726 w731] -> w717
                frame 0, Default {
                  n276 = Replace Array Subset(array=w730, new element=w728, index=w729) -> (w727:T45[])
                }
                frame -1 {
                  n277 = call <vilib>:"Error Cluster From Error Code.vi"("error in (no error)"=w732, "error message (\"\")"=w733, "error code (0)"=7004) -> ("error out"=w731:errorcluster)  [unwired: 6 in]
                }
              }
            }
            frame True {
              n278 = Build Array (concatenate)(w741, w740) -> (w739:T45[])
            }
          }
          n279 = in-place-cluster #10("Main Config.Flow Module Configs"=w709) -> (w699:T1)
        }
        n280 = call "Write to Log File.vi"("error in"=w701, "text"="Main: Commit Config (Flow Module)") -> ()  [unwired: 9 in, 1 out]
      }
      frame "Commit Config (TT)" {
        # "Save Temperature Transmitter Module Settings"
        n281 = Variant To Data(error in=w748, type=T34 {"GUID"="", "Drop Coords"={"Horizontal"=0, "Vertical"=0}, "Input Channel Tag Name "="", "Process Name"="", "Queue Name"="", "Input Channel Numeric Alarm Settings"=[]} ("TT Module Config"), Variant=w749) -> (data=w747:T34, error out=w746:errorcluster)
        n282 = in-place {
          in-place-border: w747 -> [w758]
          in-place-border: w746 -> [w754]
          in-place-border: [w753] -> w744
          n283 = in-place-cluster #11(w743) -> ("Main Config.TT Module Configs"=w751:T34[])
          n284 = Unbundle By Name(w758) -> ("GUID"=w755:string)
          n285 = Empty Array?(array=w751) -> (empty?=w759:bool)
          n286 = Format Into String(format string="Could not save TT Module config. No matching GUID for \"%s\"." ("error message (\"\")"), w755) -> (resulting string=w756:string)  [unwired: 2 in, 1 out]
          n287 = case shown="True" w759 {
            tunnel: w755 -> [w767 _]
            tunnel: w751 -> [w765 w784]
            tunnel: w758 -> [w764 w783]
            tunnel: [w763 w782] -> w752
            tunnel: w756 -> [w762 _]
            tunnel: w754 -> [w761 w781]
            tunnel: [w760 w781] -> w753
            frame False {
              n288 = for {
                tunnel: w765 -> [w780] mode=indexing
                tunnel: [w779] -> w768 mode=indexing
                workers-P: _ -> [_]
                n289 = Unbundle By Name(w780) -> ("GUID"=w779:string)
              }
              n290 = Search 1D Array(1D array=w768, element=w767) -> (index of element=w766:i32)  [unwired: 1 in]
              n291 = case shown="0, Default" w766 {
                selector: w766 -> [w772 _]
                tunnel: w765 -> [w773 w778]
                tunnel: w764 -> [w771 _]
                tunnel: [w770 w778] -> w763
                tunnel: w762 -> [_ w776]
                tunnel: w761 -> [w769 w775]
                tunnel: [w769 w774] -> w760
                frame 0, Default {
                  n292 = Replace Array Subset(array=w773, new element=w771, index=w772) -> (w770:T34[])
                }
                frame -1 {
                  n293 = call <vilib>:"Error Cluster From Error Code.vi"("error in (no error)"=w775, "error message (\"\")"=w776, "error code (0)"=7003) -> ("error out"=w774:errorcluster)  [unwired: 6 in]
                }
              }
            }
            frame True {
              n294 = Build Array (concatenate)(w784, w783) -> (w782:T34[])
            }
          }
          n295 = in-place-cluster #11("Main Config.TT Module Configs"=w752) -> (w742:T1)
        }
        n296 = call "Write to Log File.vi"("error in"=w744, "text"="Main: Commit Config (TT)") -> ()  [unwired: 9 in, 1 out]
      }
      frame "Commit Config (PT)" {
        # "Save Pressure Transmitter Module Settings"
        n297 = Variant To Data(error in=w791, type=T38 {"GUID"="", "Drop Coords"={"Horizontal"=0, "Vertical"=0}, "Input Channel Tag Name "="", "Process Name"="", "Queue Name"="", "Input Channel Numeric Alarm Settings"=[]} ("TT Module Config"), Variant=w792) -> (data=w790:T38, error out=w789:errorcluster)
        n298 = in-place {
          in-place-border: w790 -> [w801]
          in-place-border: w789 -> [w797]
          in-place-border: [w796] -> w787
          n299 = in-place-cluster #12(w786) -> ("Main Config.PT Module Configs"=w795:T38[])
          n300 = Unbundle By Name(w801) -> ("GUID"=w798:string)
          n301 = Empty Array?(array=w795) -> (empty?=w802:bool)
          n302 = Format Into String(format string="Could not save PT Module config. No matching GUID for \"%s\"." ("error message (\"\")"), w798) -> (resulting string=w799:string)  [unwired: 2 in, 1 out]
          n303 = case shown="True" w802 {
            tunnel: w798 -> [w810 _]
            tunnel: w795 -> [w808 w827]
            tunnel: w801 -> [w807 w826]
            tunnel: [w806 w825] -> w794
            tunnel: w799 -> [w805 _]
            tunnel: w797 -> [w804 w824]
            tunnel: [w803 w824] -> w796
            frame False {
              n304 = for {
                tunnel: w808 -> [w823] mode=indexing
                tunnel: [w822] -> w811 mode=indexing
                workers-P: _ -> [_]
                n305 = Unbundle By Name(w823) -> ("GUID"=w822:string)
              }
              n306 = Search 1D Array(1D array=w811, element=w810) -> (index of element=w809:i32)  [unwired: 1 in]
              n307 = case shown="0, Default" w809 {
                selector: w809 -> [w815 _]
                tunnel: w808 -> [w816 w821]
                tunnel: w807 -> [w814 _]
                tunnel: [w813 w821] -> w806
                tunnel: w805 -> [_ w819]
                tunnel: w804 -> [w812 w818]
                tunnel: [w812 w817] -> w803
                frame 0, Default {
                  n308 = Replace Array Subset(array=w816, new element=w814, index=w815) -> (w813:T38[])
                }
                frame -1 {
                  n309 = call <vilib>:"Error Cluster From Error Code.vi"("error in (no error)"=w818, "error message (\"\")"=w819, "error code (0)"=7005) -> ("error out"=w817:errorcluster)  [unwired: 6 in]
                }
              }
            }
            frame True {
              n310 = Build Array (concatenate)(w827, w826) -> (w825:T38[])
            }
          }
          n311 = in-place-cluster #12("Main Config.PT Module Configs"=w794) -> (w785:T1)
        }
        n312 = call "Write to Log File.vi"("error in"=w787, "text"="Main: Commit Config (PT)") -> ()  [unwired: 9 in, 1 out]
      }
      frame "Commit Config (U3)" {
        # "Save LabJack U3 Module Settings"
        n313 = Variant To Data(error in=w834, type=T43 {"GUID"="", "Drop Coords"={"Horizontal"=0, "Vertical"=0}, "AI Channel Number"=enum."Default", "Process Name"="", "Queue Name"="", "Input Channel Numeric Alarm Settings"=[]} ("TT Module Config"), Variant=w835) -> (data=w833:T43, error out=w832:errorcluster)
        n314 = in-place {
          in-place-border: w833 -> [w844]
          in-place-border: w832 -> [w840]
          in-place-border: [w839] -> w830
          n315 = in-place-cluster #13(w829) -> ("Main Config.U3 Module Configs"=w838:T43[])
          n316 = Unbundle By Name(w844) -> ("GUID"=w841:string)
          n317 = Empty Array?(array=w838) -> (empty?=w845:bool)
          n318 = Format Into String(format string="Could not save U3 Module config. No matching GUID for \"%s\"." ("error message (\"\")"), w841) -> (resulting string=w842:string)  [unwired: 2 in, 1 out]
          n319 = case shown="True" w845 {
            tunnel: w841 -> [w853 _]
            tunnel: w838 -> [w851 w870]
            tunnel: w844 -> [w850 w869]
            tunnel: [w849 w868] -> w837
            tunnel: w842 -> [w848 _]
            tunnel: w840 -> [w847 w867]
            tunnel: [w846 w867] -> w839
            frame False {
              n320 = for {
                tunnel: w851 -> [w866] mode=indexing
                tunnel: [w865] -> w854 mode=indexing
                workers-P: _ -> [_]
                n321 = Unbundle By Name(w866) -> ("GUID"=w865:string)
              }
              n322 = Search 1D Array(1D array=w854, element=w853) -> (index of element=w852:i32)  [unwired: 1 in]
              n323 = case shown="-1" w852 {
                selector: w852 -> [w858 _]
                tunnel: w851 -> [w859 w864]
                tunnel: w850 -> [w857 _]
                tunnel: [w856 w864] -> w849
                tunnel: w848 -> [_ w862]
                tunnel: w847 -> [w855 w861]
                tunnel: [w855 w860] -> w846
                frame 0, Default {
                  n324 = Replace Array Subset(array=w859, new element=w857, index=w858) -> (w856:T43[])
                }
                frame -1 {
                  n325 = call <vilib>:"Error Cluster From Error Code.vi"("error in (no error)"=w861, "error message (\"\")"=w862, "error code (0)"=7005) -> ("error out"=w860:errorcluster)  [unwired: 6 in]
                }
              }
            }
            frame True {
              n326 = Build Array (concatenate)(w870, w869) -> (w868:T43[])
            }
          }
          n327 = in-place-cluster #13("Main Config.U3 Module Configs"=w837) -> (w828:T1)
        }
        n328 = call "Write to Log File.vi"("error in"=w830, "text"="Main: Commit Config (U3)") -> ()  [unwired: 9 in, 1 out]
      }
      frame "Delete Module" {
        w881 = ""  # GUID
        # "This message is called when a user deletes a module from the canvas. The GUID for the module is passed here and we delete it from the list."
        n329 = Variant To Data(error in=w879, type=w881, Variant=w880) -> (data=w876:string, error out=w878:errorcluster)
        n330 = in-place {
          in-place-border: w878 -> [w886]
          in-place-border: w876 -> [w885]
          in-place-border: [w884] -> w873
          n331 = in-place-cluster #14(w872) -> ("Main Config"=w883:T7)
          n332 = call "Delete GUID Module.vi"("error in (no error)"=w886, "GUID"=w885, "Main Config in"=w883) -> ("error out"=w884:errorcluster, "Main Config out"=w882:T7)  [unwired: 7 in]
          n333 = in-place-cluster #14("Main Config"=w882) -> (w871:T1)
        }
        n334 = Concatenate Strings("Main: GUID " ("string"), w876, " Deleted" ("string")) -> (w877:string)
        n335 = call "Write to Log File.vi"("error in"=w873, "text"=w877) -> ()  [unwired: 9 in, 1 out]
      }
      frame "Update Config (DAQ)" {
        n336 = Unbundle By Name(w891) -> ("Main Config.DAQ Config"=w890:T36)
        n337 = call-poly "Enqueue Message.vi"("error in (no error)"=w889, "Message Data"=w890, "Message"="DAQ-Update Settings", "Message Queue"=w892) -> ("error out"=w887:errorcluster)  [unwired: 6 in, 1 out]
        n338 = call "Write to Log File.vi"("error in"=w887, "text"="Main: Update Config (DAQ)") -> ()  [unwired: 9 in, 1 out]
      }
      frame "Update Config (TT)" {
        # "Create TT Modules and \"drop\" them on the Picture Control and assign configs"
        n339 = Unbundle By Name(w900) -> ("Main Config.TT Module Configs"=w899:T34[])
        n340 = property class="VI"() -> ("Front Panel.Title"=w898:string)  [unwired: 2 in, 2 out]
        n341 = for {
          shift-right: [w917] -> w901
          shift-left: w900 -> [w916]
          tunnel: w899 -> [w913] mode=indexing
          tunnel: w898 -> [w910]
          tunnel: w897 -> [w908]
          shift-right: [w907] -> w894
          shift-left: w896 -> [w906]
          # "TT (Main).vit"
          n342 = vi-ref "TT (Main).vi"() -> (w905:refnum<vi>)
          n343 = Unbundle By Name(w913) -> ("Process Name"=w912:string, "Drop Coords"=w909:T10)
          n344 = To Variant(anything=w913) -> (Variant=w914:variant)
          n345 = property class="VI"(reference=w905) -> ("Path"=w904:path)  [unwired: 1 in, 2 out]
          n346 = Bundle By Name(cluster=T82 {"Module VI Filepath"=path "", "Process Name"="", "Main UI Message Queue"=refnum, "Drop Coords"={"Horizontal"=0, "Vertical"=0}, "Module Parameters"=variant, "Name of Parent Window"=""} ("Drop Parameters"), "Module VI Filepath"=w904, "Module Parameters"=w914, "Process Name"=w912, "Main UI Message Queue"=w908, "Drop Coords"=w909, "Name of Parent Window"=w910) -> (w911:T82)
          n347 = call "Next Instance Number.vi"("Module Type"=Module_Type_Enum."TT", "Operation"=Module_Instance_Number_Operation_Enum."Next Instance Number") -> ()  [unwired: 8 in, 2 out]
          n348 = call "Drop Start VI.vi"("error in (no error)"=w906, "Drop Parameters"=w911, "State in"=w916) -> ("error out"=w907:errorcluster, "State out"=w917:T1)  [unwired: 7 in]
        }
        n349 = call "Write to Log File.vi"("error in"=w894, "text"="Main: Update Config (TT)") -> ()  [unwired: 9 in, 1 out]
      }
      frame "Update Config (PT)" {
        # "Create PT Modules and \"drop\" them on the Picture Control and assign configs"
        n350 = Unbundle By Name(w924) -> ("Main Config.PT Module Configs"=w923:T38[])
        n351 = property class="VI"() -> ("Front Panel.Title"=w922:string)  [unwired: 2 in, 2 out]
        n352 = for {
          shift-right: [w941] -> w925
          shift-left: w924 -> [w940]
          tunnel: w923 -> [w937] mode=indexing
          tunnel: w922 -> [w934]
          tunnel: w921 -> [w932]
          shift-right: [w931] -> w918
          shift-left: w920 -> [w930]
          n353 = vi-ref "PT (Main).vi"() -> (w929:refnum<vi>)
          n354 = To Variant(anything=w937) -> (Variant=w938:variant)
          n355 = Unbundle By Name(w937) -> ("Process Name"=w936:string, "Drop Coords"=w933:T10)
          n356 = property class="VI"(reference=w929) -> ("Path"=w928:path)  [unwired: 1 in, 2 out]
          n357 = Bundle By Name(cluster=T82 {"Module VI Filepath"=path "", "Process Name"="", "Main UI Message Queue"=refnum, "Drop Coords"={"Horizontal"=0, "Vertical"=0}, "Module Parameters"=variant, "Name of Parent Window"=""} ("Drop Parameters"), "Module VI Filepath"=w928, "Module Parameters"=w938, "Process Name"=w936, "Main UI Message Queue"=w932, "Drop Coords"=w933, "Name of Parent Window"=w934) -> (w935:T82)
          n358 = call "Drop Start VI.vi"("error in (no error)"=w930, "Drop Parameters"=w935, "State in"=w940) -> ("error out"=w931:errorcluster, "State out"=w941:T1)  [unwired: 7 in]
          n359 = call "Next Instance Number.vi"("Module Type"=Module_Type_Enum."PT", "Operation"=Module_Instance_Number_Operation_Enum."Next Instance Number") -> ()  [unwired: 8 in, 2 out]
        }
        n360 = call "Write to Log File.vi"("error in"=w918, "text"="Main: Update Config (PT)") -> ()  [unwired: 9 in, 1 out]
      }
      frame "Update Config (U3)" {
        # "Create U3 Modules and \"drop\" them on the Picture Control and assign configs"
        n361 = Unbundle By Name(w948) -> ("Main Config.U3 Module Configs"=w947:T43[])
        n362 = property class="VI"() -> ("Front Panel.Title"=w946:string)  [unwired: 2 in, 2 out]
        n363 = for {
          shift-right: [w965] -> w949
          shift-left: w948 -> [w964]
          tunnel: w947 -> [w961] mode=indexing
          tunnel: w946 -> [w958]
          tunnel: w945 -> [w956]
          shift-right: [w955] -> w942
          shift-left: w944 -> [w954]
          n364 = vi-ref "U3 Module.lvlib:U3 (Main).vit"() -> (w953:refnum<vi>)
          n365 = Unbundle By Name(w961) -> ("Process Name"=w960:string, "Drop Coords"=w957:T10)
          n366 = To Variant(anything=w961) -> (Variant=w962:variant)
          n367 = property class="VI"(reference=w953) -> ("Path"=w952:path)  [unwired: 1 in, 2 out]
          n368 = Bundle By Name(cluster=T82 {"Module VI Filepath"=path "", "Process Name"="", "Main UI Message Queue"=refnum, "Drop Coords"={"Horizontal"=0, "Vertical"=0}, "Module Parameters"=variant, "Name of Parent Window"=""} ("Drop Parameters"), "Module VI Filepath"=w952, "Module Parameters"=w962, "Process Name"=w960, "Main UI Message Queue"=w956, "Drop Coords"=w957, "Name of Parent Window"=w958) -> (w959:T82)
          n369 = call "Drop Start VI.vi"("error in (no error)"=w954, "Drop Parameters"=w959, "State in"=w964) -> ("error out"=w955:errorcluster, "State out"=w965:T1)  [unwired: 7 in]
          n370 = call "Next Instance Number.vi"("Module Type"=Module_Type_Enum."U3", "Operation"=Module_Instance_Number_Operation_Enum."Next Instance Number") -> ()  [unwired: 8 in, 2 out]
        }
        n371 = call "Write to Log File.vi"("error in"=w942, "text"="Main: Update Config (U3)") -> ()  [unwired: 9 in, 1 out]
      }
      frame "Update Config (Feed)" {
        # "Create Feed Modules and \"drop\" them on the Picture Control and assign configs"
        n372 = Unbundle By Name(w972) -> ("Main Config.Feed Module Configs"=w971:T17[])
        n373 = property class="VI"() -> ("Front Panel.Title"=w970:string)  [unwired: 2 in, 2 out]
        n374 = for {
          shift-right: [w989] -> w973
          shift-left: w972 -> [w988]
          tunnel: w971 -> [w985] mode=indexing
          tunnel: w970 -> [w982]
          tunnel: w969 -> [w980]
          shift-right: [w979] -> w966
          shift-left: w968 -> [w978]
          # "Feed Module (Main.vit"
          n375 = vi-ref "Feed Module (Main).vi"() -> (w977:refnum<vi>)
          n376 = To Variant(anything=w985) -> (Variant=w986:variant)
          n377 = Unbundle By Name(w985) -> ("Process Name"=w984:string, "Drop Coords"=w981:T10)
          n378 = property class="VI"(reference=w977) -> ("Path"=w976:path)  [unwired: 1 in, 2 out]
          n379 = Bundle By Name(cluster=T82 {"Module VI Filepath"=path "", "Process Name"="", "Main UI Message Queue"=refnum, "Drop Coords"={"Horizontal"=0, "Vertical"=0}, "Module Parameters"=variant, "Name of Parent Window"=""} ("Drop Parameters"), "Module VI Filepath"=w976, "Module Parameters"=w986, "Process Name"=w984, "Main UI Message Queue"=w980, "Drop Coords"=w981, "Name of Parent Window"=w982) -> (w983:T82)
          n380 = call "Drop Start VI.vi"("error in (no error)"=w978, "Drop Parameters"=w983, "State in"=w988) -> ("error out"=w979:errorcluster, "State out"=w989:T1)  [unwired: 7 in]
          n381 = call "Next Instance Number.vi"("Module Type"=Module_Type_Enum."Feed", "Operation"=Module_Instance_Number_Operation_Enum."Next Instance Number") -> ()  [unwired: 8 in, 2 out]
        }
        n382 = call "Write to Log File.vi"("error in"=w966, "text"="Main: Update Config (Feed)") -> ()  [unwired: 9 in, 1 out]
      }
      frame "Update Config (OPC)" {
        # "Create Feed Modules and \"drop\" them on the Picture Control and assign configs"
        n383 = Unbundle By Name(w996) -> ("Main Config.OPC Module Configs"=w995:T8[])
        n384 = property class="VI"() -> ("Front Panel.Title"=w994:string)  [unwired: 2 in, 2 out]
        n385 = for {
          shift-right: [w1013] -> w997
          shift-left: w996 -> [w1012]
          tunnel: w995 -> [w1009] mode=indexing
          tunnel: w994 -> [w1006]
          tunnel: w993 -> [w1004]
          shift-right: [w1003] -> w990
          shift-left: w992 -> [w1002]
          # "OPC Module (Main).vit"
          n386 = vi-ref "OPC Main.vi"() -> (w1001:refnum<vi>)
          n387 = To Variant(anything=w1009) -> (Variant=w1010:variant)
          n388 = Unbundle By Name(w1009) -> ("Process Name"=w1008:string, "Drop Coords"=w1005:T10)
          n389 = property class="VI"(reference=w1001) -> ("Path"=w1000:path)  [unwired: 1 in, 2 out]
          n390 = Bundle By Name(cluster=T82 {"Module VI Filepath"=path "", "Process Name"="", "Main UI Message Queue"=refnum, "Drop Coords"={"Horizontal"=0, "Vertical"=0}, "Module Parameters"=variant, "Name of Parent Window"=""} ("Drop Parameters"), "Module VI Filepath"=w1000, "Module Parameters"=w1010, "Process Name"=w1008, "Main UI Message Queue"=w1004, "Drop Coords"=w1005, "Name of Parent Window"=w1006) -> (w1007:T82)
          n391 = call "Drop Start VI.vi"("error in (no error)"=w1002, "Drop Parameters"=w1007, "State in"=w1012) -> ("error out"=w1003:errorcluster, "State out"=w1013:T1)  [unwired: 7 in]
          n392 = call "Next Instance Number.vi"("Module Type"=Module_Type_Enum."OPC", "Operation"=Module_Instance_Number_Operation_Enum."Next Instance Number") -> ()  [unwired: 8 in, 2 out]
        }
        n393 = call "Write to Log File.vi"("error in"=w990, "text"="Main: Update Config (Feed)") -> ()  [unwired: 9 in, 1 out]
      }
      frame "Update Config (Pump)" {
        # "Create Pump Modules and \"drop\" them on the Picture Control and assign configs"
        n394 = Unbundle By Name(w1020) -> ("Main Config.Pump Module Configs"=w1019:T41[])
        n395 = property class="VI"() -> ("Front Panel.Title"=w1018:string)  [unwired: 2 in, 2 out]
        n396 = for {
          shift-right: [w1037] -> w1021
          shift-left: w1020 -> [w1036]
          tunnel: w1019 -> [w1033] mode=indexing
          tunnel: w1018 -> [w1030]
          tunnel: w1017 -> [w1028]
          shift-right: [w1027] -> w1014
          shift-left: w1016 -> [w1026]
          # "Pump Module (Main).vit"
          n397 = vi-ref "Pump Module (Main).vi"() -> (w1025:refnum<vi>)
          n398 = To Variant(anything=w1033) -> (Variant=w1034:variant)
          n399 = Unbundle By Name(w1033) -> ("Process Name"=w1032:string, "Drop Coords"=w1029:T10)
          n400 = property class="VI"(reference=w1025) -> ("Path"=w1024:path)  [unwired: 1 in, 2 out]
          n401 = Bundle By Name(cluster=T82 {"Module VI Filepath"=path "", "Process Name"="", "Main UI Message Queue"=refnum, "Drop Coords"={"Horizontal"=0, "Vertical"=0}, "Module Parameters"=variant, "Name of Parent Window"=""} ("Drop Parameters"), "Module VI Filepath"=w1024, "Module Parameters"=w1034, "Process Name"=w1032, "Main UI Message Queue"=w1028, "Drop Coords"=w1029, "Name of Parent Window"=w1030) -> (w1031:T82)
          n402 = call "Drop Start VI.vi"("error in (no error)"=w1026, "Drop Parameters"=w1031, "State in"=w1036) -> ("error out"=w1027:errorcluster, "State out"=w1037:T1)  [unwired: 7 in]
          n403 = call "Next Instance Number.vi"("Module Type"=Module_Type_Enum."Pump", "Operation"=Module_Instance_Number_Operation_Enum."Next Instance Number") -> ()  [unwired: 8 in, 2 out]
        }
        n404 = call "Write to Log File.vi"("error in"=w1014, "text"="Main: Update Config (Pump)") -> ()  [unwired: 9 in, 1 out]
      }
      frame "Update Config (DO)" {
        # "Create DO Modules and \"drop\" them on the Picture Control and assign configs"
        n405 = Unbundle By Name(w1044) -> ("Main Config.DO Module Configs"=w1043:T56[])
        n406 = property class="VI"() -> ("Front Panel.Title"=w1042:string)  [unwired: 2 in, 2 out]
        n407 = for {
          shift-right: [w1061] -> w1045
          shift-left: w1044 -> [w1060]
          tunnel: w1043 -> [w1057] mode=indexing
          tunnel: w1042 -> [w1054]
          tunnel: w1041 -> [w1052]
          shift-right: [w1051] -> w1038
          shift-left: w1040 -> [w1050]
          # "DO Module (Main).vit"
          n408 = disable-structure shown="Enabled" {
            disable-tunnel: [w1062 w1063] -> w1049
            frame Disabled {
              n409 = vi-ref "D-O Module.lvlib:D-O Module (Main).vi"() -> (w1062:refnum<vi>)
            }
            frame Enabled {
              n410 = vi-ref "D-O Module.lvlib:D-O Module (Main).vi"() -> (w1063:refnum<vi>)
            }
          }
          n411 = To Variant(anything=w1057) -> (Variant=w1058:variant)
          n412 = Unbundle By Name(w1057) -> ("Process Name"=w1056:string, "Drop Coords"=w1053:T10)
          n413 = property class="VI"(reference=w1049) -> ("Path"=w1048:path)  [unwired: 1 in, 2 out]
          n414 = Bundle By Name(cluster=T82 {"Module VI Filepath"=path "", "Process Name"="", "Main UI Message Queue"=refnum, "Drop Coords"={"Horizontal"=0, "Vertical"=0}, "Module Parameters"=variant, "Name of Parent Window"=""} ("Drop Parameters"), "Module VI Filepath"=w1048, "Module Parameters"=w1058, "Process Name"=w1056, "Main UI Message Queue"=w1052, "Drop Coords"=w1053, "Name of Parent Window"=w1054) -> (w1055:T82)
          n415 = call "Drop Start VI.vi"("error in (no error)"=w1050, "Drop Parameters"=w1055, "State in"=w1060) -> ("error out"=w1051:errorcluster, "State out"=w1061:T1)  [unwired: 7 in]
          n416 = call "Next Instance Number.vi"("Module Type"=Module_Type_Enum."Pump", "Operation"=Module_Instance_Number_Operation_Enum."Next Instance Number") -> ()  [unwired: 8 in, 2 out]
        }
        n417 = call "Write to Log File.vi"("error in"=w1038, "text"="Main: Update Config (DO)") -> ()  [unwired: 9 in, 1 out]
      }
      frame "Update Config (PR)" {
        # "Create Pressure Regulator Modules and \"drop\" them on the Picture Control and assign configs"
        n418 = Unbundle By Name(w1070) -> ("Main Config.PR Module Configs"=w1069:T61[])
        n419 = property class="VI"() -> ("Front Panel.Title"=w1068:string)  [unwired: 2 in, 2 out]
        n420 = for {
          shift-right: [w1087] -> w1071
          shift-left: w1070 -> [w1086]
          tunnel: w1069 -> [w1083] mode=indexing
          tunnel: w1068 -> [w1080]
          tunnel: w1067 -> [w1078]
          shift-right: [w1077] -> w1064
          shift-left: w1066 -> [w1076]
          # "PR Module (Main).vit"
          n421 = vi-ref "4-20mA Module (Main).vi"() -> (w1075:refnum<vi>)
          n422 = To Variant(anything=w1083) -> (Variant=w1084:variant)
          n423 = Unbundle By Name(w1083) -> ("Process Name"=w1082:string, "Drop Coords"=w1079:T10)
          n424 = property class="VI"(reference=w1075) -> ("Path"=w1074:path)  [unwired: 1 in, 2 out]
          n425 = Bundle By Name(cluster=T82 {"Module VI Filepath"=path "", "Process Name"="", "Main UI Message Queue"=refnum, "Drop Coords"={"Horizontal"=0, "Vertical"=0}, "Module Parameters"=variant, "Name of Parent Window"=""} ("Drop Parameters"), "Module VI Filepath"=w1074, "Module Parameters"=w1084, "Process Name"=w1082, "Main UI Message Queue"=w1078, "Drop Coords"=w1079, "Name of Parent Window"=w1080) -> (w1081:T82)
          n426 = call "Drop Start VI.vi"("error in (no error)"=w1076, "Drop Parameters"=w1081, "State in"=w1086) -> ("error out"=w1077:errorcluster, "State out"=w1087:T1)  [unwired: 7 in]
          n427 = call "Next Instance Number.vi"("Module Type"=Module_Type_Enum."Pump", "Operation"=Module_Instance_Number_Operation_Enum."Next Instance Number") -> ()  [unwired: 8 in, 2 out]
        }
        n428 = call "Write to Log File.vi"("error in"=w1064, "text"="Main: Update Config (PR)") -> ()  [unwired: 9 in, 1 out]
      }
      frame "Update Config (TCU)" {
        # "Create TCU Modules and \"drop\" them on the Picture Control and assign configs"
        n429 = Unbundle By Name(w1094) -> ("Main Config.TCU Module Configs"=w1093:T47[])
        n430 = property class="VI"() -> ("Front Panel.Title"=w1092:string)  [unwired: 2 in, 2 out]
        n431 = for {
          shift-right: [w1111] -> w1095
          shift-left: w1094 -> [w1110]
          tunnel: w1093 -> [w1107] mode=indexing
          tunnel: w1092 -> [w1104]
          tunnel: w1091 -> [w1102]
          shift-right: [w1101] -> w1088
          shift-left: w1090 -> [w1100]
          # "TCU Module (Main).vit"
          n432 = vi-ref "TCU Module.lvlib:TCU Module (Main).vi"() -> (w1099:refnum<vi>)
          n433 = To Variant(anything=w1107) -> (Variant=w1108:variant)
          n434 = Unbundle By Name(w1107) -> ("Process Name"=w1106:string, "Drop Coords"=w1103:T10)
          n435 = property class="VI"(reference=w1099) -> ("Path"=w1098:path)  [unwired: 1 in, 2 out]
          n436 = Bundle By Name(cluster=T82 {"Module VI Filepath"=path "", "Process Name"="", "Main UI Message Queue"=refnum, "Drop Coords"={"Horizontal"=0, "Vertical"=0}, "Module Parameters"=variant, "Name of Parent Window"=""} ("Drop Parameters"), "Module VI Filepath"=w1098, "Module Parameters"=w1108, "Process Name"=w1106, "Main UI Message Queue"=w1102, "Drop Coords"=w1103, "Name of Parent Window"=w1104) -> (w1105:T82)
          n437 = call "Drop Start VI.vi"("error in (no error)"=w1100, "Drop Parameters"=w1105, "State in"=w1110) -> ("error out"=w1101:errorcluster, "State out"=w1111:T1)  [unwired: 7 in]
          n438 = call "Next Instance Number.vi"("Module Type"=Module_Type_Enum."TCU", "Operation"=Module_Instance_Number_Operation_Enum."Next Instance Number") -> ()  [unwired: 8 in, 2 out]
        }
        n439 = call "Write to Log File.vi"("error in"=w1088, "text"="Main: Update Config (TCU)") -> ()  [unwired: 9 in, 1 out]
      }
      frame "Update Config (Scale)" {
        # "Create Scale Modules and \"drop\" them on the Picture Control and assign configs"
        n440 = Unbundle By Name(w1118) -> ("Main Config.Scale Module Configs"=w1117:T39[])
        n441 = property class="VI"() -> ("Front Panel.Title"=w1116:string)  [unwired: 2 in, 2 out]
        n442 = for {
          shift-right: [w1135] -> w1119
          shift-left: w1118 -> [w1134]
          tunnel: w1117 -> [w1131] mode=indexing
          tunnel: w1116 -> [w1128]
          tunnel: w1115 -> [w1126]
          shift-right: [w1125] -> w1112
          shift-left: w1114 -> [w1124]
          # "Scale Module (Main).vit"
          n443 = vi-ref "Scale Module (Main).vi"() -> (w1123:refnum<vi>)
          n444 = To Variant(anything=w1131) -> (Variant=w1132:variant)
          n445 = Unbundle By Name(w1131) -> ("Process Name"=w1130:string, "Drop Coords"=w1127:T10)
          n446 = property class="VI"(reference=w1123) -> ("Path"=w1122:path)  [unwired: 1 in, 2 out]
          n447 = Bundle By Name(cluster=T82 {"Module VI Filepath"=path "", "Process Name"="", "Main UI Message Queue"=refnum, "Drop Coords"={"Horizontal"=0, "Vertical"=0}, "Module Parameters"=variant, "Name of Parent Window"=""} ("Drop Parameters"), "Module VI Filepath"=w1122, "Module Parameters"=w1132, "Process Name"=w1130, "Main UI Message Queue"=w1126, "Drop Coords"=w1127, "Name of Parent Window"=w1128) -> (w1129:T82)
          n448 = call "Drop Start VI.vi"("error in (no error)"=w1124, "Drop Parameters"=w1129, "State in"=w1134) -> ("error out"=w1125:errorcluster, "State out"=w1135:T1)  [unwired: 7 in]
          n449 = call "Next Instance Number.vi"("Module Type"=Module_Type_Enum."Scale", "Operation"=Module_Instance_Number_Operation_Enum."Next Instance Number") -> ()  [unwired: 8 in, 2 out]
        }
        n450 = call "Write to Log File.vi"("error in"=w1112, "text"="Main: Update Config (Scale)") -> ()  [unwired: 9 in, 1 out]
      }
      frame "Update Config (Flow)" {
        # "Create Flow Modules and \"drop\" them on the Picture Control and assign configs"
        n451 = Unbundle By Name(w1142) -> ("Main Config.Flow Module Configs"=w1141:T45[])
        n452 = property class="VI"() -> ("Front Panel.Title"=w1140:string)  [unwired: 2 in, 2 out]
        n453 = for {
          shift-right: [w1159] -> w1143
          shift-left: w1142 -> [w1158]
          tunnel: w1141 -> [w1155] mode=indexing
          tunnel: w1140 -> [w1152]
          tunnel: w1139 -> [w1150]
          shift-right: [w1149] -> w1136
          shift-left: w1138 -> [w1148]
          # "Flow Module (Main).vit"
          n454 = vi-ref "Flow Module.lvlib:Flow Module (Main).vi"() -> (w1147:refnum<vi>)
          n455 = To Variant(anything=w1155) -> (Variant=w1156:variant)
          n456 = Unbundle By Name(w1155) -> ("Process Name"=w1154:string, "Drop Coords"=w1151:T10)
          n457 = property class="VI"(reference=w1147) -> ("Path"=w1146:path)  [unwired: 1 in, 2 out]
          n458 = Bundle By Name(cluster=T82 {"Module VI Filepath"=path "", "Process Name"="", "Main UI Message Queue"=refnum, "Drop Coords"={"Horizontal"=0, "Vertical"=0}, "Module Parameters"=variant, "Name of Parent Window"=""} ("Drop Parameters"), "Module VI Filepath"=w1146, "Module Parameters"=w1156, "Process Name"=w1154, "Main UI Message Queue"=w1150, "Drop Coords"=w1151, "Name of Parent Window"=w1152) -> (w1153:T82)
          n459 = call "Drop Start VI.vi"("error in (no error)"=w1148, "Drop Parameters"=w1153, "State in"=w1158) -> ("error out"=w1149:errorcluster, "State out"=w1159:T1)  [unwired: 7 in]
          n460 = call "Next Instance Number.vi"("Module Type"=Module_Type_Enum."Flow", "Operation"=Module_Instance_Number_Operation_Enum."Next Instance Number") -> ()  [unwired: 8 in, 2 out]
        }
        n461 = call "Write to Log File.vi"("error in"=w1136, "text"="Main: Update Config (Flow)") -> ()  [unwired: 9 in, 1 out]
      }
      frame "Update Config (Decoration)" {
        # "Display all decorations (e.g. arrows, lines) that are in the campaign. Get the image path for the decoration and raw them on the canvas."
        n462 = Unbundle By Name(w1163) -> ("Main Config.Decoration Module Configs"=w1164:T44[])
        n463 = property class="VI"() -> ("Front Panel.Title"=w1165:string)  [unwired: 2 in, 2 out]
        n464 = Current VI's Path() -> (path=w1166:path)
        n465 = call "Image Folder.vi"("Main VI path"=w1166) -> ("Image Folder path"=w1167:path)  [unwired: 10 in]
        n466 = for "For every decoration (e.g. arrows, lines)" {
          tunnel: w1164 -> [w1178] mode=indexing
          tunnel: w1165 -> [_]
          shift-right: [w1168] -> w1160
          shift-left: w1162 -> [w1168]
          tunnel: w1167 -> [w1171]
          # "Use relative path of\nthe image in case\nthe image folder has\nchanged."
          n467 = Unbundle By Name(w1178) -> ("Decoration Filepath"=w1172:path, "Drop Coords"=w1173:T10)
          n468 = Strip Path(path=w1172) -> (name=w1170:string)  [unwired: 1 out]
          n469 = Build Path(base path=w1171, name or relative path=w1170) -> (appended path=w1169:path)
          n470 = Unbundle By Name(w1173) -> ("Horizontal"=w1175:i32, "Vertical"=w1174:i32)
          n471 = local read "Canvas"() -> (w1177:picture)
          n472 = call "Draw BMP at Location.vi"("top"=w1174, "left"=w1175, "selected path"=w1169, "picture in"=w1177) -> ("picture out"=w1176:picture)  [unwired: 5 in, 2 out]
          n473 = local write "Canvas"(w1176) -> ()
        }
        n474 = call "Write to Log File.vi"("error in"=w1160, "text"="Main: Update Config (Decoration)") -> ()  [unwired: 9 in, 1 out]
      }
      frame "Drag Start" {
        n475 = Variant To Data(error in=w1193, type=T68 {"Mouse Position"={"X"=0, "Y"=0}, "Mouse Modifiers"={"Button Down"=FALSE, "Shift Mod"=FALSE, "Menu Mod"=FALSE, "Option Mod"=FALSE}} ("Mouse"), Variant=w1192) -> (data=w1187:T68, error out=w1191:errorcluster)
        n476 = Unbundle By Name(w1187) -> ("Mouse Position"=w1186:cluster{"X":i32, "Y":i32})
        n477 = Unbundle By Name(w1184) -> ("[Thumbnails]"=w1190:T2[])
        n478 = call "Which Thumbnail.vi"("error in (no error)"=w1191, "Coords"=w1186, "[Thumbnails]"=w1190) -> ("error out"=w1181:errorcluster, "Path"=→"Path":path, "index of element"=w1180:i32)  [unwired: 6 in]
        "index of element" <- w1180
        n479 = call "Palette Cursors.vi"("error in (no error)"=w1181, "Index"=w1180) -> ("error out"=w1182:errorcluster, "cursor ID"=w1183:refnum<k1>)  [unwired: 7 in, 1 out]
        n480 = Bundle By Name(cluster=w1184, "Drag Object Idx"=w1180) -> (w1185:T1)
        n481 = call-poly <vilib>:"Set Cursor.vi"("error in (no error)"=w1182, "cursor ID"=w1183) -> ("error out"=w1179:errorcluster)  [unwired: 8 in, 1 out]
      }
      frame "Drop" {
        (unwired) T68 {"Mouse Position"={"X"=0, "Y"=0}, "Mouse Modifiers"={"Button Down"=FALSE, "Shift Mod"=FALSE, "Menu Mod"=FALSE, "Option Mod"=FALSE}} ("Mouse")
        n482 = Variant To Data(error in=w1208, type=cluster{"Coords":T10, "Mouse":T68} {"Coords"={"Horizontal"=0, "Vertical"=0}, "Mouse"={"Mouse Position"={"X"=0, "Y"=0}, "Mouse Modifiers"={"Button Down"=FALSE, "Shift Mod"=FALSE, "Menu Mod"=FALSE, "Option Mod"=FALSE}}} ("output cluster"), Variant=w1210) -> (data=w1205:cluster{"Coords":T10, "Mouse":T68}, error out=w1209:errorcluster)
        n483 = Unbundle By Name(w1207) -> ("Drag Object Idx"=w1206:i32, "Drop Offset"=w1203:T6)
        n484 = Unbundle By Name(w1205) -> ("Mouse.Mouse Position"=w1204:cluster{"X":i32, "Y":i32})
        "Mouse Position" <- w1204
        n485 = case shown="Default" w1206 {
          selector: w1206 -> [_ w1220]
          tunnel: w1207 -> [w1213 w1218]
          tunnel: [w1213 w1223] -> w1195
          tunnel: [w1212 w1222] -> w1200
          tunnel: w1209 -> [w1212 w1221]
          tunnel: w1204 -> [_ w1217]
          tunnel: w1203 -> [_ _]
          tunnel: w1201 -> [_ w1216]
          tunnel: [T82 {"Module VI Filepath"=path "", "Process Name"="Error", "Main UI Message Queue"=refnum, "Drop Coords"={"Horizontal"=0, "Vertical"=0}, "Module Parameters"=variant, "Name of Parent Window"=""} ("Drop Parameters") w1214] -> w1194
          frame -1 {
          }
          frame Default {
            n486 = call "Thumbnail Path.vi"("Drag Object Idx"=w1220, "Cluster"=w1218) -> ("Module Type"=w1215:T80, "Thumbnail Path"=w1219:path)  [unwired: 8 in]
            n487 = case "Module Type?" shown="\"Feed\"..\"OPC\"" w1215 {
              selector: w1215 -> [_ w1237]
              tunnel: [w1227 w1246] -> w1223
              tunnel: [w1231 w1245] -> w1222
              tunnel: w1221 -> [w1231 w1242]
              tunnel: w1217 -> [w1229 w1241]
              tunnel: w1219 -> [w1226 _]
              tunnel: w1218 -> [w1228 w1239]
              tunnel: w1216 -> [w1225 w1240]
              tunnel: [T82 {"Module VI Filepath"=path "", "Process Name"="Error", "Main UI Message Queue"=refnum, "Drop Coords"={"Horizontal"=0, "Vertical"=0}, "Module Parameters"=variant, "Name of Parent Window"=""} ("Drop Parameters") w1236] -> w1214
              frame "<unknown module>" {
                # "Non functional module (i.e. decoration like an arrow or line) has been dropped\nby the user. Save the filepath of the image being drawn and the coordinates into the\ncampaign configuration so it can be saved and recalled later."
                n488 = property class="VI"() -> ("Front Panel.Title"=w1230:string)  [unwired: 2 in, 2 out]
                n489 = call "Drop Decoration Parameters.vi"("Main UI Message Queue"=w1225, "Mouse Position"=w1229, "Parent Window Title"=w1230, "Path to Decoration image"=w1226, "State in"=w1228) -> ("State out"=w1227:T1)  [unwired: 4 in, 2 out]
                n490 = local read "Canvas"() -> (w1235:picture)
                n491 = Unbundle By Name(w1229) -> ("X"=w1233:i32, "Y"=w1232:i32)
                n492 = call "Draw BMP at Location.vi"("top"=w1232, "left"=w1233, "selected path"=w1226, "picture in"=w1235) -> ("picture out"=w1234:picture)  [unwired: 5 in, 2 out]
                n493 = local write "Canvas"(w1234) -> ()
              }
              frame "Feed".."OPC" {
                n494 = property class="VI"() -> ("Front Panel.Title"=w1238:string)  [unwired: 2 in, 2 out]
                n495 = call "Drop Parameters.vi"("Main UI Message Queue"=w1240, "Mouse Position"=w1241, "error in (no error)"=w1242, "Parent Window Title"=w1238, "Module Type"=w1237, "State in"=w1239) -> ("error out"=w1243:errorcluster, "Drop Parameters"=w1236:T82, "State out"=w1244:T1)  [unwired: 3 in]
                n496 = call "Drop Start VI.vi"("error in (no error)"=w1243, "Drop Parameters"=w1236, "State in"=w1244) -> ("error out"=w1245:errorcluster, "State out"=w1246:T1)  [unwired: 7 in]
              }
            }
          }
        }
        n497 = Unbundle By Name(w1194) -> ("Process Name"=w1197:string)
        n498 = Concatenate Strings("Main: " ("string"), w1197, " Dropped" ("text")) -> (w1199:string)
        n499 = call "Write to Log File.vi"("error in"=w1200, "text"=w1199) -> ()  [unwired: 9 in, 1 out]
      }
      frame "E-Stop" {
        # "Stop the VI?"
        # "Tell all the modules to do E-Stop"
        n500 = call "E-Stop.vi"("State in"=w1252) -> ("error out"=w1250:errorcluster, "State out"=w1251:T1)  [unwired: 9 in]
        n501 = Merge Errors(w1250, w1249) -> (w1247:errorcluster)
        n502 = call "Write to Log File.vi"("error in"=w1247, "text"="Main: E-STOP Activated") -> ()  [unwired: 9 in, 1 out]
      }
      frame "Error" {
        w1263 = T86 1 items=["no dialog", "OK message", "continue or stop message", "OK message + warnings", "continue/stop + warnings"] ("type of dialog (OK msg:1)")
        # "Error - Check the error message data and respond accordingly. This message is sent by the \"Error Handler\" VIs at the end of each loop in this application."
        n503 = Variant To Data(type=errorcluster {"status"=FALSE, "code"=0, "source"=""} ("error out"), Variant=w1268) -> (data=w1262:errorcluster, error out=w1261:errorcluster)  [unwired: 1 in]
        n504 = Merge Errors(w1262, w1261) -> (w1260:errorcluster)
        "data" <- w1260
        n505 = call <vilib>:"General Error Handler.vi"("type of dialog (OK msg:1)"=w1263, "error in (no error)"=w1260) -> ("message"=w1254:string, "error out"=w1256:errorcluster)  [unwired: 9 in, 3 out]
        n506 = disable-structure shown="Enabled" {
          disable-tunnel: w1266 -> [w1272 _]
          disable-tunnel: [w1269 _] -> w1265
          disable-tunnel: w1256 -> [_ _]
          frame Disabled {
            n507 = call-poly "Enqueue Message.vi"("Priority Message? (F)"=TRUE, "Message"="Exit", "Message Queue"=w1272) -> ("error out"=w1269:errorcluster)  [unwired: 7 in, 1 out]
          }
          frame Enabled {
            # "If infinite error loop, slow it down\nso user can exit"
            n508 = Wait (ms)(milliseconds to wait=u32 2000) -> ()  [unwired: 1 out]
          }
        }
        n509 = Merge Errors(w1265, w1261) -> (w1259:errorcluster)
        n510 = call <vilib>:"Clear Errors.vi"("error in (no error)"=w1259) -> ("error out"=w1258:errorcluster)  [unwired: 5 in, 1 out]
        n511 = Concatenate Strings("Main: Error in Main: " ("text"), w1254) -> (w1255:string)
        n512 = call "Write to Log File.vi"("error in"=w1258, "text"=w1255) -> ()  [unwired: 9 in, 1 out]
        "Message Data" <- w1268
      }
      frame "Exit" {
        # "Stop and close the dynamically launched modules\n(e.g. Feed Modules)"
        # "Don't stop the VI quite yet. Wait for the DAQ to\nstop so we can delete the tags/shared variables."
        # "Exit - Fire the User Event to stop the Event Handling Loop.  Also send Exit messages to the Acquisition and Logging loops."
        n513 = call "Fire User Event - Stop.vi"("User Event - Stop"=w1297) -> ("error out"=w1274:errorcluster)  [unwired: 10 in]
        n514 = Unbundle By Name(w1296) -> ("Waveform Loop"=w1292:refnum<queue>, "CSV Log"=w1295:refnum<queue>, "TDMS Log"=w1294:refnum<queue>, "Graphs"=w1278:refnum<queue>[], "DAQ"=w1281:refnum<queue>, "Sequence"=w1277:refnum<queue>)
        n515 = call "Palette Cursors.vi"() -> ("error out"=w1289:errorcluster, "Cursor IDs out"=w1290:refnum<k1>[])  [unwired: 9 in, 1 out]
        n516 = for {
          tunnel: w1290 -> [w1303] mode=indexing
          shift-right: [w1300] -> w1288
          shift-left: w1289 -> [w1302]
          n517 = call <vilib>:"Destroy Cursor.vi"("cursor ID"=w1303, "error in (no error)"=w1302) -> ("error out"=w1301:errorcluster)  [unwired: 8 in]
          n518 = call <vilib>:"Clear Errors.vi"("error in (no error)"=w1301) -> ("error out"=w1300:errorcluster)  [unwired: 5 in, 1 out]
        }
        n519 = Build Array (concatenate)(w1292, w1295, w1294, w1278, w1277) -> (w1293:refnum<queue>[])
        n520 = for "stop and close support VIs" {
          tunnel: w1293 -> [w1308] mode=indexing
          tunnel: [w1306] -> w1287 mode=indexing
          tunnel: w1274 -> [w1304]
          n521 = call-poly "Enqueue Message.vi"("error in (no error)"=w1304, "Message"="Stop", "Message Queue"=w1308) -> ("error out"=w1305:errorcluster, "dup Message Queue"=w1309:refnum<queue>)  [unwired: 7 in]
          n522 = call-poly "Enqueue Message.vi"("error in (no error)"=w1305, "Message"="Exit", "Message Queue"=w1309) -> ("error out"=w1306:errorcluster)  [unwired: 7 in, 1 out]
        }
        n523 = call-poly "Enqueue Message.vi"("Priority Message? (F)"=TRUE, "Message"="DAQ-Exit", "Message Queue"=w1281) -> ("error out"=w1283:errorcluster)  [unwired: 7 in, 1 out]
        n524 = Merge Errors(w1274, w1287, w1283) -> (w1286:errorcluster)
        n525 = call "Close VIs.vi"("error in (no error)"=w1286, "State in"=w1284) -> ("error out"=w1279:errorcluster, "State out"=w1285:T1)  [unwired: 8 in]
        n526 = flat-sequence {
          tunnel: w1279 -> [_]
          frame #0 {
            n527 = call "Tag FGV.vi"("Operation"=Tag_FGV_Operation_Enum."Delete All Tags") -> ()  [unwired: 7 in, 8 out]
          }
        }
        n528 = Merge Errors(w1280, w1279, w1288) -> (w1275:errorcluster)
        n529 = call "Write to Log File.vi"("error in"=w1275, "text"="Main: Exited") -> ()  [unwired: 9 in, 1 out]
      }
      frame "File-Settings" {
        # "Get the Process Name from the settings dialog"
        n530 = call "File-Settings-Dialog.vi"("error in (no error)"=w1316) -> ("error out"=w1312:errorcluster, "Process Name Out"=w1314:string)  [unwired: 9 in]
        n531 = Bundle By Name(cluster=w1315, "Process Name"=w1314) -> (w1311:T1)
        n532 = call "Write to Log File.vi"("error in"=w1312, "text"="Main: File-Settings") -> ()  [unwired: 9 in, 1 out]
      }
      frame "Initialize" {
        (unwired) "Thumbnail (Feed Module).bmp" ("name or relative path")
        # "Initialize - Get configuration settings, then message the UI to initialize, and broadcast the settings to the other message loops."
        n533 = call "Empty Picture"() -> ("empty picture"=w1349:picture)
        n534 = local write "Canvas"(w1349) -> ()
        n535 = call-poly "Enqueue Message.vi"("error in (no error)"=w1328, "Message"="New Document", "Message Queue"=w1329) -> ("error out"=w1321:errorcluster)  [unwired: 7 in, 1 out]
        n536 = property on="Start Log" class="Bool"("DisabledEnum"=T77."Enabled" ("Disabled")) -> ()  [unwired: 2 in, 2 out]
        n537 = property on="Pause Log Button" class="Bool (strict)"("DisabledEnum"=T77."Disabled and Grayed Out" ("Disabled")) -> ()  [unwired: 2 in, 2 out]
        n538 = property on="Palette" class="Pict"("DisabledEnum"=T77."Enabled" ("Disabled")) -> ()  [unwired: 2 in, 2 out]
        n539 = property class="VI"() -> ("Front Panel.PanelBounds"=w1341:T4, "Front Panel.WinBounds"=w1340:T4)  [unwired: 2 in, 2 out]
        "Front Panel Window:Panel Bounds" <- w1341
        n540 = property class="VI"() -> ("Panel"=w1334:refnum<vi>)  [unwired: 2 in, 2 out]
        n541 = Current VI's Path() -> (path=w1353:path)
        n542 = property on="Canvas" class="Pict"() -> ("Position"=w1339:T6)  [unwired: 2 in, 2 out]
        "Position" <- w1339
        n543 = disable-structure shown="Default" {
          disable-tunnel: w1353 -> [w1357 _]
          disable-tunnel: [w1356 w1358] -> w1322
          frame condition #0 (active) {
            n544 = Strip Path(path=w1357) -> (stripped path=w1356:path)  [unwired: 1 out]
          }
          frame condition #1 {
            n545 = Default Directory() -> (w1358:path)
          }
        }
        n546 = property class="Pnl"(reference=w1334) -> ("Panes[]"=w1335:refnum<vi>[])  [unwired: 1 in, 2 out]
        n547 = call "Next Instance Number.vi"("Operation"=Module_Instance_Number_Operation_Enum."Init") -> ()  [unwired: 9 in, 2 out]
        n548 = Index Array(array=w1335) -> (element=w1336:refnum<vi>)  [unwired: 1 in]
        n549 = property class="Pane"(reference=w1336) -> ("Origin"=w1337:T67)  [unwired: 1 in, 2 out]
        "Origin" <- w1337
        n550 = Build Path(base path=w1322, name or relative path="Images") -> (appended path=w1354:path)
        n551 = Subtract(x=w1340, y=w1341) -> (x-y=w1342:T4)
        "x-y" <- w1342
        n552 = Negate(x=w1337) -> (-x=w1338:T67)
        n553 = call "Load Palette Images.vi"("Palette Image Folder"=w1354) -> ("error out"=w1326:errorcluster, "Cursor IDs"=w1325:refnum<k1>[], "[Thumbnails]"=w1350:T2[], "new picture"=→"Palette":picture)  [unwired: 7 in]
        n554 = Unbundle By Name(w1342) -> ("Top"=w1343:i16)
        n555 = Add(x=w1338, y=w1339) -> (x+y=w1346:T6)
        n556 = Unbundle By Name(w1346) -> ("Top"=w1344:i32)
        n557 = Negate(x=w1343) -> (-x=w1347:i16)
        n558 = Add(x=w1347, y=w1344) -> (x+y=w1345:i32)
        n559 = Bundle By Name(cluster=w1346, "Top"=w1345) -> (w1333:T6)
        "Drop Offset" <- w1333
        n560 = call "Palette Cursors.vi"("error in (no error)"=w1326, "Initialize"=TRUE, "Cursor IDs in"=w1325) -> ()  [unwired: 6 in, 3 out]
        n561 = Bundle By Name(cluster=w1317, "[Thumbnails]"=w1350, "Active Object"=-1, "Drop Offset"=w1333, "Main Config.Cycle Period"=1.0) -> (w1351:T1)
        n562 = call "Write to Log File.vi"("error in"=w1321, "text"="Main: Initialized") -> ("error out"=w1320:errorcluster)  [unwired: 9 in]
      }
      frame "New Document" {
        # "Start DAQ. Don't wait for Start Log"
        # "DAQ task is cleared here"
        # "Reset all the tags."
        # "Called from initialize at the start of a run"
        n563 = call "Tag FGV.vi"("Operation"=Tag_FGV_Operation_Enum."Read All Tags", "error in (no error)"=w1365) -> ("error out"=w1366:errorcluster)  [unwired: 6 in, 7 out]
        n564 = call "Empty Picture"() -> ("empty picture"=w1368:picture)
        n565 = call "Tag FGV.vi"("Operation"=Tag_FGV_Operation_Enum."Init", "error in (no error)"=w1366) -> ("error out"=w1370:errorcluster)  [unwired: 6 in, 7 out]
        n566 = local write "Canvas"(w1368) -> ()
        n567 = call-poly "Enqueue Message.vi"("error in (no error)"=w1370, "Message"="DAQ-Initialize", "Message Queue"=w1369) -> ("error out"=w1362:errorcluster, "dup Message Queue"=w1363:refnum<queue>)  [unwired: 7 in]
        n568 = call-poly "Enqueue Message.vi"("error in (no error)"=w1362, "Message"="DAQ-Start", "Message Queue"=w1363) -> ("error out"=w1360:errorcluster)  [unwired: 7 in, 1 out]
        n569 = call "Write to Log File.vi"("error in"=w1360, "text"="Main: New Document") -> ("error out"=w1359:errorcluster)  [unwired: 9 in]
      }
      frame "Open Campaign" {
        # "Choose a saved campaign to load"
        # "Load a Campaign from a previous save"
        n570 = Unbundle By Name(w1379) -> ("Main Config"=w1390:T7, "Campaign Filepath"=w1383:path)
        n571 = call "Application Data Folder.vi"() -> ("Campaign Folder"=w1382:path)  [unwired: 7 in, 4 out]
        n572 = Empty String/Path?(string/path=w1383) -> (empty?=w1384:bool)
        n573 = Select(t=w1382, s=w1384, f=w1383) -> (s? t:f=w1381:path)
        n574 = call "File Dialog3"("start path"=w1381, "prompt"="Open campaign", "error in"=w1389, "pattern (all files)"="*.cfg") -> ("selected path"=w1387:path, "cancelled"=w1388:bool, "error out"=w1378:errorcluster)  [unwired: 8 in, 1 out]
        n575 = call <vilib>:"Clear Errors.vi"("error in (no error)"=w1378) -> ("error out"=w1377:errorcluster)  [unwired: 5 in, 1 out]
        n576 = case shown="False" w1388 {
          tunnel: w1390 -> [w1401 _]
          tunnel: w1377 -> [w1395 w1419]
          tunnel: [w1408 w1419] -> w1374
          tunnel: w1387 -> [w1412 _]
          tunnel: w1379 -> [w1403 w1418]
          tunnel: [w1410 w1418] -> w1380
          tunnel: w1376 -> [w1406 _]
          tunnel: w1375 -> [w1394 _]
          frame False {
            # "After the DAQ has executed its configuration, it will call the next case,\ni.e. Open Campaign-DAQ Commited\"\nwhich queues additional messages."
            # "close previously\nopened dynamic VIs"
            n577 = call "Empty Picture"() -> ("empty picture"=w1398:picture)
            n578 = call-poly "Enqueue Message.vi"("error in (no error)"=w1395, "Message"="DAQ-Stop", "Message Queue"=w1394) -> ("error out"=w1396:errorcluster)  [unwired: 7 in, 1 out]
            n579 = local write "Canvas"(w1398) -> ()
            n580 = call "Close VIs.vi"("error in (no error)"=w1396, "State in"=w1403) -> ("error out"=w1400:errorcluster, "State out"=w1404:T1)  [unwired: 8 in]
            n581 = call <vilib>:"Clear Errors.vi"("error in (no error)"=w1400) -> ("error out"=w1399:errorcluster)  [unwired: 5 in, 1 out]
            n582 = call "Clear Dynamic Module Configs.vi"("Main Config in"=w1401) -> ("Main Config out"=w1402:T7)  [unwired: 8 in, 1 out]
            n583 = call "Read-Write Config File.vi"("configuration file path"=w1412, "Main Config in"=w1402, "Mode"=Config_File_Operation_Enum."Read", "error in"=w1399) -> ("Config File Path"=w1411:path, "Main Config out"=w1393:T7, "error out"=w1409:errorcluster)  [unwired: 4 in]
            n584 = Unbundle By Name(w1393) -> ("Notebook"=w1392:string, "Page"=w1391:string)
            n585 = Bundle By Name(cluster=w1404, "Campaign Filepath"=w1411, "Config Changed?"=FALSE, "Main Config"=w1393) -> (w1410:T1)
            n586 = for {
              tunnel: w1406 -> [w1415]
              shift-right: [w1416] -> w1408
              shift-left: w1409 -> [w1417]
              tunnel: string[] ["New Document", "Update Config (DAQ)"] -> [w1414] mode=indexing
              n587 = call-poly "Enqueue Message.vi"("error in (no error)"=w1417, "Message"=w1414, "Message Queue"=w1415) -> ("error out"=w1416:errorcluster)  [unwired: 7 in, 1 out]
            }
            n588 = property on="Notebook" class="Str"("Val(Sgnl)"=w1392) -> ()  [unwired: 2 in, 2 out]
            n589 = property on="Page" class="Str"("Val(Sgnl)"=w1391) -> ()  [unwired: 2 in, 2 out]
          }
          frame True {
          }
        }
      }
      frame "Open Campaign-DAQ Commited" {
        # "Wait for DAQ Message Loop to commit its tags/shared variables before starting up the dynamic modules so that the dynamic modules that bind to tags/shared variables in the DAQ task will not error."
        n590 = for {
          tunnel: w1424 -> [w1426]
          shift-right: [w1427] -> w1420
          shift-left: _ -> [w1428]
          tunnel: string[] ["Update Config (TT)", "Update Config (Feed)", "Update Config (PT)", "Update Config (Pump)", "Update Config (Scale)", "Update Config (Flow)", "Update Config (U3)", "Update Config (Decoration)", "Update Config (TCU)", "Update Config (DO)", "Update Config (PR)", "Update Config (OPC)"] -> [w1425] mode=indexing
          n591 = call-poly "Enqueue Message.vi"("error in (no error)"=w1428, "Message"=w1425, "Message Queue"=w1426) -> ("error out"=w1427:errorcluster)  [unwired: 7 in, 1 out]
        }
        n592 = call "Write to Log File.vi"("error in"=w1420, "text"="Main: Campaign Opened") -> ()  [unwired: 9 in, 1 out]
      }
      frame "Read Config" {
        n593 = call "Read Main Config File.vi"("error in (no error)"=w1434) -> ("Main Config out"=w1431:T7, "error out"=w1429:errorcluster)  [unwired: 7 in, 1 out]
        n594 = Bundle By Name(cluster=w1432, "Main Config"=w1431) -> (w1433:T1)
        n595 = call "Write to Log File.vi"("error in"=w1429, "text"="Main: Read Config Completed") -> ()  [unwired: 9 in, 1 out]
      }
      frame "Save Campaign", "Save Campaign As" {
        n596 = local read "Notebook"() -> (w1437:string)
        n597 = local read "Page"() -> (w1436:string)
        n598 = Bundle By Name(cluster=w1438, "Main Config.Notebook"=w1437, "Main Config.Page"=w1436) -> (w1435:T1)
        n599 = Equal?(x=w1445, y="Save Campaign As") -> (x = y?=w1443:bool)
        n600 = call "Application Data Folder.vi"() -> ("Campaign Folder"=w1452:path)  [unwired: 7 in, 4 out]
        n601 = Unbundle By Name(w1435) -> ("Main Config"=w1453:T7, "Campaign Filepath"=w1447:path)
        n602 = Empty String/Path?(string/path=w1447) -> (empty?=w1442:bool)
        n603 = Or(x=w1442, y=w1443) -> (x .or. y?=w1441:bool)
        n604 = case shown="True" w1441 {
          tunnel: w1452 -> [_ w1464]
          tunnel: w1451 -> [w1456 w1461]
          tunnel: [w1456 w1457] -> w1450
          tunnel: [FALSE ("cancelled") w1460] -> w1449
          tunnel: [w1454 w1459] -> w1448
          tunnel: w1447 -> [w1454 _]
          frame False {
          }
          frame True {
            # "Choose a file name to save"
            n605 = call "File Dialog2"("start path"=w1464, "prompt"="Save campaign as", "error in"=w1461, "pattern (all files)"="*.cfg") -> ("selected path"=w1459:path, "cancelled"=w1460:bool, "error out"=w1458:errorcluster)  [unwired: 8 in, 1 out]
            n606 = call <vilib>:"Clear Errors.vi"("error in (no error)"=w1458) -> ("error out"=w1457:errorcluster)  [unwired: 5 in, 1 out]
          }
        }
        n607 = case shown="False" w1449 {
          tunnel: w1453 -> [w1471 _]
          tunnel: w1450 -> [w1470 w1474]
          tunnel: [w1469 w1474] -> w1439
          tunnel: w1448 -> [w1468 _]
          tunnel: w1435 -> [w1467 w1473]
          tunnel: [w1465 w1473] -> w1446
          frame False {
            n608 = call "Read-Write Config File.vi"("configuration file path"=w1468, "Main Config in"=w1471, "Mode"=Config_File_Operation_Enum."Write", "error in"=w1470) -> ("Config File Path"=w1466:path, "error out"=w1469:errorcluster)  [unwired: 4 in, 1 out]
            n609 = Bundle By Name(cluster=w1467, "Campaign Filepath"=w1466) -> (w1465:T1)
          }
          frame True {
          }
        }
        n610 = call "Write to Log File.vi"("error in"=w1439, "text"="Main: Campaign Saved") -> ()  [unwired: 9 in, 1 out]
      }
      frame "Start Log" {
        w1483 = "Set Data Rate" ("item tag")
        # "The Cycle Rate cannot be changed mid run"
        # "Set up the alarms, create the data and graphing files, create the data tags, and start the logging"
        n611 = Unbundle By Name(w1476) -> ("Process Name"=w1505:string)
        n612 = Unbundle By Name(w1510) -> ("Waveform Loop"=w1494:refnum<queue>, "CSV Log"=w1487:refnum<queue>)
        n613 = Unbundle By Name(w1476) -> ("Queues"=w1493:refnum<queue>[])
        n614 = Empty String/Path?(string/path=w1505) -> (empty?=w1504:bool)
        n615 = case "Is there a process name" shown="True" w1504 {
          tunnel: [w1533 w1536] -> w1486
          tunnel: w1505 -> [w1533 _]
          frame False {
          }
          frame True {
            n616 = Empty String/Path?(string/path="Page") -> (empty?=w1534:bool)
            n617 = case shown="False" w1534 {
              tunnel: "Notebook" -> [w1542 w1545]
              tunnel: [w1539 w1543] -> w1536
              tunnel: "Page" -> [w1538 _]
              frame False {
                n618 = Concatenate Strings(w1542, " " ("string"), w1538, "" ("string")) -> (w1539:string)
              }
              frame True {
                n619 = Concatenate Strings(w1545, "" ("string")) -> (w1543:string)
              }
            }
          }
        }
        n620 = Unbundle By Name(w1476) -> ("Main Config.Cycle Period"=w1481:dbl)
        n621 = Max & Min(x=w1481, y=1.0) -> (max(x,y)=w1479:dbl)  [unwired: 1 out]
        n622 = call "Logfile Paths.vi"("File Name"=w1486) -> ("Alarm CSV Logfile path"=w1497:path, "TDMS Logfile path"=w1508:path, "CSV Logfile path"=w1506:path)  [unwired: 8 in]
        "CSV Log File" <- w1506
        n623 = call-poly "Enqueue Message.vi"("Message Data"=w1486, "Message"="Notebook", "Message Queue"=w1487) -> ()  [unwired: 7 in, 2 out]
        n624 = Bundle By Name(cluster=T84 {"dt (seconds)"=0.1, "CSV Logfile path"=path "", "TDMS Logfile path"=path ""} ("Start Params"), "dt (seconds)"=w1479, "CSV Logfile path"=w1506, "TDMS Logfile path"=w1508) -> (w1507:T84)
        n625 = call "Log Alarm FGV.vi"("error in (no error)"=w1500, "Path"=w1497, "Operation"=Alarm_Log_Operation_Enum."Create Log") -> ("error out"=w1498:errorcluster)  [unwired: 8 in]
        n626 = flat-sequence {
          tunnel: w1493 -> [w1512]
          tunnel: w1498 -> [w1511]
          tunnel: [w1513] -> w1496
          tunnel: w1496 -> [w1522]
          tunnel: [w1521] -> w1495
          tunnel: w1492 -> [w1523]
          tunnel: w1476 -> [w1520]
          tunnel: w1495 -> [w1526]
          tunnel: w1507 -> [w1532]
          tunnel: w1494 -> [w1530]
          tunnel: [w1524] -> w1489
          tunnel: w1476 -> [w1528]
          tunnel: w1491 -> [w1527]
          frame #0 {
            n627 = for {
              tunnel: w1512 -> [w1518] mode=indexing
              tunnel: w1511 -> [w1517]
              tunnel: [w1516] -> w1514 mode=indexing
              n628 = Wait (ms)(milliseconds to wait=u32 250) -> ()  [unwired: 1 out]
              n629 = call-poly "Enqueue Message.vi"("error in (no error)"=w1517, "Message"="Start Log", "Message Queue"=w1518) -> ("error out"=w1516:errorcluster)  [unwired: 7 in, 1 out]
            }
            n630 = Merge Errors(w1511, w1514) -> (w1513:errorcluster)
          }
          frame #1 {
            n631 = call "Check Module Tag Creation.vi"("error in (no error)"=w1522, "Cluster"=w1520, "UI"=w1523) -> ("error out"=w1521:errorcluster)  [unwired: 8 in]
          }
          frame #2 {
            n632 = call-poly "Enqueue Message.vi"("error in (no error)"=w1526, "Message Data"=w1528, "Message"="Log Settings", "Message Queue"=w1527) -> ("error out"=w1525:errorcluster)  [unwired: 6 in, 1 out]
            n633 = call-poly "Enqueue Message.vi"("error in (no error)"=w1525, "Message Data"=w1532, "Message"="Start", "Message Queue"=w1530) -> ("error out"=w1524:errorcluster)  [unwired: 6 in, 1 out]
          }
        }
        n634 = call-poly "Enqueue Message.vi"("Message Data"=w1476, "Message"="Start", "Message Queue"=w1477) -> ()  [unwired: 7 in, 2 out]
        n635 = property on="Palette" class="Pict"("DisabledEnum"=T77."Disabled and Grayed Out" ("Disabled")) -> ()  [unwired: 2 in, 2 out]
        n636 = property on="Pause Log Button" class="Bool (strict)"("DisabledEnum"=T77."Enabled" ("Disabled")) -> ()  [unwired: 2 in, 2 out]
        n637 = property on="Start Log" class="Bool"("DisabledEnum"=T77."Disabled and Grayed Out" ("Disabled")) -> ()  [unwired: 2 in, 2 out]
        n638 = Current VI's Menubar() -> (w1484:refnum<k9>)
        n639 = call "Tag FGV.vi"("Operation"=Tag_FGV_Operation_Enum."Enable All Alarms", "error in (no error)"=w1489) -> ("error out"=w1478:errorcluster)  [unwired: 6 in, 7 out]
        n640 = Set Menu Item Info(7:w1483, 9:FALSE ("enabled"), 10:w1483, 11:w1484) -> ()  [unwired: 3 in, 2 out]
        n641 = call "Write to Log File.vi"("error in"=w1478, "text"="Main: Data Log Started") -> ()  [unwired: 9 in, 1 out]
      }
      frame "Stop Log" {
        # "Stop Waveform loop,\nwhich stops the\nCSV Log and\nTDMS Log."
        # "Stop the logging"
        n642 = Unbundle By Name(w1557) -> ("Waveform Loop"=w1556:refnum<queue>)
        n643 = property on="Palette" class="Pict"("DisabledEnum"=T77."Enabled" ("Disabled")) -> ()  [unwired: 2 in, 2 out]
        n644 = call-poly "Enqueue Message.vi"("error in (no error)"=w1554, "Message"="Stop", "Message Queue"=w1556) -> ("error out"=w1552:errorcluster)  [unwired: 7 in, 1 out]
        n645 = property on="Start Log" class="Bool"("DisabledEnum"=T77."Enabled" ("Disabled")) -> ()  [unwired: 2 in, 2 out]
        n646 = property on="Pause Log Button" class="Bool (strict)"("DisabledEnum"=T77."Disabled and Grayed Out" ("Disabled")) -> ()  [unwired: 2 in, 2 out]
        n647 = call "Log Alarm FGV.vi"("error in (no error)"=w1552, "Operation"=Alarm_Log_Operation_Enum."Close Log") -> ("error out"=w1546:errorcluster)  [unwired: 9 in]
        n648 = call "Write to Log File.vi"("error in"=w1546, "text"="Main: Data Log Stopped") -> ()  [unwired: 9 in, 1 out]
      }
      frame "Timeout" {
        # "Prevent CPU from overloading in the case that this is called too often."
        n649 = Wait (ms)(milliseconds to wait=u32 5) -> ()  [unwired: 1 out]
      }
      frame "Launch Sequence Dialog" {
        # "Control the execution of the Sequencer"
        n650 = call "Sequence Dialog.vi"("error in (no error)"=w1572, "Sequence UI"=w1561, "State Cluster In"=w1565) -> ("error out"=w1568:errorcluster, "Start"=w1566:bool, "cancelled"=w1571:bool, "State Cluster Out"=w1570:T1, "Pause"=w1564:bool)  [unwired: 3 in, 1 out]
        n651 = case "Is it Cancelled?" shown="False" w1571 {
          tunnel: w1570 -> [w1579 _]
          tunnel: [w1579 w1599] -> w1569
          tunnel: w1568 -> [w1583 w1600]
          tunnel: w1567 -> [w1581 _]
          tunnel: [w1573 w1600] -> w1562
          tunnel: w1566 -> [w1580 _]
          tunnel: w1565 -> [_ w1599]
          tunnel: w1564 -> [w1578 _]
          frame False {
            n652 = call-poly "Enqueue Message.vi"("error in (no error)"=w1583, "Message Data"=w1579, "Message"="Update Sequence", "Message Queue"=w1581) -> ("error out"=w1574:errorcluster, "dup Message Queue"=w1575:refnum<queue>)  [unwired: 6 in]
            n653 = case "Is it Paused?" shown="True" w1578 {
              tunnel: w1574 -> [w1587 w1593]
              tunnel: [w1586 w1592] -> w1577
              tunnel: w1575 -> [w1585 w1591]
              tunnel: [w1584 w1589] -> w1576
              frame False {
                n654 = call-poly "Enqueue Message.vi"("error in (no error)"=w1587, "Message"="Resume Sequence", "Message Queue"=w1585) -> ("error out"=w1586:errorcluster, "dup Message Queue"=w1584:refnum<queue>)  [unwired: 7 in]
              }
              frame True {
                n655 = call-poly "Enqueue Message.vi"("error in (no error)"=w1593, "Message"="Pause Sequence", "Message Queue"=w1591) -> ("error out"=w1592:errorcluster, "dup Message Queue"=w1589:refnum<queue>)  [unwired: 7 in]
              }
            }
            n656 = case "Start?" shown="True" w1580 {
              tunnel: w1577 -> [w1594 w1598]
              tunnel: [w1594 w1597] -> w1573
              tunnel: w1576 -> [_ w1596]
              frame False {
              }
              frame True {
                n657 = call-poly "Enqueue Message.vi"("error in (no error)"=w1598, "Message"="Start Sequence", "Message Queue"=w1596) -> ("error out"=w1597:errorcluster)  [unwired: 7 in, 1 out]
              }
            }
          }
          frame True {
          }
        }
        n658 = call "Write to Log File.vi"("error in"=w1562, "text"="Main: Sequencer Opened") -> ()  [unwired: 9 in, 1 out]
      }
      frame "Launch Data Rate Dialog" {
        # "Control the execution of the Sequencer"
        n659 = call "Data Rate Dialog.vi"("error in (no error)"=w1604, 11:w1601) -> ("error out"=w1603:errorcluster, 3:w1602:T1)  [unwired: 8 in]
        n660 = call "Write to Log File.vi"("error in"=w1603, "text"="Main: Data Rate Dialog Opened") -> ()  [unwired: 9 in, 1 out]
      }
      frame "Launch Calibration Dialog" {
        # "Run the Calibration Program"
        n661 = call "Calibration Main.vi"("error in (no error)"=w1610, "Pump Calibration Config in"=T85 {"Settings"={"Cycle Period"=500.0, "Ismatech"={"VISA resource name"="", "Simulated?"=TRUE, "Pump Number"=1.0, "Reverse?"=FALSE}, "Masterflex"={"VISA resource name"="", "Simulated?"=TRUE, "Pump Number"=1.0, "Reverse?"=FALSE}, "Bronkhorst M13 Flow Meter"={"VISA resource name"="", "Simulated?"=TRUE}, "PID 2 Parameters"={"Input Device"=enum."Default", "Output Device"=enum."Default"}, "Bronkhorst M14"={"VISA resource name"="", "Simulated?"=FALSE}, "Tacmina Settings"={"Analog DAQ Task"="", "Digital DAQ Task"=""}, "KNF SIMDOS Settings"={"VISA resource name"="", "Simulated?"=TRUE}, "VICI M50 Settings"={"VISA resource name"="", "Simulated?"=TRUE, "Pump Letter"="", "Reverse?"=FALSE}, "FLOM Settings"={"VISA resource name"="", "Simulated?"=TRUE, "Pump Number"=0.0}, "Calibration Limits"={"Minimum (ml/min)"=0.0, "Maximum (ml/min)"=0.0, "Steps"=0.0}, "SSI PR Settings"={"VISA resource name"="", "Simulated?"=FALSE}}, "Flowmeter Output"=0.0, "Density"=0.0, "FL Temp"=0.0, "Speed %"=0.0, "File Refnum"=refnum, "Pump On?"=enum."Not Initialized"}) -> ("error out"=w1609:errorcluster)  [unwired: 8 in, 1 out]
        n662 = call "Write to Log File.vi"("error in"=w1609, "text"="Main: Calibration Opened") -> ("error out"=w1608:errorcluster)  [unwired: 9 in]
      }
      frame "Launch Note Dialog" {
        # "Open the dialog for adding notes to the data file"
        n663 = call-poly "Enqueue Message.vi"("error in (no error)"=w1616, "Message"="Add Note", "Message Queue"=w1617) -> ("error out"=w1612:errorcluster)  [unwired: 7 in, 1 out]
        n664 = call "Write to Log File.vi"("error in"=w1612, "text"="Main: Note Dialog Opened") -> ()  [unwired: 9 in, 1 out]
      }
      frame Default {
        # "'Default' case only runs if there is a message that isn't defined in any of the other cases.  Output a programming error."
        n665 = Concatenate Strings("The invalid message string " ("string"), w1619, " was received in Main." ("string")) -> (w1620:string)
        n666 = Bundle By Name(cluster=errorcluster {"status"=TRUE, "code"=1, "source"=""} ("error constant"), "source"=w1620) -> (w1618:errorcluster)
        n667 = call <vilib>:"General Error Handler.vi"("error in (no error)"=w1618) -> ("message"=w1624:string)  [unwired: 10 in, 4 out]
        n668 = Concatenate Strings("Main: Note Dialog Opened" ("text"), w1624) -> (w1625:string)
        n669 = call "Write to Log File.vi"("text"=w1625) -> ()  [unwired: 10 in, 1 out]
      }
      frame "Tags Created" {
        n670 = call "Write to Log File.vi"("error in"=w1628, "text"="Main: Tags Created") -> ()  [unwired: 9 in, 1 out]
      }
    }
    "Cluster" <- w357
    n671 = call "Error Handler - Message Handling Loop.vi"("error in (no error)"=w363, "Message Queue"=w361) -> ("dup error in"=w362:errorcluster, "dup Message Queue"=w355:refnum<queue>)  [unwired: 8 in]
  }
  n672 = Build Path(base path=w66, name or relative path="History Graph Message Loop.vi") -> (appended path=w65:path)
  n673 = Open VI Reference(vi path=w65) -> (vi reference=w72:refnum<vi>, error out=w70:errorcluster)  [unwired: 5 in]
  n674 = invoke class="VI" method="Ctrl Val.Set"(reference=w72, error in=w70, "Control Name"="Message Queues", "Value"=w29) -> (reference out=w71:refnum<vi>, error out=w69:errorcluster)  [unwired: 1 in, 3 out]
  n675 = invoke class="VI" method="Run VI"(reference=w71, error in=w69, "Wait until done"=FALSE ("Wait Until Done"), "Auto Dispose Ref"=FALSE ("Auto Dispose Reference")) -> (reference out=w74:refnum<vi>)  [unwired: 1 in, 4 out]
  n676 = invoke on="Sub Panel" class="SubPnl" method="Insert VI"("VI Ref"=w74) -> (error out=→"error out":errorcluster)  [unwired: 3 in, 3 out]
  n677 = Unregister For Events(event registration refnum=w83, error in=w86) -> (error out=w53:errorcluster)
  n678 = disable-structure shown="Enabled" {
    frame Disabled {
      n679 = call "Feed Module (Main).vi"() -> ()  [unwired: 12 in]
      n680 = call "Tag FGV.vi"() -> ()  [unwired: 6 in, 6 out]
      n681 = call "TT (Main).vi"() -> ()  [unwired: 12 in]
      n682 = call "PT (Main).vi"() -> ()  [unwired: 12 in]
      n683 = call "History Graph Message Loop.vi"() -> ()  [unwired: 11 in, 1 out]
      n684 = call "Scale Module (Main).vi"() -> ()  [unwired: 12 in]
      n685 = call "Log Alarm FGV.vi"() -> ()  [unwired: 11 in, 1 out]
      n686 = call "Pump Module (Main).vi"() -> ()  [unwired: 12 in]
    }
    frame Enabled {
    }
  }
  n687 = Generate User Event(user event=w51, event data cluster=w50, error in=w53) -> (error out=w56:errorcluster)  [unwired: 1 in, 1 out]
  n688 = invoke class="VI (strict)" method="FP.Close"(reference=w52, error in=w56) -> (error out=w55:errorcluster)  [unwired: 1 in, 2 out]
  n689 = call <vilib>:"Clear Errors.vi"("error in (no error)"=w55) -> ("error out"=w54:errorcluster)  [unwired: 5 in, 1 out]
  n690 = Close Reference(reference=w52, error in (no error)=w54) -> ()  [unwired: 1 out]
  n691 = Merge Errors(w53, w87, w36, w35, w34, w33, w32) -> (w85:errorcluster)
  n692 = call "Destroy User Event - Stop.vi"("error in (no error)"=w85, "User Event - Stop"=w84) -> ("error out"=w38:errorcluster)  [unwired: 9 in]
  n693 = call "Close File.vi"("error in"=w38) -> ("error out"=w12:errorcluster)  [unwired: 10 in]
  n694 = Release Queue(queue=w13, error in (no error)=w12) -> (error out=w11:errorcluster)  [unwired: 1 in, 2 out]
  n695 = Release Queue(queue=w14, error in (no error)=w11) -> (error out=w10:errorcluster)  [unwired: 1 in, 2 out]
  n696 = Release Queue(queue=w15, error in (no error)=w10) -> (error out=w9:errorcluster)  [unwired: 1 in, 2 out]
  n697 = for {
    tunnel: w16 -> [w1633] mode=indexing
    tunnel: w9 -> [w1632]
    tunnel: [w1631] -> _ mode=indexing
    tunnel: [w1631] -> w8
    n698 = Release Queue(queue=w1633, error in (no error)=w1632) -> (error out=w1631:errorcluster)  [unwired: 1 in, 2 out]
  }
  n699 = Merge Errors(w8) -> (w7:errorcluster)
  n700 = Release Queue(queue=w17, error in (no error)=w7) -> (error out=w6:errorcluster)  [unwired: 1 in, 2 out]
  n701 = Release Queue(queue=w18, error in (no error)=w6) -> (error out=w5:errorcluster)  [unwired: 1 in, 2 out]
  n702 = Release Queue(queue=w26, error in (no error)=w5) -> (error out=w4:errorcluster)  [unwired: 1 in, 2 out]
  n703 = Release Queue(queue=w27, error in (no error)=w4) -> (error out=w3:errorcluster)  [unwired: 1 in, 2 out]
  n704 = Release Queue(queue=w25, error in (no error)=w3) -> (error out=w2:errorcluster)  [unwired: 1 in, 2 out]
  n705 = Release Queue(queue=w28, error in (no error)=w2) -> (error out=w1:errorcluster)  [unwired: 1 in, 2 out]
  n706 = disable-structure shown="RUN_TIME_ENGINE==True" {
    disable-tunnel: w1 -> [_ _]
    frame condition #0 {
      # "Call Quit LabVIEW if running as a built application."
      n707 = Quit LabVIEW() -> ()  [unwired: 1 in]
    }
    frame condition #1 (active) {
    }
  }
